vi "mainDebug.vi"() -> ()   [LabVIEW 2024]
doc: "Main VI for FLS imaging system."
uses:
  SubVI/DigitizerConfiguration/FLImDAQ.ctl
  <instrlib>/niScope/Controls/niScope trigger source.ctl
  SubVI/LabJack/LJ Pin Setting.ctl
  ConfigFiles/AimingBeamVideoConfig.ctl
  <vilib>/Utility/error.llb/DialogType.ctl
  SubVI/GlobalVariables.vi
  <vilib>/Instr/_visa.llb/VISA Configure Serial Port (Instr).vi
  <userlib>/_OpenG.lib/file/file.llb/openg_file.lvlib
  <userlib>/_OpenG.lib/time/time.llb/openg_time.lvlib
  <vilib>/Utility/miscctls.llb/LVPointTypeDef.ctl
panel:
  out "TCP wait time(ms)":u32
  in  "error (stop LT loop)":errorcluster
  out "Dummy LT Waveform":dbl(graph)
  in  "DeconChannel":i8=1 min=1 max=3 step=1
  out "Visualization PC video source":T1
  in  "Video Display":bool
  out "ML?":bool
  out "Sync Success?":bool
  out "Disclamer":picture
  out "Calibration #":i8
  out "BG #":i8
  in  "TCP Connect":bool
  out "Help":string
  in  "355nm Laser toggle":bool caption="355nm 460Hz"
  in  "Aiming beam toggle":bool caption="445nm 15Hz 15mA"
  out "Run #":i8
  in  "StopButton":bool caption="Stop"
  out "Aquisition Status:":bool
  in  "StartButton":bool caption="Start"
  in  "Video Source":enum32{"Camera", "FrameGrabber"}(radio)
  out "Case #":string
  out "System Hardware Connection Status":T2
  in  "Tab Control":T3(tab)
  out "Communication loop(ms)":u32
  out "laser EM lamp V":dbl format="%0.6f"
  in  "Show BG":bool
  out "LJ Pinout":T4={"Ch1 Bias"="DAC0", "Ch2 Bias"="DAC1", "Ch3 Bias"="DAC2", "Ch4 Bias"="DAC0", "355 PWM"="FIO0", "AimingBeam PWM"="FIO2", "Laser Ready"="FIO3", "Interlock"="FIO1", "Laser Start/Stop"="FIO1", "Red LED"="FIO1", "Green LED"="DIO3", "Foot Pedal"="DIO15"}
  out "FLImDAQ":T5={"Digitizer 1"="", "Digitizer 2"="", "Channel"=enum."Channel 0", "trigger source"="VAL_EXTERNAL", "trigger level"=0.5, "trigger delay"=1.35e-07, "min sample rate"=12500000000.0, "min record length"=2500, "vertical range"=1.0, "vertical offset"=-0.25, "Waveform to Avg"=2000} caption="FLIm DAQ Configuration" {"trigger delay" format="%^#.4e"; "trigger level" min=0.0 max=3.5 step=0.5 format="%.2f"; "vertical offset" format="%.4f"; "vertical range" format="%.2f"; "min sample rate" format="%#.2p"}
  in  "Sys Reconfig":bool
  out "data out(communcation loop)":string
  out "Laser Rep Rate":dbl
  out "State log":string
  in  "Quit":bool
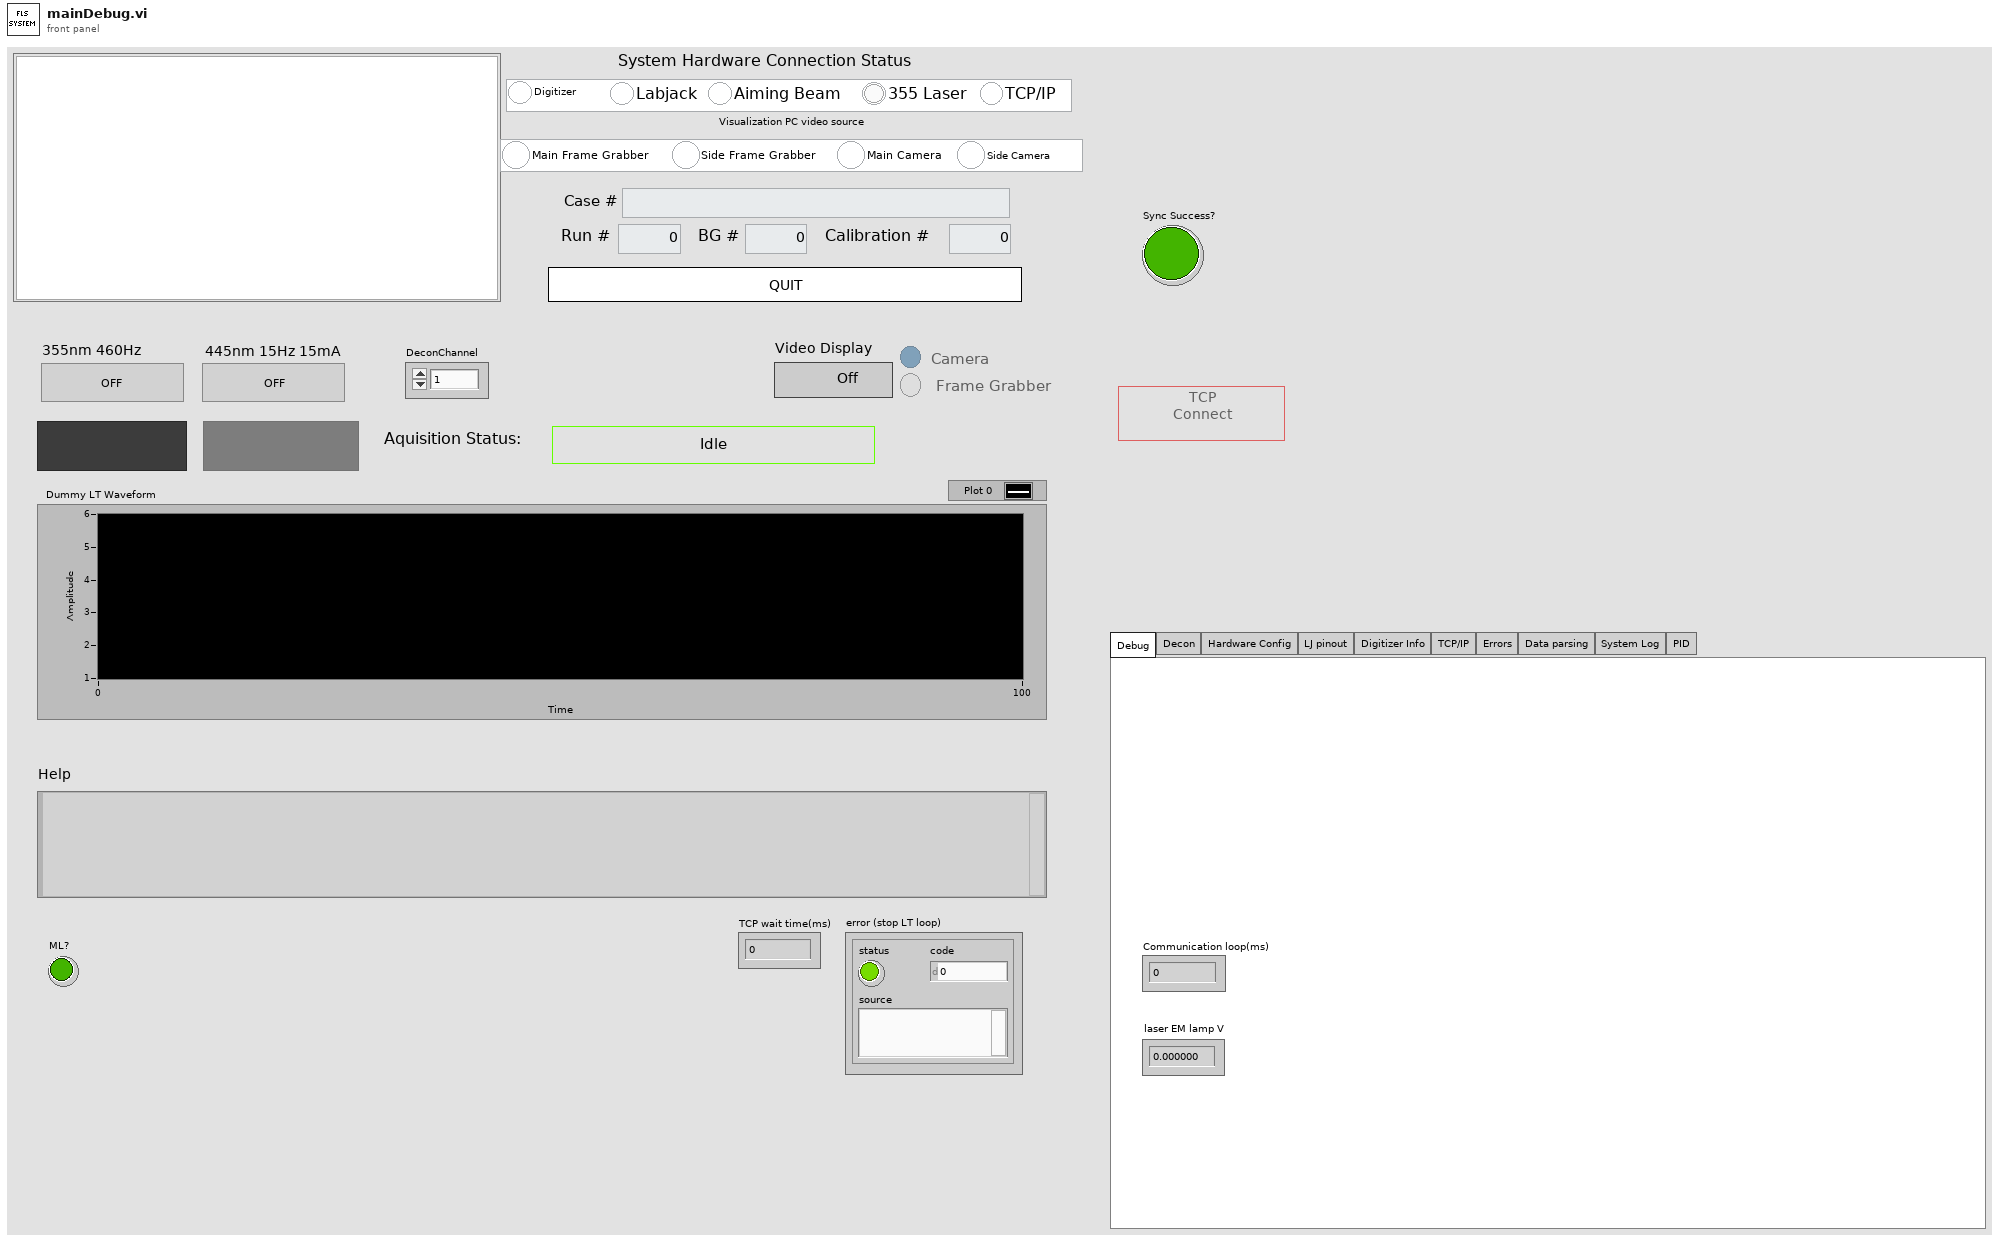
[diagram p1: front panel]
types:
  T1 = cluster{"Main Frame Grabber":bool, "Side Frame Grabber":bool, "Main Camera":bool, "Side Camera":bool}
  T2 = cluster{"Digitizer":bool, "Labjack":bool, "Aiming Beam":bool, "355 Laser":bool, "TCP/IP":bool}
  T3 = enum32{"Debug", "Decon", "Hardware Config", "LJ pinout", "Digitizer Info", "TCP/IP", "Errors", "Data parsing", "System Log", "PID"}
  T4 = typedef "LJ Pin Setting.ctl" = cluster{"Ch1 Bias":string, "Ch2 Bias":string, "Ch3 Bias":string, "Ch4 Bias":string, "355 PWM":string, "AimingBeam PWM":string, "Laser Ready":string, "Interlock":string, "Laser Start/Stop":string, "Red LED":string, "Green LED":string, "Foot Pedal":string}
  T5 = typedef "FLImDAQ.ctl" = cluster{"Digitizer 1":refnum<k15>, "Digitizer 2":refnum<k15>, "Channel":enum16{"Channel 0", "Channel 1", "Channel 0&1"}, "trigger source":T6, "trigger level":dbl, "trigger delay":dbl, "min sample rate":dbl, "min record length":i32, "vertical range":dbl, "vertical offset":dbl, "Waveform to Avg":i16}
  T6 = typedef "niScope trigger source.ctl" = string
  T7 = cluster{"remote start event":refnum<user-event>, "remote stop  event":refnum<user-event>}
  T8 = enum8{"Enabled", "Disabled", "Disabled and Grayed Out"}
  T9 = enum16{"open", "replace", "create", "open or create", "replace or create", "replace or create with confirmation"}
  T10 = enum32{"Invalid", "Standard", "Closed", "Hidden", "Minimized", "Maximized"}
  T11 = enum32{"invalid app kind", "Development System", "Run Time System", "Student Edition", "Embedded LabVIEW", "Evaluation", "Custom"}
  T12 = enum32{"Bad", "Idle", "Run top level", "Running"}
  T13 = enum16{"Standard", "Buffered", "CRLF", "Immediate"}
  T14 = typedef "AimingBeamVideoConfig.ctl" = cluster{"DeCon Channel":enum16{"1", "2", "3"}, "Scale Bar":bool, "Scale Low":dbl, "Scale High":dbl, "ANSI":dbl, "Radius":dbl, "3D?":bool, "Firefly?":bool, "Pentero?":bool}
  T15 = cluster{"Core":cluster{"Current VI Reference":refnum<vi>, "Close Panel on Exit?":bool}, "SysConfigCluster":cluster{"Ch1Enable?":bool, "Ch2Enable?":bool, "Ch3Enable?":bool, "Ch1AutoGain?":bool, "Ch2AutoGain?":bool, "Ch3AutoGain?":bool, "AimingBeamEnable?":bool}, "System Status":cluster{"Digitizer":bool, "Labjack":bool, "Aiming Beam":bool, "355 Laser":bool, "TCP/IP":bool}, "IDs":cluster{"RunID":i8, "BG ID":i8, "Cali ID":i8}, "CaseID":string, "DefaultPath":path, "Pathes":cluster{"DataPath":path, "BG Path":path, "iRFPath":path, "CaliPath":path}, "FLImDAQ":cluster{"resource name":refnum<k15>, "resource name 2":refnum<k15>, "Channel":enum16{"Channel 0", "Channel 1", "Channel 0&1"}, "trigger source":T6, "trigger level":dbl, "trigger delay":dbl, "min sample rate":dbl, "min record length":i32, "vertical range":dbl, "vertical offset":dbl, "Waveform to Avg":i32}, "SysRunning?":bool, "AB Cluster":cluster{"Aiming Beam COM Port":refnum<visa-resource-name>, "Min Current":dbl, "Max Current":dbl, "Default Current":dbl, "Freq":i32}, "LJ Pinout":T4, "355 PWM setting":cluster{"DIO_EF_CLOCK1_DIVISOR":i16, "DIO_EF_CLOCK1_ROLL_VALUE":i32, "DIO#_EF_INDEX":i16, "DIO#_EF_OPTIONS":i16, "DIO#_EF_CONFIG_A":i32}, "AB PWM setting":cluster{"DIO_EF_CLOCK1_DIVISOR":i16, "DIO_EF_CLOCK1_ROLL_VALUE":i32, "DIO#_EF_INDEX":i16, "DIO#_EF_OPTIONS":i16, "DIO#_EF_CONFIG_A":i32}, "Last Trigger":u32, "niTClk sessions":refnum<k20>[], "Laser start tic":u32, "TCP attempt count":i32, "Ch1Data":dbl[][], "Ch2Data":dbl[][], "Ch3Data":dbl[][], "V1":dbl[], "V2":dbl[], "V3":dbl[], "SlowTimer":u32, "FastTimer":u32, "listener ID":refnum<k5>, "TempPath":path, "LED vi reference":refnum<vi>, "Aquisition Timer":u32, "APDSerialNum":cluster{"Ch1APDSerial#":string, "Ch2APDSerial#":string, "Ch3APDSerial#":string}, "VideoConfig":T14, "CaliPath":path, "LED vi ref open?":bool, "video source":cluster{"Main Frame Grabber":bool, "Side Frame Grabber":bool, "Main Camera":bool, "Side Camera":bool}, "bothVidSourceAvail":bool}
  T16 = cluster{"Ch1APDSerial#":string, "Ch2APDSerial#":string, "Ch3APDSerial#":string}
  T17 = cluster{"DataPath":path, "BG Path":path, "iRFPath":path, "CaliPath":path}
  T18 = cluster{"DIO_EF_CLOCK1_DIVISOR":i16, "DIO_EF_CLOCK1_ROLL_VALUE":i32, "DIO#_EF_INDEX":i16, "DIO#_EF_OPTIONS":i16, "DIO#_EF_CONFIG_A":i32}
  T19 = cluster{"Aiming Beam COM Port":refnum<visa-resource-name>, "Min Current":dbl, "Max Current":dbl, "Default Current":dbl, "Freq":i32}
  T20 = cluster{"resource name":refnum<k15>, "resource name 2":refnum<k15>, "Channel":enum16{"Channel 0", "Channel 1", "Channel 0&1"}, "trigger source":T6, "trigger level":dbl, "trigger delay":dbl, "min sample rate":dbl, "min record length":i32, "vertical range":dbl, "vertical offset":dbl, "Waveform to Avg":i32}
  T21 = cluster{"Ch1Enable?":bool, "Ch2Enable?":bool, "Ch3Enable?":bool, "Ch1AutoGain?":bool, "Ch2AutoGain?":bool, "Ch3AutoGain?":bool, "AimingBeamEnable?":bool}
  T22 = cluster{"Current VI Reference":refnum<vi>, "Close Panel on Exit?":bool}
  T23 = typedef "DialogType.ctl" = u16
  T24 = typedef "LJ PWM Setting.ctl" = cluster{"DIO_EF_CLOCK1_DIVISOR":i16, "DIO_EF_CLOCK1_ROLL_VALUE":i32, "DIO#_EF_INDEX":i16, "DIO#_EF_OPTIONS":i16, "DIO#_EF_CONFIG_A":i32}
  T25 = typedef "AimingBeam.ctl" = cluster{"Aiming Beam COM Port":refnum<visa-resource-name>, "Min Current":dbl, "Max Current":dbl, "Default Current":dbl, "Frequency(Hz)":u32}
  T26 = typedef "LVBoundsTypeDef.ctl" = cluster{"Width":u32, "Height":u32}
  T27 = typedef "imagedata.ctl" = cluster{"image type":i32, "image depth":i32, "image":u8[], "mask":u8[], "colors":u32[], "Rectangle":cluster{"left":i16, "top":i16, "right":i16, "bottom":i16}}
  T28 = typedef "LVPointTypeDef.ctl" = cluster{"Horizontal":i16, "Vertical":i16}
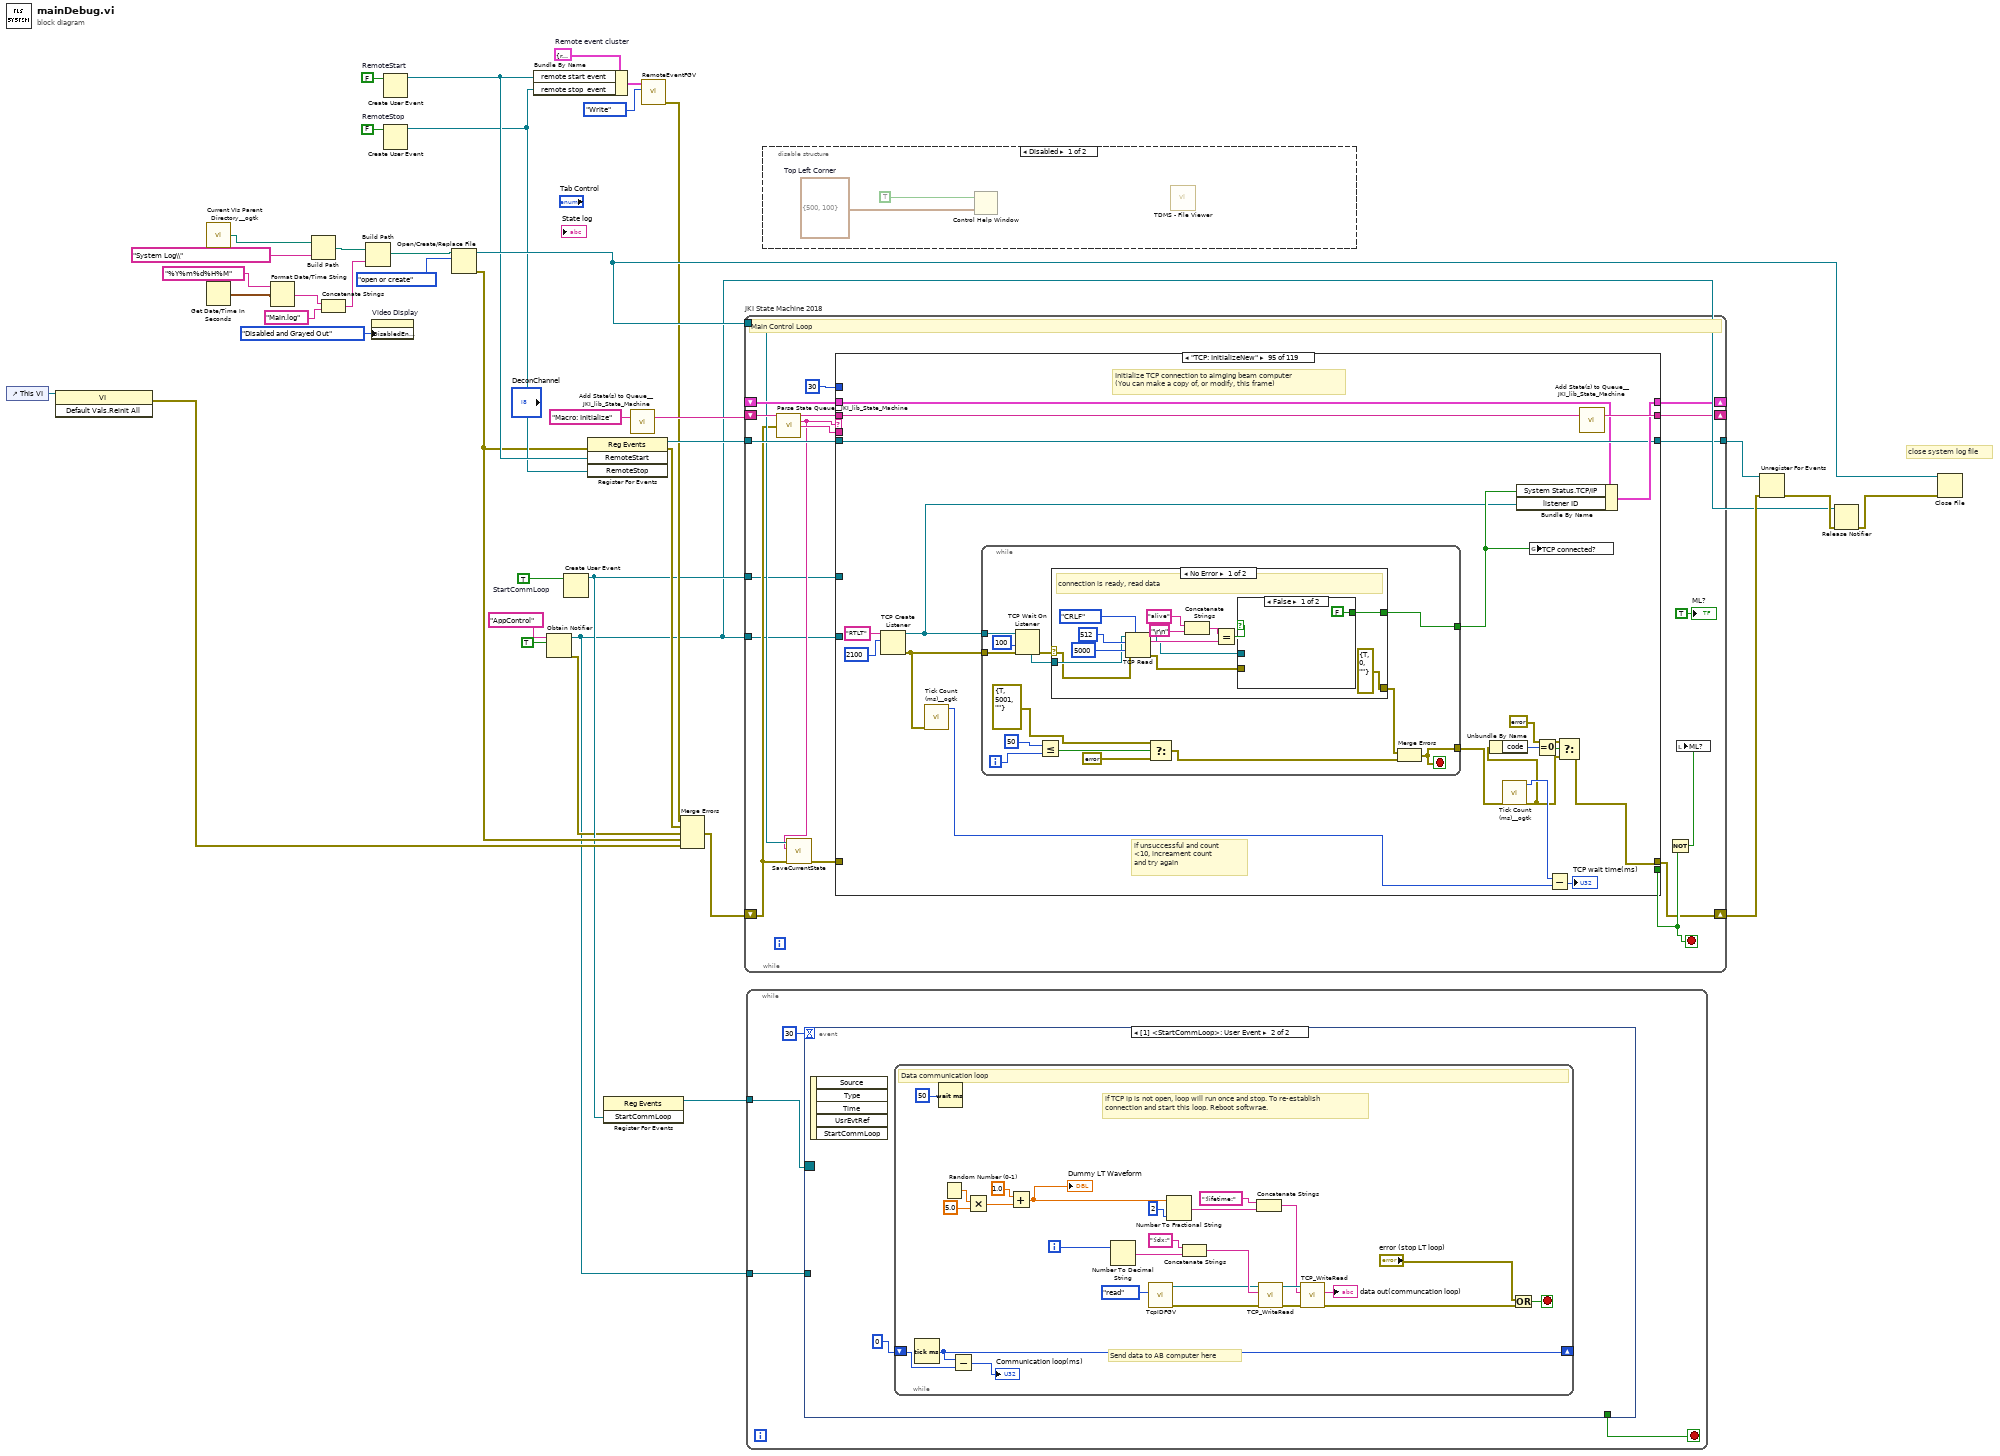
[diagram p0: block diagram]
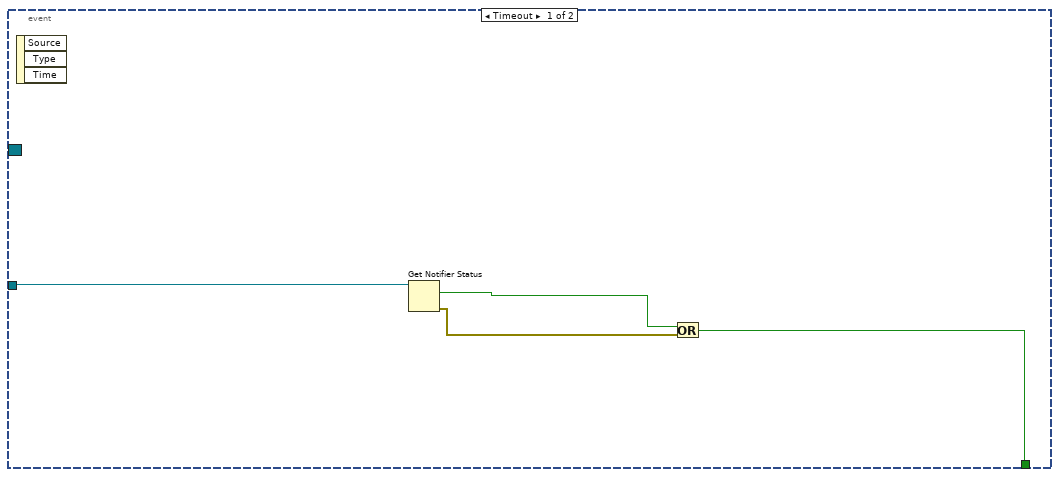
[diagram p2: hidden frame]
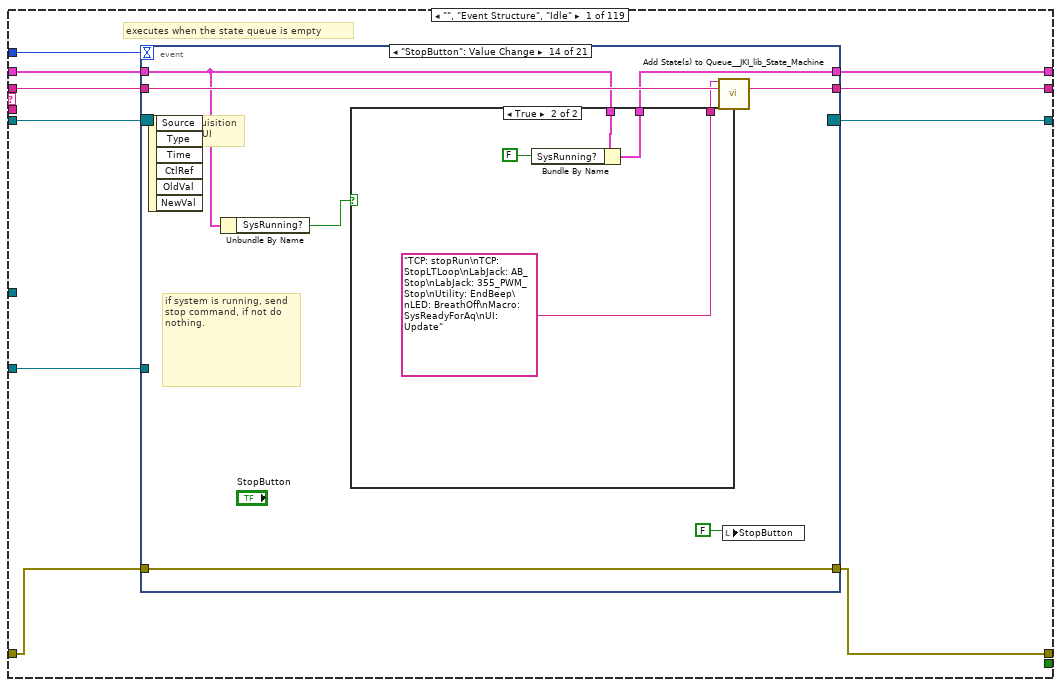
[diagram p3: hidden frame]
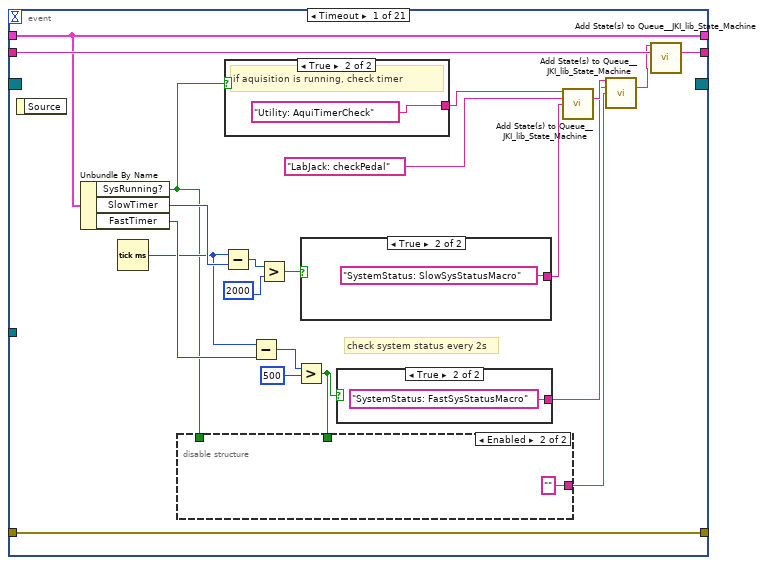
[diagram p4: hidden frame]
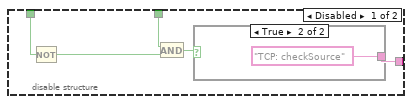
[diagram p5: hidden frame]
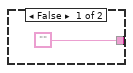
[diagram p6: hidden frame]
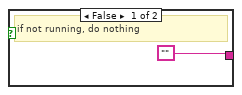
[diagram p7: hidden frame]
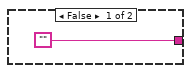
[diagram p8: hidden frame]
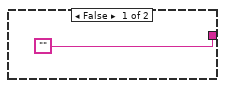
[diagram p9: hidden frame]
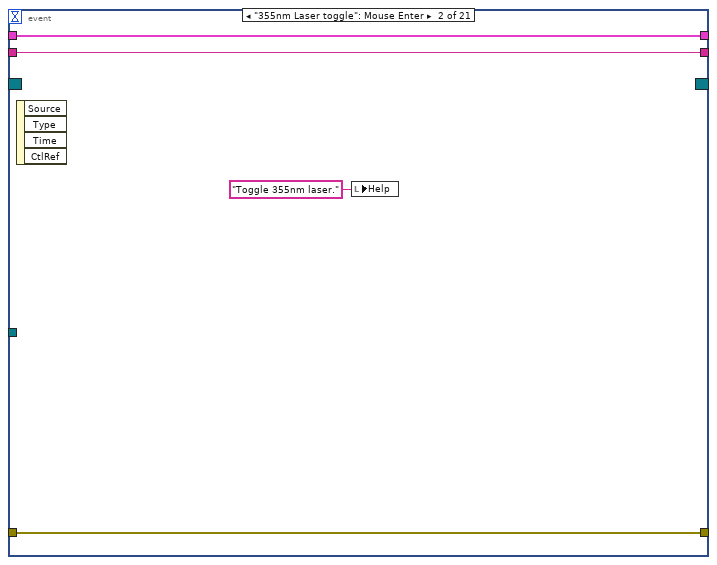
[diagram p10: hidden frame]
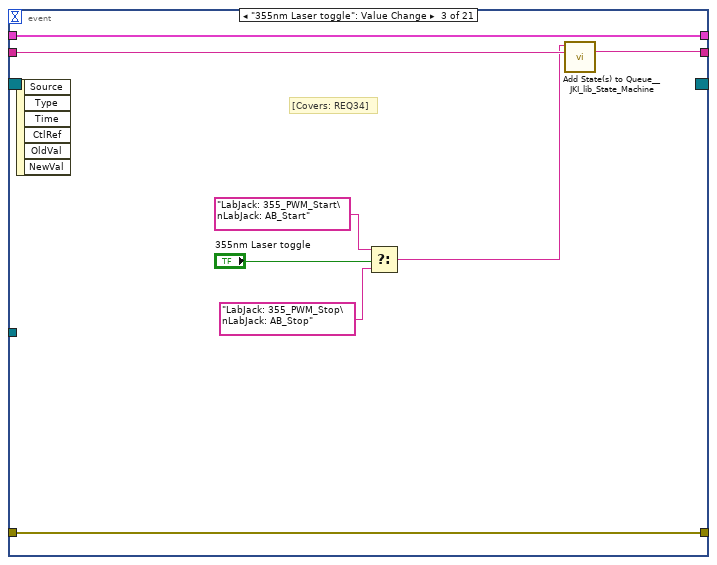
[diagram p11: hidden frame]
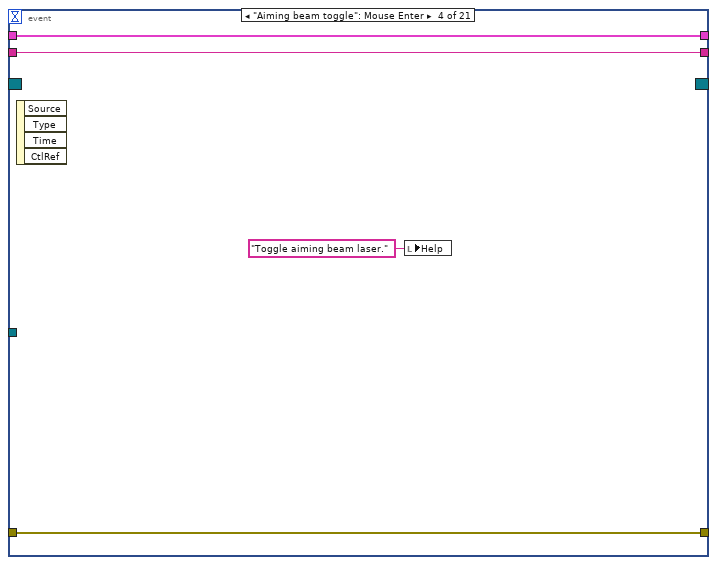
[diagram p12: hidden frame]
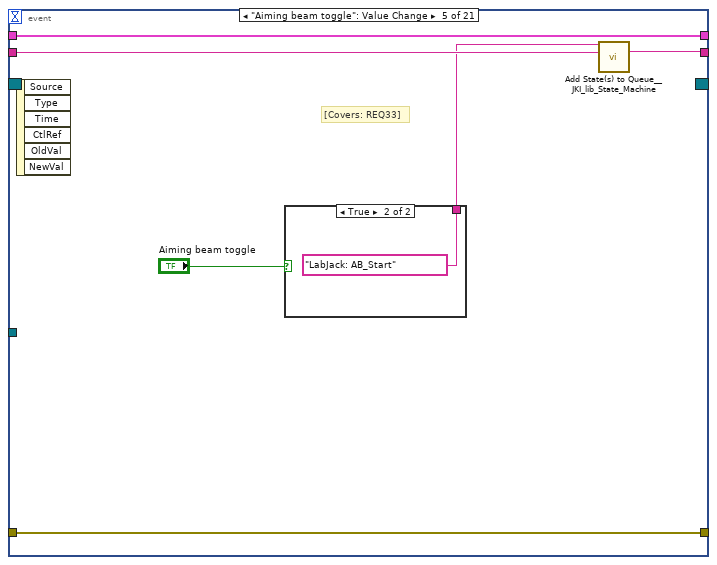
[diagram p13: hidden frame]
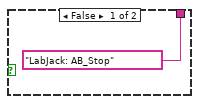
[diagram p14: hidden frame]
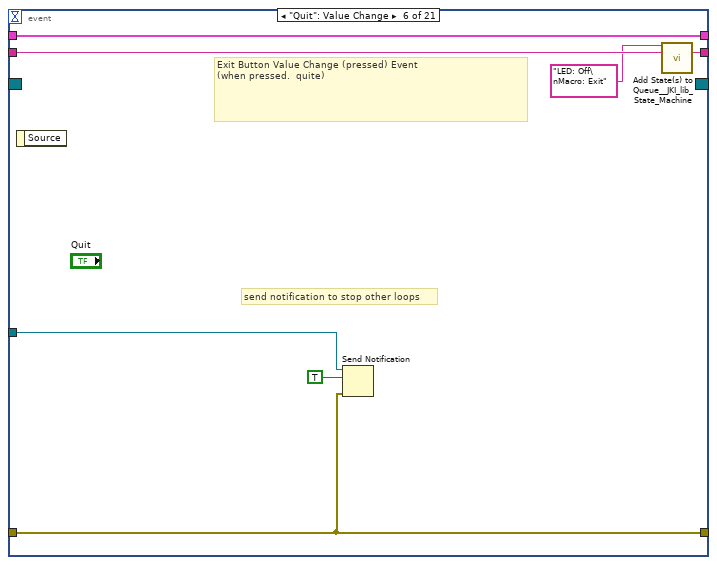
[diagram p15: hidden frame]
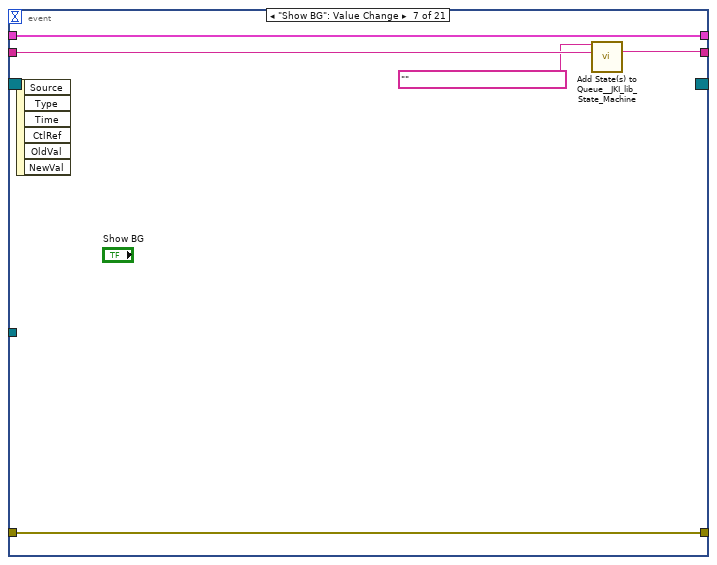
[diagram p16: hidden frame]
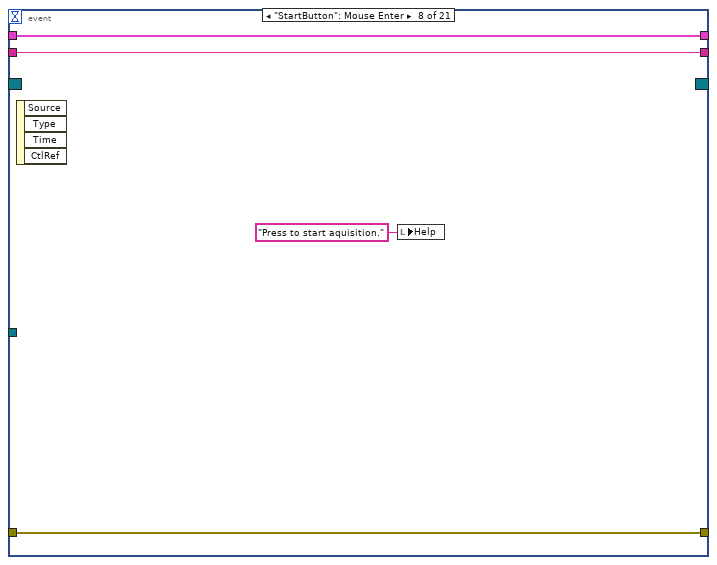
[diagram p17: hidden frame]
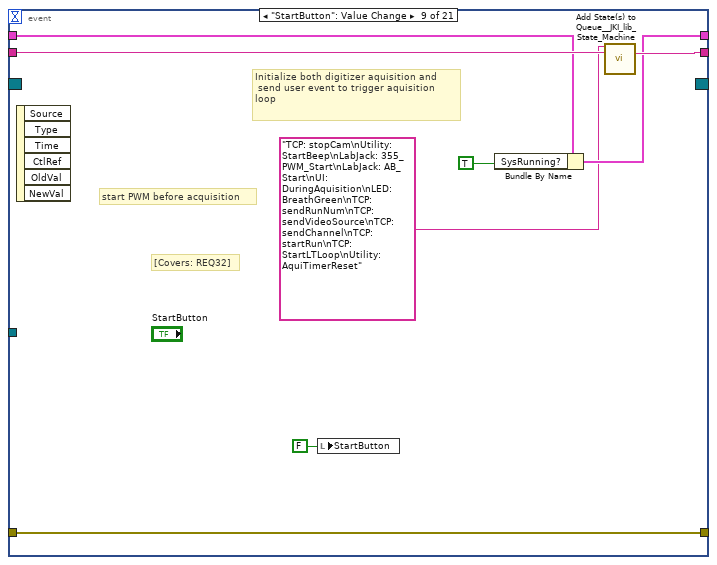
[diagram p18: hidden frame]
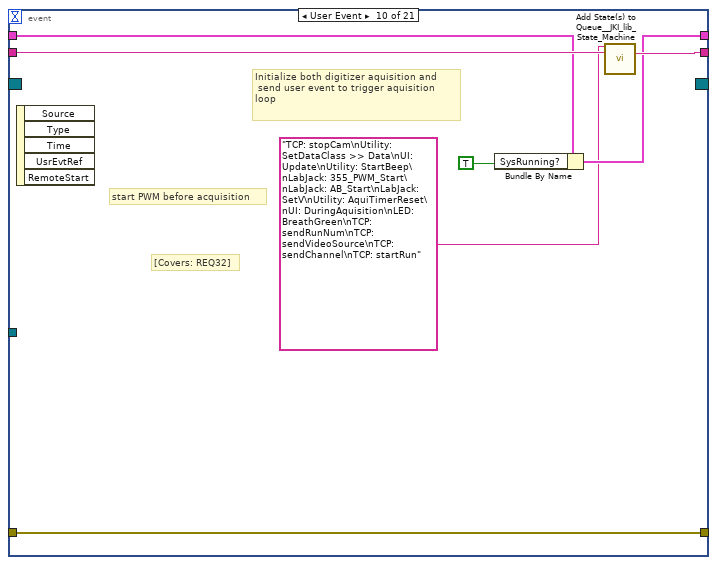
[diagram p19: hidden frame]
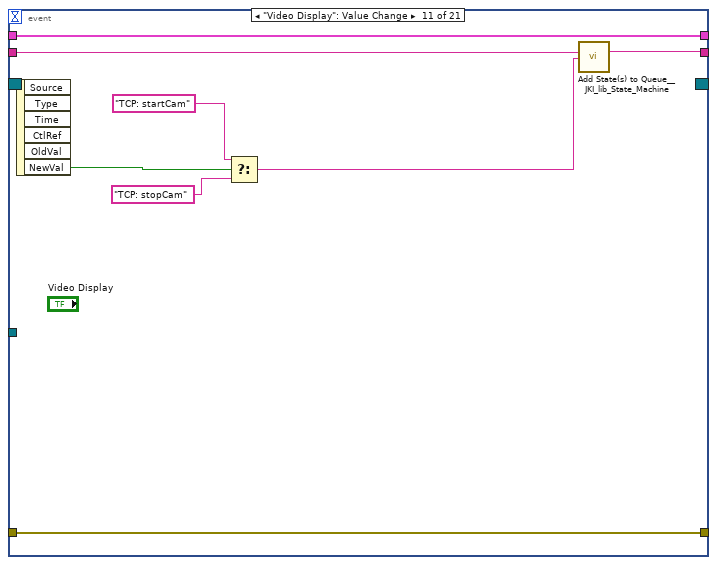
[diagram p20: hidden frame]
diagram:
  w9 = TRUE  # StartCommLoop
  w17 = T7 {"remote start event"=refnum, "remote stop  event"=refnum}  # Remote event cluster
  w20 = FALSE  # RemoteStop
  w21 = FALSE  # RemoteStart
  # "close system log file"
  n1 = control-ref of="This VI"() -> (w37:refnum<vi>)
  n2 = invoke on="Invoke Node" class="VI" method="Default Vals.Reinit All"(reference=w37) -> (error out=w11:errorcluster)  [unwired: 2 in, 2 out]
  n3 = call <userlib>:"Current VIs Parent Directory__ogtk.vi"() -> ("Parent Directory (+ Relative)"=w34:path)  [unwired: 5 in]
  n4 = Get Date/Time In Seconds() -> (seconds since 1Jan1904=w32:timestamp)
  n5 = Format Date/Time String(time format string (%c)="%Y%m%d%H%M", seconds (now)=w32) -> (date/time string=w29:string)  [unwired: 1 in]
  n6 = Build Path(base path=w34, name or relative path="System Log\\") -> (appended path=w25:path)
  n7 = Concatenate Strings(w29, "Main.log" ("string")) -> (w27:string)
  n8 = Build Path(base path=w25, name or relative path=w27) -> (appended path=w30:path)
  n9 = property on="Video Display" class="Bool (strict)"("DisabledEnum"=T8."Disabled and Grayed Out" ("Disabled")) -> ()  [unwired: 2 in, 2 out]
  n10 = Create User Event(user event datatype=w21) -> (user event=w19:refnum<user-event>)  [unwired: 1 in, 1 out]
  n11 = Create User Event(user event datatype=w20) -> (user event=w18:refnum<user-event>)  [unwired: 1 in, 1 out]
  n12 = Open/Create/Replace File(file path (use dialog)=w30, operation (0:open)=T9."open or create") -> (refnum out=w23:refnum<file>, error out=w10:errorcluster)  [unwired: 4 in, 1 out]
  n13 = Bundle By Name(cluster=w17, "remote start event"=w19, "remote stop  event"=w18) -> (w15:T7)
  n14 = Obtain Notifier(name (unnamed)="AppControl", notification data type=TRUE) -> (notifier out=w1:refnum<notifier>, error out=w5:errorcluster)  [unwired: 2 in, 1 out]
  n15 = Create User Event(user event datatype=w9) -> (user event=w8:refnum<user-event>)  [unwired: 1 in, 1 out]
  n16 = register-events(error in=w10, w19, w18) -> (reference out=w36:refnum<event-registration>, error out=w14:errorcluster)  [unwired: 1 in]
  n17 = register-events(w8) -> (reference out=w7:refnum<event-registration>)  [unwired: 2 in, 1 out]
  n18 = call <vilib>:"Add State(s) to Queue__JKI_lib_State_Machine.vi"("State(s) in (\"\")"="Macro: Initialize") -> ("States Out"=w39:string)  [unwired: 14 in]
  n19 = call "RemoteEventFGV.vi"("Operation (Read)"=enum16{"Read", "Write"}."Write", "Remote Event in"=w15) -> ("Error Out"=w12:errorcluster)  [unwired: 8 in, 1 out]
  n20 = Merge Errors(w12, w14, w5, w10, w11) -> (w24:errorcluster)
  n21 = while "JKI State Machine 2018" {
    shift-right: [w54] -> _
    shift-left: _ -> [w53]
    shift-right: [w42] -> w13
    shift-left: w24 -> [w44]
    shift-right: [w55] -> _
    shift-left: w39 -> [w56]
    tunnel: w36 -> [w51]
    tunnel: [w50] -> w35
    tunnel: w23 -> [w46]
    tunnel: w8 -> [w41]
    tunnel: w1 -> [w40]
    stop <- w49 stop-if-true
    # "Main Control Loop"
    n22 = call <vilib>:"Parse State Queue__JKI_lib_State_Machine.vi"("State Queue"=w56, "Error In (no error)"=w44) -> ("Remaining States"=w58:string, "Current State"=w45:string, "Arguments"=w57:string)  [unwired: 11 in]
    n23 = call "SaveCurrentState.vi"("error in (no error)"=w44, "Current State"=w45, "Byte Stream File in"=w46) -> ("error out"=w43:errorcluster)  [unwired: 8 in]
    n24 = case shown="\"TCP: InitializeNew\"" w45 {
      selector: w45 -> [_ _ _ _ _ _ _ _ _ _ w358 _ _ _ _ _ _ _ _ _ _ _ _ _ _ _ _ _ _ _ _ _ _ _ _ _ _ _ _ _ _ _ _ _ _ _ _ _ _ _ _ _ _ _ _ _ _ _ _ _ _ _ _ _ _ _ _ _ _ _ _ _ _ _ _ _ _ _ _ _ _ _ _ _ _ _ _ _ _ _ _ _ _ _ _ _ _ _ _ _ _ _ _ _ _ _ _ _ _ _ _ _ _ _ _ _ _ _ _]
      tunnel: w58 -> [w68 w248 w257 w263 w269 w291 w304 w344 w351 w356 w362 w389 w397 w420 w425 w432 w445 w464 w492 w520 w556 w568 w597 w621 w633 w668 w679 w685 w696 w708 w739 w752 w766 w781 w800 w835 w840 w854 w864 w880 w892 w904 w932 w947 w952 w960 w968 w977 w986 w991 w1007 w1027 w1038 w1060 w1075 w1080 w1088 w1096 w1101 w1107 w1125 w1134 w1141 w1147 w1156 w1172 w1177 w1184 w1196 w1266 w1278 w1287 w1304 w1313 w1336 w1353 w1364 w1377 w1402 w1425 w1431 w1447 w1469 w1477 w1483 w1488 w1495 w1507 w1516 w1521 w1535 w1540 w1545 w1550 w1569 w1620 w1666 w1711 w1722 w1740 w1760 w1774 w1787 w1795 w1812 w1834 w1858 w1877 w1895 w1913 w1931 w1945 w1959 w1978 w1992 w2007 w2013 w2021 w2036]
      tunnel: w57 -> [_ _ _ _ _ _ _ _ _ _ _ _ _ _ _ _ _ _ _ _ _ _ _ _ _ _ _ _ _ w706 _ _ _ _ _ _ _ _ _ _ _ _ _ _ _ _ _ _ _ _ _ _ _ _ _ _ _ _ _ _ _ _ _ _ _ _ _ w1179 w1190 _ _ _ _ w1310 _ _ _ _ _ w1421 _ _ _ _ _ _ _ _ _ _ w1531 _ _ _ _ _ _ _ _ _ _ _ _ _ _ _ _ _ _ _ _ _ _ _ _ _ _ _ _]
      tunnel: w53 -> [w66 w245 w253 w260 w266 w288 w301 _ w346 w353 w360 w382 w394 w418 w422 w428 w433 w454 w484 w512 w553 w557 w586 w611 w626 w647 w677 w682 w689 w704 w722 w747 w758 w776 w793 w818 w837 w850 w858 w877 w889 w901 w920 w936 w949 w954 w961 w973 w982 w988 w994 w1022 w1028 w1057 w1068 w1077 w1081 w1089 w1098 w1105 w1122 w1128 w1139 w1144 w1150 w1169 w1174 w1182 w1192 w1263 w1268 w1281 w1302 w1311 w1326 w1350 w1361 w1371 w1395 w1422 w1428 w1440 w1465 w1474 w1480 w1485 w1489 w1503 w1513 w1518 w1528 w1537 w1542 w1547 w1563 w1614 w1662 w1708 w1718 w1735 w1755 w1769 w1783 w1789 w1807 w1829 w1853 w1872 w1890 w1908 w1926 w1940 w1954 w1973 w1987 w2005 w2010 w2016 w2033]
      tunnel: [w61 w246 w255 w261 w267 w289 w302 w342 w347 w354 w364 w386 errorcluster {"status"=FALSE, "code"=0, "source"=""} ("error out") w417 w423 w430 w443 w462 w476 w499 w554 w560 w584 w607 w625 w635 w671 w683 w694 w698 w713 w742 w754 w772 w792 w809 w838 w842 w860 w875 w887 w899 w922 w937 w950 w958 w966 w970 w979 w989 w1002 w1021 w1032 w1050 w1072 w1078 w1086 w1094 w1099 w1104 w1123 w1132 w1138 w1145 w1153 w1170 w1175 w1180 w1193 w1264 w1272 w1284 w1294 w1307 w1327 w1351 w1360 w1373 w1397 w1423 w1429 w1437 w1459 w1475 w1481 w1486 w1493 w1505 w1514 w1519 w1533 w1538 w1543 w1548 w1558 w1615 w1663 w1709 w1717 w1737 w1757 w1771 w1785 w1791 w1809 w1831 w1855 w1874 w1892 w1910 w1928 w1942 w1956 w1975 w1989 w2001 w2011 w2017 w2034] -> w42
      tunnel: w43 -> [w65 w246 w255 w261 w267 w289 w302 w342 w348 w354 w363 w386 w390 w417 w423 w430 w443 w462 w475 w511 w554 w559 w585 w610 w631 w640 w670 w683 w691 w701 w712 w741 w757 w771 w791 w808 w838 w848 w861 w874 w886 w898 w921 w938 w950 w958 w966 w969 w978 w989 w1001 w1020 w1031 w1056 w1071 w1078 w1086 w1094 w1099 w1104 w1123 w1132 w1138 w1145 w1153 w1170 w1175 w1181 w1194 w1264 w1273 w1283 w1290 w1306 w1328 w1351 w1360 w1368 w1400 w1423 w1429 w1442 w1458 w1475 w1481 w1486 w1493 w1505 w1514 w1519 w1533 w1538 w1543 w1548 _ w1616 w1663 w1709 w1716 w1736 w1756 w1770 w1785 w1790 w1808 w1830 w1854 w1873 w1891 w1909 w1927 w1941 w1955 w1974 w1988 w2000 w2011 w2015 w2034]
      tunnel: [w67 w247 w256 w262 w268 w290 w303 w343 w350 w355 w361 w388 w396 w419 w424 w431 w444 w463 w491 w519 w555 w567 w596 w620 w632 w667 w678 w684 w695 w707 w738 w751 w765 w780 w799 w834 w839 w853 w863 w879 w891 w903 w931 w946 w951 w959 w967 w976 w985 w990 w1006 w1026 w1037 w1059 w1074 w1079 w1087 w1095 w1100 w1106 w1124 w1133 w1140 w1146 w1155 w1171 w1176 w1183 w1195 w1265 w1277 w1286 w1303 w1312 w1335 w1352 w1363 w1376 w1401 w1424 w1430 w1446 w1468 w1476 w1482 w1487 w1494 w1506 w1515 w1520 w1534 w1539 w1544 w1549 w1568 w1619 w1665 w1710 w1721 w1739 w1759 w1773 w1786 w1794 w1811 w1833 w1857 w1876 w1894 w1912 w1930 w1944 w1958 w1977 w1991 w2006 w2012 w2020 w2035] -> w55
      tunnel: [_ _ _ _ _ _ _ _ _ _ _ _ _ TRUE _ _ _ _ _ _ _ _ _ _ _ _ _ _ _ _ _ _ _ _ _ _ _ _ _ _ _ _ _ _ _ _ _ _ _ _ _ _ _ _ _ _ _ _ _ _ _ _ _ _ _ _ _ _ _ _ _ _ _ _ _ _ _ _ _ _ _ _ _ _ _ _ _ _ _ _ _ _ _ _ _ _ _ _ _ _ _ _ _ _ _ _ _ _ _ _ _ _ _ _ _ _ _ _ _] -> w49
      tunnel: [w64 w245 w253 w260 w266 w288 w301 w317 w346 w353 w360 w387 w394 w418 w422 w429 w434 w455 w485 w513 w553 w558 w586 w611 w630 w647 w677 w682 w692 w704 w722 w747 w758 w776 w793 w818 w837 w851 w858 w877 w889 w901 w920 w936 w949 w955 w962 w974 w983 w988 w1000 w1009 w1033 w1058 w1069 w1077 w1082 w1090 w1098 w1105 w1122 w1128 w1139 w1144 w1150 w1169 w1174 w1182 w1192 w1263 w1269 w1282 w1302 w1311 w1326 w1350 w1361 w1372 w1396 w1422 w1428 w1441 w1465 w1474 w1480 w1485 w1490 w1503 w1513 w1518 w1528 w1537 w1542 w1547 w1567 w1613 w1662 w1708 w1718 w1735 w1755 w1769 w1783 w1789 w1807 w1829 w1853 w1872 w1890 w1908 w1926 w1940 w1954 w1973 w1987 w2005 w2010 w2018 w2033] -> w54
      tunnel: 30 ("Timeout") -> [w63 _ _ _ _ _ _ _ _ _ _ _ _ _ _ _ _ _ _ _ _ _ _ _ _ _ _ _ _ _ _ _ _ _ _ _ _ _ _ _ _ _ _ _ _ _ _ _ _ _ _ _ _ _ _ _ _ _ _ _ _ _ _ _ _ _ _ _ _ _ _ _ _ _ _ _ _ _ _ _ _ _ _ _ _ _ _ _ _ _ _ _ _ _ _ _ _ _ _ _ _ _ _ _ _ _ _ _ _ _ _ _ _ _ _ _ _ _ _]
      tunnel: w51 -> [w60 w244 w254 w259 w265 w280 w300 w327 w345 w352 w357 w374 w393 w416 w421 w427 w442 w461 w490 w510 w552 w566 w595 w619 w624 w666 w669 w681 w688 w697 w709 w740 w756 w770 w790 w805 w836 w852 w862 w878 w890 w902 w930 w933 w948 w957 w965 w972 w981 w987 w995 w1010 w1029 w1055 w1073 w1076 w1084 w1092 w1097 w1103 w1121 w1131 w1137 w1143 w1152 w1164 w1173 w1178 w1189 w1262 w1267 w1279 w1289 w1305 w1334 w1349 w1362 w1374 w1398 w1418 w1426 w1439 w1467 w1472 w1478 w1484 w1492 w1504 w1512 w1517 w1532 w1536 w1541 w1546 w1566 w1618 w1664 w1705 w1720 w1738 w1758 w1772 w1784 w1793 w1810 w1832 w1856 w1875 w1893 w1911 w1929 w1943 w1957 w1976 w1990 w2004 w2009 w2019 w2032]
      tunnel: [w62 w244 w254 w259 w265 w280 w300 w327 w345 w352 w357 w374 w393 w416 w421 w427 w442 w461 w490 w510 w552 w566 w595 w619 w624 w666 w669 w681 w688 w697 w709 w740 w756 w770 w790 w805 w836 w852 w862 w878 w890 w902 w930 w933 w948 w957 w965 w972 w981 w987 w995 w1010 w1029 w1055 w1073 w1076 w1084 w1092 w1097 w1103 w1121 w1131 w1137 w1143 w1152 w1164 w1173 w1178 w1189 w1262 w1267 w1279 w1289 w1305 w1334 w1349 w1362 w1374 w1398 w1418 w1426 w1439 w1467 w1472 w1478 w1484 w1492 w1504 w1512 w1517 w1532 w1536 w1541 w1546 w1566 w1618 w1664 w1705 w1720 w1738 w1758 w1772 w1784 w1793 w1810 w1832 w1856 w1875 w1893 w1911 w1929 w1943 w1957 w1976 w1990 w2004 w2009 w2019 w2032] -> w50
      tunnel: w41 -> [_ _ _ _ _ _ _ _ _ _ _ _ _ _ _ _ _ _ _ _ _ _ _ _ _ _ _ _ _ _ _ _ _ _ _ _ _ _ _ _ _ _ _ _ _ _ _ _ _ _ _ _ _ _ _ _ _ _ _ _ _ _ _ _ _ _ _ _ _ _ _ _ _ _ _ _ _ _ _ _ _ _ _ _ _ _ _ _ _ _ _ _ _ _ _ _ _ _ _ _ _ _ _ _ _ _ _ _ _ _ _ _ _ _ _ w2003 _ _ _]
      tunnel: w40 -> [w59 _ _ _ _ _ _ _ _ _ _ _ _ _ _ _ _ _ _ _ _ _ _ _ _ _ _ _ _ _ _ _ _ _ _ _ _ _ _ _ _ _ _ _ _ _ _ _ _ _ _ _ _ _ _ _ _ _ _ _ _ _ _ _ _ _ _ _ _ _ _ _ _ _ _ _ _ _ _ _ _ _ _ _ _ _ _ _ _ _ _ _ _ _ _ _ _ _ _ _ _ _ _ _ _ _ _ _ _ _ _ _ _ _ _ _ _ _ _]
      frame "", "Event Structure", "Idle" {
        # "executes when the state queue is empty"
        n25 = event shown="[13] \"StopButton\": Value Change" {
          selector: w60 -> [_ _ _ _ _ _ _ _ _ _ _ _ _ _ _ _ _ _ _ _ _]
          dyn-events: [_ _ _ _ _ _ _ _ _ _ _ _ _ _ _ _ _ _ _ _ _] -> w62
          timeout: w63 -> [_ _ _ _ _ _ _ _ _ _ _ _ _ _ _ _ _ _ _ _ _]
          tunnel: w68 -> [w88 w107 w115 w119 w123 w134 w137 w143 w150 w157 w163 w169 w175 w182 w195 w206 w218 w225 w229 w233 w243]
          tunnel: [w89 w107 w114 w119 w122 w133 w136 w143 w151 w158 w162 w168 w175 w183 w196 w206 w219 w225 w229 w232 w242] -> w67
          tunnel: w66 -> [w72 w105 w109 w117 w124 w131 w138 w141 w146 w153 w165 w170 w173 w177 w190 w204 w214 w223 w227 w234 w240]
          tunnel: [w87 w106 w110 w118 w125 w128 w139 w142 w147 w154 w166 w171 w174 w181 w194 w205 w215 w224 w228 w235 w241] -> w61
          tunnel: w65 -> [w87 w106 w110 w118 w125 w128 w139 w142 w147 w154 w166 w171 w174 w181 w194 w205 w217 w224 w228 w235 w241]
          tunnel: [w72 w105 w109 w117 w124 w131 w138 w141 w148 w155 w165 w170 w173 w178 w191 w204 w220 w223 w227 w234 w240] -> w64
          tunnel: w59 -> [_ _ _ _ _ w130 _ _ _ _ _ _ _ _ _ _ _ _ _ _ _]
          event Timeout {
            # "check system status every 2s"
            n26 = event-data() -> ()  [unwired: 1 in, 1 out]
            n27 = Unbundle By Name(w72) -> ("SysRunning?"=w70:bool, "SlowTimer"=w86:u32, "FastTimer"=w80:u32)
            n28 = Tick Count (ms)() -> (millisecond timer value=w73:u32)
            n29 = Subtract(x=w73, y=w86) -> (x-y=w83:u32)
            n30 = case shown="True" w70 {
              tunnel: ["" "Utility: AquiTimerCheck" ("State(s) in Front (\"\")")] -> w78
              frame False {
                # "if not running, do nothing"
              }
              frame True {
                # "if aquisition is running, check timer"
              }
            }
            n31 = Subtract(x=w73, y=w80) -> (x-y=w81:u32)
            n32 = Greater?(x=w83, y=u32 2000) -> (0:w84:bool)
            n33 = Greater?(x=w81, y=u32 500) -> (0:w71:bool)
            n34 = disable-structure shown="Enabled" {
              disable-tunnel: w71 -> [w94 _]
              disable-tunnel: w70 -> [w93 _]
              disable-tunnel: [w90 "" ("State(s) at Back (\"\")")] -> w69
              frame Disabled {
                n35 = Not(x=w93) -> (.not. x?=w92:bool)
                n36 = And(x=w94, y=w92) -> (x .and. y?=w91:bool)
                n37 = case shown="True" w91 {
                  tunnel: ["" ("Empty String Constant") "TCP: checkSource" ("State(s) in Front (\"\")")] -> w90
                  frame False {
                  }
                  frame True {
                  }
                }
              }
              frame Enabled {
              }
            }
            n38 = case shown="True" w84 {
              tunnel: ["" ("Empty String Constant") "SystemStatus: SlowSysStatusMacro" ("State(s) in Front (\"\")")] -> w76
              frame False {
              }
              frame True {
              }
            }
            n39 = case shown="True" w71 {
              tunnel: ["" ("Empty String Constant") "SystemStatus: FastSysStatusMacro" ("State(s) in Front (\"\")")] -> w74
              frame False {
              }
              frame True {
              }
            }
            n40 = call <vilib>:"Add State(s) to Queue__JKI_lib_State_Machine.vi"("State(s) in Front (\"\")"=w78, "State(s) in (\"\")"="LabJack: checkPedal" ("State(s) in Front (\"\")"), "State(s) at Back (\"\")"=w76) -> ("States Out"=w75:string)  [unwired: 12 in]
            n41 = call <vilib>:"Add State(s) to Queue__JKI_lib_State_Machine.vi"("State(s) in Front (\"\")"=w75, "State(s) in (\"\")"=w74, "State(s) at Back (\"\")"=w69) -> ("States Out"=w79:string)  [unwired: 12 in]
            n42 = call <vilib>:"Add State(s) to Queue__JKI_lib_State_Machine.vi"("State(s) in Front (\"\")"=w79, "State(s) in (\"\")"=w88) -> ("States Out"=w89:string)  [unwired: 13 in]
          }
          event "355nm Laser toggle": Mouse Enter {
            n43 = event-data() -> ()  [unwired: 1 in, 4 out]
            n44 = local write "Help"("Toggle 355nm laser." ("Help")) -> ()
          }
          event "355nm Laser toggle": Value Change {
            # "[Covers: REQ34]"
            n45 = event-data() -> ()  [unwired: 1 in, 6 out]
            n46 = Select(t="LabJack: 355_PWM_Start\nLabJack: AB_Start", s="355nm Laser toggle", f="LabJack: 355_PWM_Stop\nLabJack: AB_Stop") -> (s? t:f=w112:string)
            n47 = call <vilib>:"Add State(s) to Queue__JKI_lib_State_Machine.vi"("State(s) in Front (\"\")"=w112, "State(s) in (\"\")"=w115) -> ("States Out"=w114:string)  [unwired: 13 in]
          }
          event "Aiming beam toggle": Mouse Enter {
            n48 = event-data() -> ()  [unwired: 1 in, 4 out]
            n49 = local write "Help"("Toggle aiming beam laser." ("Help")) -> ()
          }
          event "Aiming beam toggle": Value Change {
            # "[Covers: REQ33]"
            n50 = event-data() -> ()  [unwired: 1 in, 6 out]
            n51 = case shown="True" "Aiming beam toggle" {
              tunnel: ["LabJack: AB_Stop" ("State(s) in Front (\"\")") "LabJack: AB_Start" ("State(s) in Front (\"\")")] -> w121
              frame False {
              }
              frame True {
              }
            }
            n52 = call <vilib>:"Add State(s) to Queue__JKI_lib_State_Machine.vi"("State(s) in Front (\"\")"=w121, "State(s) in (\"\")"=w123) -> ("States Out"=w122:string)  [unwired: 13 in]
          }
          event "Quit": Value Change {
            # "send notification to stop other loops"
            # "Exit Button Value Change (pressed) Event\n(when pressed.  quite)"
            n53 = event-data() -> ()  [unwired: 1 in, 1 out]
            n54 = Send Notification(notification=TRUE, notifier=w130, error in (no error)=w128) -> ()  [unwired: 2 out]
            n55 = call <vilib>:"Add State(s) to Queue__JKI_lib_State_Machine.vi"("State(s) in Front (\"\")"="LED: Off\nMacro: Exit", "State(s) in (\"\")"=w134) -> ("States Out"=w133:string)  [unwired: 13 in]
          }
          event "Show BG": Value Change {
            n56 = event-data() -> ()  [unwired: 1 in, 6 out]
            n57 = call <vilib>:"Add State(s) to Queue__JKI_lib_State_Machine.vi"("State(s) in Front (\"\")"="" ("State(s) in Front (\"\")"), "State(s) in (\"\")"=w137) -> ("States Out"=w136:string)  [unwired: 13 in]
          }
          event "StartButton": Mouse Enter {
            n58 = event-data() -> ()  [unwired: 1 in, 4 out]
            n59 = local write "Help"("Press to start aquisition." ("Help")) -> ()
          }
          event "StartButton": Value Change {
            # "[Covers: REQ32]"
            # "start PWM before acquisition"
            # "Initialize both digitizer aquisition and\n send user event to trigger aquisition loop"
            n60 = event-data() -> ()  [unwired: 1 in, 6 out]
            n61 = local write "StartButton"(FALSE ("StartButton")) -> ()
            n62 = Bundle By Name(cluster=w146, "SysRunning?"=TRUE) -> (w148:T15)
            n63 = call <vilib>:"Add State(s) to Queue__JKI_lib_State_Machine.vi"("State(s) in Front (\"\")"="TCP: stopCam\nUtility: StartBeep\nLabJack: 355_PWM_Start\nLabJack: AB_Start\nUI: DuringAquisition\nLED: BreathGreen\nTCP: sendRunNum\nTCP: sendVideoSource\nTCP: sendChannel\nTCP: startRun\nTCP: StartLTLoop\nUtility: AquiTimerReset", "State(s) in (\"\")"=w150) -> ("States Out"=w151:string)  [unwired: 13 in]
          }
          event User Event {
            # "[Covers: REQ32]"
            # "start PWM before acquisition"
            # "Initialize both digitizer aquisition and\n send user event to trigger aquisition loop"
            n64 = event-data() -> ()  [unwired: 1 in, 5 out]
            n65 = Bundle By Name(cluster=w153, "SysRunning?"=TRUE) -> (w155:T15)
            n66 = call <vilib>:"Add State(s) to Queue__JKI_lib_State_Machine.vi"("State(s) in Front (\"\")"="TCP: stopCam\nUtility: SetDataClass >> Data\nUI: Update\nUtility: StartBeep\nLabJack: 355_PWM_Start\nLabJack: AB_Start\nLabJack: SetV\nUtility: AquiTimerReset\nUI: DuringAquisition\nLED: BreathGreen\nTCP: sendRunNum\nTCP: sendVideoSource\nTCP: sendChannel\nTCP: startRun", "State(s) in (\"\")"=w157) -> ("States Out"=w158:string)  [unwired: 13 in]
          }
          event "Video Display": Value Change {
            n67 = event-data() -> ("NewVal"=w164:bool)  [unwired: 1 in, 5 out]
            n68 = Select(t="TCP: startCam", s=w164, f="TCP: stopCam") -> (s? t:f=w161:string)
            n69 = call <vilib>:"Add State(s) to Queue__JKI_lib_State_Machine.vi"("State(s) in (\"\")"=w163, "State(s) at Back (\"\")"=w161) -> ("States Out"=w162:string)  [unwired: 13 in]
          }
          event "Video Source": Value Change {
            n70 = event-data() -> ()  [unwired: 1 in, 6 out]
            n71 = call <vilib>:"Add State(s) to Queue__JKI_lib_State_Machine.vi"("State(s) in Front (\"\")"="TCP: sendVideoSource" ("State(s) in Front (\"\")"), "State(s) in (\"\")"=w169) -> ("States Out"=w168:string)  [unwired: 13 in]
          }
          event "StopButton": Mouse Enter {
            n72 = event-data() -> ()  [unwired: 1 in, 4 out]
            n73 = local write "Help"("Press to stop data aquisition." ("Help")) -> ()
          }
          event "StopButton": Value Change {
            # "if system is running, send stop command, if not do nothing."
            # "stop aquisition\nupdate UI"
            n74 = event-data() -> ()  [unwired: 1 in, 6 out]
            n75 = Unbundle By Name(w177) -> ("SysRunning?"=w179:bool)
            n76 = case shown="True" w179 {
              tunnel: ["" ("Empty String Constant") "TCP: stopRun\nTCP: StopLTLoop\nLabJack: AB_Stop\nLabJack: 355_PWM_Stop\nUtility: EndBeep\nLED: BreathOff\nMacro: SysReadyForAq\nUI: Update"] -> w180
              tunnel: w177 -> [w184 w188]
              tunnel: [w184 w187] -> w178
              frame False {
              }
              frame True {
                n77 = Bundle By Name(cluster=w188, "SysRunning?"=FALSE) -> (w187:T15)
              }
            }
            n78 = call <vilib>:"Add State(s) to Queue__JKI_lib_State_Machine.vi"("State(s) in Front (\"\")"=w180, "State(s) in (\"\")"=w182) -> ("States Out"=w183:string)  [unwired: 13 in]
            n79 = local write "StopButton"(FALSE ("StopButton")) -> ()
          }
          event User Event {
            # "if system is running, send stop command, if not do nothing."
            # "stop aquisition\nupdate UI"
            n80 = event-data() -> ()  [unwired: 1 in, 5 out]
            n81 = Unbundle By Name(w190) -> ("SysRunning?"=w192:bool)
            n82 = case shown="True" w192 {
              tunnel: ["" ("Empty String Constant") "LabJack: AB_Stop\nLabJack: 355_PWM_Stop"] -> w193
              tunnel: w190 -> [w197 w201]
              tunnel: [w197 w200] -> w191
              frame False {
              }
              frame True {
                n83 = Bundle By Name(cluster=w201, "SysRunning?"=FALSE) -> (w200:T15)
              }
            }
            n84 = call <vilib>:"Add State(s) to Queue__JKI_lib_State_Machine.vi"("State(s) in Front (\"\")"=w193, "State(s) in (\"\")"=w195) -> ("States Out"=w196:string)  [unwired: 13 in]
          }
          event "Sys Reconfig": Mouse Enter {
            n85 = event-data() -> ()  [unwired: 1 in, 4 out]
            n86 = local write "Help"("Click to reconfig digitizer settings." ("Help")) -> ()
          }
          event "Sys Reconfig": Value Change {
            # "everytime the user change data aquisition setting, need to reinitilize decon engine and realign iRF.\ncheck whether data length has changed, if changed, reinitialize Decon engine\nreset BG ready, need a new BG"
            # "update DAQ FGV"
            n87 = event-data() -> ()  [unwired: 1 in, 6 out]
            n88 = call "SystemConfigEditorV6.vi"("error in"=w217) -> ("error out"=w216:errorcluster, "FLImDAQ out"=w211:T5)  [unwired: 1 in]
            n89 = Unbundle By Name(w214) -> ("FLImDAQ.min record length"=w213:i32)
            n90 = Unbundle By Name(w211) -> ("min record length"=w212:i32)
            n91 = call "FLImDAQ_FGV.vi"("error in (no error)"=w216, "Operation (Read)"=enum16{"Write", "Read"}."Write" ("Operation"), "Write data"=w211) -> ("error out"=w215:errorcluster, "Read data"=w210:T5)  [unwired: 7 in]
            n92 = Equal?(x=w213, y=w212) -> (x = y?=w209:bool)
            n93 = case shown="False" w209 {
              tunnel: ["UI: Cursor Set >> Busy\nUI: CaliAndiRFNotReady\n/*UI iRF not ready\nUI: Update\nUI: Cursor Set >> Idle" "UI: Cursor Set >> Busy\nUI: Update\nUI: Cursor Set >> Idle"] -> w208
              frame False {
              }
              frame True {
              }
            }
            n94 = Bundle By Name(cluster=w214, "FLImDAQ"=w210) -> (w220:T15)
            n95 = call <vilib>:"Add State(s) to Queue__JKI_lib_State_Machine.vi"("State(s) in Front (\"\")"=w208, "State(s) in (\"\")"=w218) -> ("States Out"=w219:string)  [unwired: 13 in]
          }
          event "System Hardware Connection Status", "StartButton", "StopButton", "355nm Laser toggle", "Aiming beam toggle", "Sys Reconfig": Mouse Leave {
            n96 = event-data() -> ()  [unwired: 1 in, 4 out]
            n97 = invoke on="Help" class="Str" method="Reinit To Default"() -> ()  [unwired: 3 in, 3 out]
          }
          event "System Hardware Connection Status.Digitizer": Mouse Enter {
            n98 = event-data() -> ()  [unwired: 1 in, 4 out]
            n99 = local write "Help"("Status of hardware connections. TCP/IP is optional." ("Help")) -> ()
          }
          event "TCP Connect": Value Change {
            n100 = event-data() -> ("NewVal"=w230:bool)  [unwired: 1 in, 5 out]
            n101 = case shown="True" w230 {
              tunnel: ["TCP: Close\nUI: Update" ("State(s) in Front (\"\")") "TCP: SendSettingMacro\nUI: Update" ("State(s) in Front (\"\")")] -> w231
              frame False {
              }
              frame True {
              }
            }
            n102 = call <vilib>:"Add State(s) to Queue__JKI_lib_State_Machine.vi"("State(s) in Front (\"\")"=w231, "State(s) in (\"\")"=w233) -> ("States Out"=w232:string)  [unwired: 13 in]
          }
          event Panel Close? {
            # "Discard the event because we'll close the front panel ourselves in Macro: Exit"
            # "Close Panel button (pressed) Event\n(this executes Macro: Exit to terminate the VI)"
            n103 = event-data() -> ()  [unwired: 1 in, 1 out]
            n104 = event-data ("Event Filter Node")("Discard?"=TRUE) -> ()  [unwired: 1 in, 1 out]
            n105 = call <vilib>:"Add State(s) to Queue__JKI_lib_State_Machine.vi"("State(s) in Front (\"\")"="Macro: Exit", "State(s) in (\"\")"=w243) -> ("States Out"=w242:string)  [unwired: 13 in]
          }
        }
      }
      frame "---------- Macro ----------" {
        # "Do not put any code in this frame.\n(It is a separator no-op. You can make a copy of this frame to create a new Macro frame)"
        n106 = call <vilib>:"Add State(s) to Queue__JKI_lib_State_Machine.vi"("State(s) in (\"\")"=w248) -> ("States Out"=w247:string)  [unwired: 14 in]
      }
      frame "Macro: Initialize" {
        # "load Labjack setting 1st as it contaisn laser pin infortmation"
        # "start laser 1st, need 7.5s for laser to get ready"
        # "Initialization Macro\n(This is called once, when the VI starts)"
        n107 = call <vilib>:"Add State(s) to Queue__JKI_lib_State_Machine.vi"("State(s) in Front (\"\")"="UI: showDisclaimer\nUI: Cursor Set >> Busy\nData: Initialize\nInitialize Core Data\nUI: Initialize\nUI: Front Panel State >> Open\nMacro: LoadSysConfig\nTCP: InitializeNew\nTCP: checkSource\nUI: Update\nLabJack: Open\nLabJack: SetDefaultSub\nLED: OpenVIRef\nLED: BreathOrange\nUI: Update\n355 Laser: CheckControllerStatus\n355 Laser: Laser enable\n355 Laser: Dewelling>>500\n355 Laser: CheckControllerStatus\nUI: Update\nLabJack: 355_PWM_Config\nLabJack: AB_PWM_Config\nUI: Update", "State(s) in (\"\")"="UI: Update\nAimingBeam: Initialize\nAimingBeam: Set Status>>Enable\nAimingBeam: Set Current\nUI: Update\n355 Laser: Check Dewelling\nUI: Cursor Set >> Idle\nCase: GetID\nUI: Update\nTCP: SendSettingMacro\nCase: CreatFileStruct\nUI: Update\nLED: BreathOff\nMacro: SysReadyForAq") -> ("States Out"=w249:string)  [unwired: 13 in]
        n108 = call <vilib>:"Add State(s) to Queue__JKI_lib_State_Machine.vi"("State(s) in Front (\"\")"=w249, "State(s) in (\"\")"=w257) -> ("States Out"=w256:string)  [unwired: 13 in]
        "Help" <- "Hover over controls to see help!" ("Help")
      }
      frame "Macro: LoadSysConfig" {
        # "System configuration Macro. [Covers: REQ15]\n(Load configurations for different component of the system)"
        n109 = call <vilib>:"Add State(s) to Queue__JKI_lib_State_Machine.vi"("State(s) in Front (\"\")"="SysConfig: Load AB setting\nSysConfig: Load LJ Pinout\nSysConfig: Load 355 PWM\nSysConfig: LoadABVideoSetting", "State(s) in (\"\")"=w263) -> ("States Out"=w262:string)  [unwired: 13 in]
      }
      frame "Macro: SysReadyForAq" {
        # "Macro for system ready\n(It is a separator no-op. You can make a copy of this frame to create a new Macro frame)"
        n110 = call <vilib>:"Add State(s) to Queue__JKI_lib_State_Machine.vi"("State(s) in Front (\"\")"="UI: ReadyForAquisition\nLED: Green" ("State(s) in Front (\"\")"), "State(s) in (\"\")"=w269) -> ("States Out"=w268:string)  [unwired: 13 in]
      }
      frame "Macro: Exit" {
        # "close LJ last"
        # "check whether hardware is initilized, if so close, if not do nothing"
        # "Exit Macro, close all hardware\n(This is called once, when the VI exits)"
        n111 = Unbundle By Name(w288) -> ("System Status.Digitizer"=w284:bool, "System Status.Aiming Beam"=w283:bool, "System Status.355 Laser"=w282:bool, "System Status.Labjack"=w273:bool, "Core.Close Panel on Exit?"=w277:bool)
        n112 = case shown="True" w284 {
          tunnel: ["" ("Empty String Constant") ""] -> w279
          frame False {
          }
          frame True {
          }
        }
        n113 = case shown="True" w273 {
          tunnel: ["" ("Empty String Constant") "LabJack: SetDefaultAndClose"] -> w270
          frame False {
          }
          frame True {
          }
        }
        n114 = case shown="True" w283 {
          tunnel: ["" ("Empty String Constant") "AimingBeam: Set Status >> Disable\nAimingBeam: Close"] -> w272
          frame False {
          }
          frame True {
          }
        }
        n115 = case shown="True" w282 {
          tunnel: ["" ("Empty String Constant") "355 Laser: Close\n355 Laser: CheckControllerStatus"] -> w271
          frame False {
          }
          frame True {
          }
        }
        n116 = Select(t="UI: Front Panel State >> Close", s=w277, f="" ("Empty String Constant")) -> (s? t:f=w274:string)
        n117 = call <vilib>:"Add State(s) to Queue__JKI_lib_State_Machine.vi"("State(s) in Front (\"\")"="TCP: Close", "State(s) in (\"\")"=w279, "State(s) at Back (\"\")"=w272) -> ("States Out"=w281:string)  [unwired: 12 in]
        n118 = call <vilib>:"Add State(s) to Queue__JKI_lib_State_Machine.vi"("State(s) in Front (\"\")"=w281, "State(s) in (\"\")"=w271, "State(s) at Back (\"\")"=w270) -> ("States Out"=w276:string)  [unwired: 12 in]
        n119 = call <vilib>:"Add State(s) to Queue__JKI_lib_State_Machine.vi"("State(s) in Front (\"\")"=w276, "State(s) in (\"\")"="UI: Update\nLED: CloseVIRef\nData: Cleanup\nExit", "State(s) at Back (\"\")"=w274) -> ("States Out"=w285:string)  [unwired: 12 in]
        n120 = call <vilib>:"Add State(s) to Queue__JKI_lib_State_Machine.vi"("State(s) in Front (\"\")"=w285, "State(s) in (\"\")"=w291) -> ("States Out"=w290:string)  [unwired: 13 in]
      }
      frame "---------- Data ----------" {
        # "Do not put any code in this frame.\n(It is a separator no-op. You can make a copy of this frame to create a new Data frame)"
        n121 = call <vilib>:"Add State(s) to Queue__JKI_lib_State_Machine.vi"("State(s) in (\"\")"=w304) -> ("States Out"=w303:string)  [unwired: 14 in]
      }
      frame "Data: Initialize" {
        w305 = FALSE  # bothVidSourceAvail
        w306 = T1 {"Main Frame Grabber"=FALSE, "Side Frame Grabber"=FALSE, "Main Camera"=FALSE, "Side Camera"=FALSE}  # video source
        w307 = FALSE  # LED vi ref open?
        w309 = path ""  # CaliPath
        w310 = T14 {"DeCon Channel"=enum."1", "Scale Bar"=FALSE, "Scale Low"=3.0, "Scale High"=8.0, "ANSI"=20.0, "Radius"=1.0, "3D?"=FALSE, "Firefly?"=FALSE, "Pentero?"=FALSE}  # VideoConfig
        w311 = T16 {"Ch1APDSerial#"="", "Ch2APDSerial#"="", "Ch3APDSerial#"=""}  # APDSerialNum
        w312 = u32 0  # Aquisition Timer
        w313 = cluster{"RunID":i8, "BG ID":i8, "Cali ID":i8} {"RunID"=1, "BG ID"=1, "Cali ID"=1}  # IDs
        w314 = refnum<vi> refnum  # LED vi reference
        w315 = path ""  # TempPath
        w316 = T17 {"DataPath"=path "", "BG Path"=path "", "iRFPath"=path "", "CaliPath"=path ""}  # Pathes
        w318 = dbl[] []  # V3
        w319 = dbl[] []  # V2
        w320 = dbl[] []  # V1
        w322 = u32 0  # FastTimer
        w323 = u32 0  # SlowTimer
        w324 = dbl[][] []  # Ch3Data
        w325 = dbl[][] []  # Ch2Data
        w308 = dbl[][] []  # Ch1Data
        w328 = T2 {"Digitizer"=FALSE, "Labjack"=FALSE, "Aiming Beam"=FALSE, "355 Laser"=FALSE, "TCP/IP"=FALSE}  # System Status
        w329 = T18 {"DIO_EF_CLOCK1_DIVISOR"=16, "DIO_EF_CLOCK1_ROLL_VALUE"=25000, "DIO#_EF_INDEX"=0, "DIO#_EF_OPTIONS"=1, "DIO#_EF_CONFIG_A"=6250}  # AB PWM setting
        w330 = T4 {"Ch1 Bias"="TDA11", "Ch2 Bias"="DAC10", "Ch3 Bias"="DAC0", "Ch4 Bias"="DAC0", "355 PWM"="FIO0", "AimingBeam PWM"="FIO2", "Laser Ready"="FIO3", "Interlock"="FIO1", "Laser Start/Stop"="FIO1", "Red LED"="FIO1", "Green LED"="FIO1", "Foot Pedal"="DIO15"}  # LJ Pinout
        w331 = 0  # TCP attempt count
        w332 = u32 0  # Laser start tic
        w333 = refnum<k20>[] []  # niTClk sessions
        w334 = u32 0  # Last Trigger
        w335 = T18 {"DIO_EF_CLOCK1_DIVISOR"=16, "DIO_EF_CLOCK1_ROLL_VALUE"=25000, "DIO#_EF_INDEX"=0, "DIO#_EF_OPTIONS"=1, "DIO#_EF_CONFIG_A"=6250}  # 355 PWM setting
        w336 = T19 {"Aiming Beam COM Port"="COM3", "Min Current"=0.0, "Max Current"=63.0, "Default Current"=20.0, "Freq"=0}  # AB Cluster
        w337 = T20 {"resource name"="", "resource name 2"="", "Channel"=enum."Channel 0", "trigger source"="VAL_EXTERNAL", "trigger level"=0.5, "trigger delay"=1.35e-07, "min sample rate"=12500000000.0, "min record length"=2500, "vertical range"=1.0, "vertical offset"=-0.25, "Waveform to Avg"=2000}  # FLImDAQ
        w338 = FALSE  # SysRunning?
        w326 = path ""  # DefaultPath
        w339 = ""  # CaseID
        w340 = T21 {"Ch1Enable?"=FALSE, "Ch2Enable?"=FALSE, "Ch3Enable?"=FALSE, "Ch1AutoGain?"=FALSE, "Ch2AutoGain?"=FALSE, "Ch3AutoGain?"=FALSE, "AimingBeamEnable?"=FALSE}  # SysConfigCluster
        w341 = T22 {"Current VI Reference"=refnum, "Close Panel on Exit?"=FALSE}  # Core
        # "Initialize the shift-register data, here.\n(data names are defined by what you wire into the bundle function)"
        n122 = Bundle("Core"=w341, "SysConfigCluster"=w340, "System Status"=w328, "IDs"=w313, "CaseID"=w339, "DefaultPath"=w326, "Pathes"=w316, "FLImDAQ"=w337, "SysRunning?"=w338, "AB Cluster"=w336, "LJ Pinout"=w330, "355 PWM setting"=w335, "AB PWM setting"=w329, "Last Trigger"=w334, "niTClk sessions"=w333, "Laser start tic"=w332, "TCP attempt count"=w331, "Ch1Data"=w308, "Ch2Data"=w325, "Ch3Data"=w324, "V1"=w320, "V2"=w319, "V3"=w318, "SlowTimer"=w323, "FastTimer"=w322, "listener ID"=refnum<k5> refnum, "TempPath"=w315, "LED vi reference"=w314, "Aquisition Timer"=w312, "APDSerialNum"=w311, "VideoConfig"=w310, "CaliPath"=w309, "LED vi ref open?"=w307, "video source"=w306, "bothVidSourceAvail"=w305) -> (w317:T15)  [unwired: 1 in]
        n123 = call <vilib>:"Add State(s) to Queue__JKI_lib_State_Machine.vi"("State(s) in (\"\")"=w344) -> ("States Out"=w343:string)  [unwired: 14 in]
      }
      frame "Data: Cleanup" {
        # "Cleanup any data and references, here.\n(this is called automatically, by the Macro: Exit)"
        n124 = Unbundle By Name(w346) -> ("Core.Current VI Reference"=w349:refnum<vi>)
        n125 = Close Reference(reference=w349, error in (no error)=w348) -> (error out=w347:errorcluster)
        n126 = call <vilib>:"Add State(s) to Queue__JKI_lib_State_Machine.vi"("State(s) in (\"\")"=w351) -> ("States Out"=w350:string)  [unwired: 14 in]
      }
      frame "---------- Core ----------" {
        # "Do not put any code in this frame.\n(it is a separator no-op)"
        n127 = call <vilib>:"Add State(s) to Queue__JKI_lib_State_Machine.vi"("State(s) in (\"\")"=w356) -> ("States Out"=w355:string)  [unwired: 14 in]
      }
      frame Default {
        w367 = 42 items=["No error", "Argument error", "Memory is full", "Out of zone", "End of file", "File already open", "Generic file I/O error", "File not found", "File permission error", "Disk is full", "Duplicate path", "Too many files open", "System feature not enabled", "Resource file not found", "Cannot add resource", "Resource not found", "Image not found", "Image memory error", "Pen does not exist", "Config type invalid", "Config token not found", "Config parse error", "Config memory error", "Bad external code format", "Bad external code offset", "External code not present", "Null window", "Destroy window error", "Null menu", "Print aborted", "Bad print record", "Print driver error", "Windows error during printing", "Memory error during printing", "Print dialog error", "Generic print error", "Invalid device refnum", "Device not found", "Device parameter error", "Device unit error", "Cannot open device", "Device call aborted", "Generic error", "Cancelled by user", "Object ID too low", "Object ID too high", "Object not in heap", "Unknown heap", "Unknown object (invalid DefProc)", "Unknown object (DefProc not in table)", "Message out of range", "Invalid (null) method", "Unknown message", "Manager call not supported", "Bad address", "Network operation in progress", "Network operation timed out", "Connection is busy", "Network attribute not supported", "Network error", "Address in use", "System out of memory", "Connection aborted", "Connection refused", "Not connected", "Already connected", "Connection closed", "Initialization error (interapplication manager)", "Bad occurrence", "Wait on unbound occurrence handler", "Occurrence queue overflow", "Datalog type conflict", "Unused", "Unrecognized type (interapplication manager)", "Memory corrupt", "Failed to make temporary DLL", "Old CIN version", "Drag socket not found", "Failed to load drop-object", "Failed to register OLE object", "Failed to release OLE object", "Format specifier type mismatch", "Unknown format specifier", "Too few format specifiers", "Too many format specifiers", "Scan failed", "Newer CIN version", "Error converting to variant", "Runtime menu error", "Password tampered", "Variant attribute not found", "Incompatible variant data type", "Event data is not available", "Event Store is not present", "Occurrence is not found", "Event Queue is not created", "Event info is not available", "Refnum passed is NULL", "Error retrieving Class GUID", "Error retrieving CoClass GUID", "Error retrieving TypeLib GUID.", "Bad built application magic bytes.", "Specific driver is different from the specific driver associated with the Logical Name.", "There is no session opened to the class driver.", "Max Error", "MAX - Error with config objects", "MAX - Error loading configuration", "MAX - Group not supported"]
        # "Current State"
        # "Do not delete, rename, or modify this frame.\n(this is used to capture unhandled states and typos)"
        # "Handle mistyped state name (developer tool)"
        n128 = Format Into String(format string="Software Exception: Unhandled State \"%s\"." ("message"), error in=w363, w358) -> (resulting string=w366:string, error out=w365:errorcluster)  [unwired: 1 in]
        n129 = call <vilib>:"Error Cluster From Error Code.vi"("show call chain? (False)"=TRUE, "error in (no error)"=w365, "error message (\"\")"=w366, "error code (0)"=w367) -> ("error out"=w364:errorcluster)  [unwired: 5 in]
        n130 = call <vilib>:"Add State(s) to Queue__JKI_lib_State_Machine.vi"("State(s) in (\"\")"=w362) -> ("States Out"=w361:string)  [unwired: 14 in]
      }
      frame "Initialize Core Data" {
        # "Build default path based on the location of project"
        # "Do not delete, rename, or modify this frame.\n(this is used to determine panel behavior on exit)"
        # "originally closed?"
        # "exe?"
        # "If panel starts closed or is an EXE, then close it when we exit"
        n131 = call <vilib>:"Application Directory.vi"() -> ("Application Directory"=w371:path)
        n132 = property on="Property Node" class="App"() -> ("App.Kind"=w385:T11)  [unwired: 2 in, 2 out]
        n133 = property on="Property Node" class="VI"() -> ("FP.State"=w379:T10)  [unwired: 2 in, 2 out]
        n134 = control-ref of="Current VI Reference"() -> (w380:refnum<vi>)
        n135 = Equal?(x=w379, y=T10."Closed" ("Front Panel Window:State")) -> (x = y?=w377:bool)
        n136 = Equal?(x=w385, y=T11."Run Time System" ("Application:Kind")) -> (x = y?=w383:bool)
        n137 = Build Path(base path=w371, name or relative path="Data") -> (appended path=w375:path)
        n138 = Build Path(base path=w371, name or relative path="SystemTemp") -> (appended path=w372:path)
        n139 = Build Path(base path=w371, name or relative path="SystemCalibrationFile") -> (appended path=w369:path)
        n140 = Or(x=w377, y=w383) -> (x .or. y?=w381:bool)
        n141 = Bundle By Name(cluster=w382, "Core.Current VI Reference"=w380, "Core.Close Panel on Exit?"=w381, "DefaultPath"=w375, "TempPath"=w372, "CaliPath"=w369) -> (w387:T15)
        n142 = call <vilib>:"Add State(s) to Queue__JKI_lib_State_Machine.vi"("State(s) in (\"\")"=w389) -> ("States Out"=w388:string)  [unwired: 14 in]
      }
      frame "Error Handler" {
        # "Unhandled Error -- Display it"
        # "Handle any errors here.\nYou can also output any states to clean-up after errors occur"
        # "Clear error"
        n143 = Unbundle By Name(w390) -> ("code"=w392:i32)
        n144 = case shown="5001" w392 {
          tunnel: ["Macro: Exit" w402 w408] -> w391
          tunnel: w390 -> [w398 _ _]
          frame Default {
            w400 = T23 1 items=["no dialog", "OK message", "continue or stop message", "OK message + warnings", "continue/stop + warnings"] ("type of dialog (OK msg:1)")
            n145 = call <vilib>:"General Error Handler.vi"("type of dialog (OK msg:1)"=w400, "error in (no error)"=w398) -> ()  [unwired: 9 in, 5 out]
          }
          frame 5002 {
            n146 = Two Button Dialog(message="Laser interlock open! Please close interlock and try again! ", 1:"Safely Shutdown" ("F button name (\"Cancel\")"), 2:"OK" ("T button name (\"OK\")")) -> (T button?=w403:bool)
            n147 = case shown="True" w403 {
              tunnel: ["Macro: Exit" "355 Laser: CheckControllerStatus"] -> w402
              frame False {
              }
              frame True {
              }
            }
          }
          frame 5001 {
            n148 = Two Button Dialog(message="Unable to connect to imaging computer, do you want to run data aquisiton alone? ", 1:"No" ("F button name (\"Cancel\")"), 2:"Yes" ("T button name (\"OK\")")) -> (T button?=w409:bool)
            n149 = case shown="False" w409 {
              tunnel: ["Macro: Exit" "" ("Empty String Constant")] -> w408
              frame False {
              }
              frame True {
              }
            }
          }
        }
        n150 = call <vilib>:"Add State(s) to Queue__JKI_lib_State_Machine.vi"("State(s) in Front (\"\")"=w391, "State(s) in (\"\")"=w397) -> ("States Out"=w396:string)  [unwired: 13 in]
      }
      frame "Exit" {
        # "Do not put any code in this frame.\n(No errors that occur here will be handled.)"
        n151 = call <vilib>:"Add State(s) to Queue__JKI_lib_State_Machine.vi"("State(s) in (\"\")"=w420) -> ("States Out"=w419:string)  [unwired: 14 in]
      }
      frame "---------- Case ----------" {
        # "Template Separator\n(You can make a copy of, or modify, this frame)"
        n152 = call <vilib>:"Add State(s) to Queue__JKI_lib_State_Machine.vi"("State(s) in (\"\")"=w425) -> ("States Out"=w424:string)  [unwired: 14 in]
      }
      frame "Case: GetID" {
        # "Template Separator\n(You can make a copy of, or modify, this frame)"
        n153 = call "set_subjectID.vi"() -> ("subject_id"=w426:string)  [unwired: 10 in]
        n154 = Bundle By Name(cluster=w428, "CaseID"=w426) -> (w429:T15)
        n155 = call <vilib>:"Add State(s) to Queue__JKI_lib_State_Machine.vi"("State(s) in (\"\")"=w432) -> ("States Out"=w431:string)  [unwired: 14 in]
      }
      frame "Case: getCaliID" {
        # "Get Calibration file #\n(You can make a copy of, or modify, this frame)"
        n156 = Unbundle By Name(w433) -> ("Pathes.CaliPath"=w436:path)
        n157 = call <vilib>:"Recursive File List.vi"("pattern"="*.tdms", "Treat LLBs as Folders?"=FALSE, "Folder Path"=w436) -> ("All Files in Dir"=w441:path[])  [unwired: 4 in, 4 out]
        n158 = for {
          tunnel: w441 -> [w451] mode=indexing
          tunnel: [w450] -> w440 mode=indexing
          tunnel: "Calibration" -> [w447]
          n159 = Strip Path(path=w451) -> (name=w448:string)  [unwired: 1 out]
          n160 = Search and Replace String(input string=w448, search string=w447) -> (result string=w446:string)  [unwired: 6 in, 3 out]
          n161 = Scan From String(format string="%d" ("string"), input string=w446) -> (output 1=w450:i32)  [unwired: 3 in, 3 out]
        }
        n162 = Array Max & Min(array=w440) -> (max value=w439:i32)  [unwired: 3 out]
        n163 = Bundle By Name(cluster=w433, "IDs.Cali ID"=w439) -> (w434:T15)
        n164 = call <vilib>:"Add State(s) to Queue__JKI_lib_State_Machine.vi"("State(s) in (\"\")"=w445) -> ("States Out"=w444:string)  [unwired: 14 in]
      }
      frame "Case: getBGID" {
        # "Get background #\n(You can make a copy of, or modify, this frame)"
        n165 = Unbundle By Name(w454) -> ("Pathes.BG Path"=w459:path)
        n166 = call <vilib>:"Recursive File List.vi"("pattern"="*.tdms", "Treat LLBs as Folders?"=FALSE, "Folder Path"=w459) -> ("All Files in Dir"=w457:path[])  [unwired: 4 in, 4 out]
        n167 = for {
          tunnel: w457 -> [w474] mode=indexing
          tunnel: "Background" ("name or relative path") -> [w472]
          shift-right: [w465] -> w452
          shift-left: 0 -> [w469]
          n168 = Strip Path(path=w474) -> (name=w473:string)  [unwired: 1 out]
          n169 = Search and Replace String(input string=w473, search string=w472) -> (number of replacements=w471:i32)  [unwired: 6 in, 3 out]
          n170 = Greater Than 0?(x=w471) -> (x > 0?=w470:bool)
          n171 = Select(t=1, s=w470, f=0) -> (s? t:f=w468:i32)
          n172 = Add(x=w468, y=w469) -> (x+y=w465:i32)
        }
        n173 = Bundle By Name(cluster=w454, "IDs.BG ID"=w452) -> (w455:T15)
        n174 = call <vilib>:"Add State(s) to Queue__JKI_lib_State_Machine.vi"("State(s) in (\"\")"=w464) -> ("States Out"=w463:string)  [unwired: 14 in]
      }
      frame "Case: getRunID" {
        # "Check folder for run ID\n(You can make a copy of, or modify, this frame)"
        n175 = Unbundle By Name(w484) -> ("Pathes.DataPath"=w483:path, "CaseID"=w479:string)
        n176 = Build Array("Background" ("name or relative path"), "Calibration", "3DScanData" ("element")) -> (w489:string[])
        n177 = call <vilib>:"Recursive File List.vi"("Folders to Exclude"=w489, "pattern"="*.tdms", "Treat LLBs as Folders?"=FALSE, "Folder Path"=w483) -> ("All Files in Dir"=w480:path[])  [unwired: 3 in, 4 out]
        n178 = for {
          tunnel: w480 -> [w498] mode=indexing
          tunnel: [w497] -> w486 mode=indexing
          tunnel: w479 -> [w494]
          n179 = Strip Path(path=w498) -> (name=w495:string)  [unwired: 1 out]
          n180 = Search and Replace String(input string=w495, search string=w494) -> (result string=w493:string)  [unwired: 6 in, 3 out]
          n181 = Scan From String(format string="_%d" ("string"), input string=w493) -> (output 1=w497:i32)  [unwired: 3 in, 3 out]
        }
        n182 = Array Max & Min(array=w486) -> (max value=w477:i32)  [unwired: 3 out]
        n183 = Bundle By Name(cluster=w484, "IDs.RunID"=w477) -> (w485:T15)
        n184 = call "RunIDFGV.vi"("Error In"=w475, "RunID in"=w477) -> ("Error Out"=w476:errorcluster)  [unwired: 8 in, 1 out]
        n185 = call <vilib>:"Add State(s) to Queue__JKI_lib_State_Machine.vi"("State(s) in (\"\")"=w492) -> ("States Out"=w491:string)  [unwired: 14 in]
      }
      frame "Case: CreatFileStruct" {
        # "Creat case file structure"
        n186 = Unbundle By Name(w512) -> ("DefaultPath"=w518:path, "CaseID"=w505:string)
        n187 = Build Path(base path=w518, name or relative path=w505) -> (appended path=w517:path)
        n188 = call <vilib>:"Check if File or Folder Exists.vi"("error in (no error)"=w511, "path"=w517) -> ("error out"=w514:errorcluster, "file or folder exists?"=w516:bool, "dup path"=w515:path)  [unwired: 7 in]
        n189 = case shown="True" w516 {
          tunnel: w515 -> [w535 w543]
          tunnel: w514 -> [w533 w538]
          tunnel: [w527 w543] -> w503
          tunnel: [w531 w545] -> w502
          tunnel: [u32 0 u32 0] -> w501
          tunnel: [w529 w548] -> w509
          tunnel: "Background" ("name or relative path") -> [w528 w540]
          tunnel: "Calibration" -> [w526 w539]
          tunnel: [w522 w541] -> w506
          tunnel: w505 -> [_ _]
          tunnel: ["" ("Empty String Constant") "Case: getRunID\nCase: getBGID\nCase: getCaliID\nUI: Update"] -> w504
          frame False {
            # "Folder not exist. Creat folders."
            n190 = Create Folder(path (use dialog)=w535, error in=w533) -> (created path=w527:path, error out=w524:errorcluster)  [unwired: 1 in, 1 out]
            n191 = Build Path(base path=w527, name or relative path=w526) -> (appended path=w525:path)
            n192 = Build Path(base path=w527, name or relative path=w528) -> (appended path=w534:path)
            n193 = Create Folder(path (use dialog)=w534, error in=w524) -> (created path=w529:path, error out=w530:errorcluster)  [unwired: 1 in, 1 out]
            n194 = Create Folder(path (use dialog)=w525, error in=w524) -> (created path=w522:path, error out=w523:errorcluster)  [unwired: 1 in, 1 out]
            n195 = Merge Errors(w530, w523) -> (w531:errorcluster)
          }
          frame True {
            # "Folder exsit, check file #"
            n196 = Build Path(base path=w543, name or relative path=w539) -> (appended path=w544:path)
            n197 = Build Path(base path=w543, name or relative path=w540) -> (appended path=w549:path)
            n198 = call <vilib>:"Check if File or Folder Exists.vi"("path"=w544) -> ("file or folder exists?"=w542:bool, "dup path"=w541:path)  [unwired: 8 in, 1 out]
            n199 = call <vilib>:"Check if File or Folder Exists.vi"("path"=w549) -> ("file or folder exists?"=w547:bool, "dup path"=w548:path)  [unwired: 8 in, 1 out]
            n200 = And(x=w547, y=w542) -> (x .and. y?=w546:bool)
            n201 = case shown="False" w546 {
              tunnel: w538 -> [_ w551]
              tunnel: [errorcluster {"status"=TRUE, "code"=5003, "source"="File structure error."} ("error out") w551] -> w545
              frame False {
              }
              frame True {
              }
            }
          }
        }
        n202 = Bundle By Name(cluster=w512, "Pathes.DataPath"=w503, "Pathes.BG Path"=w509, "Pathes.CaliPath"=w506, "IDs.RunID"=w501, "IDs.BG ID"=w501, "IDs.Cali ID"=w501) -> (w513:T15)
        n203 = call "DataRootPathFGV.vi"("Error In"=w502, "PathIn"=w503) -> ("Error Out"=w500:errorcluster)  [unwired: 8 in, 1 out]
        n204 = call "RunIDFGV.vi"("Error In"=w500, "RunID in"=w501) -> ("Error Out"=w499:errorcluster)  [unwired: 8 in, 1 out]
        n205 = call <vilib>:"Add State(s) to Queue__JKI_lib_State_Machine.vi"("State(s) in Front (\"\")"=w504, "State(s) in (\"\")"=w520) -> ("States Out"=w519:string)  [unwired: 13 in]
      }
      frame "---------- LabJack ----------" {
        # "Template Separator\n(You can make a copy of, or modify, this frame)"
        n206 = call <vilib>:"Add State(s) to Queue__JKI_lib_State_Machine.vi"("State(s) in (\"\")"=w556) -> ("States Out"=w555:string)  [unwired: 14 in]
      }
      frame "LabJack: checkPedal" {
        # "Template Separator\n(You can make a copy of, or modify, this frame)"
        n207 = Unbundle By Name(w557) -> ("LJ Pinout.Foot Pedal"=w561:string)
        n208 = call "LabJack_FGV.vi"("Operation(Read)"=enum16{"Write", "Read"}."Read" ("Operation"), "error in (no error)"=w559) -> ("error out"=w563:errorcluster, "Read data"=w564:i32)  [unwired: 8 in]
        n209 = call "LJM_eReadName.vi"("Handle In"=w564, "Name"=w561, "error in"=w563) -> ("Value"=w562:dbl, "error out"=w560:errorcluster)  [unwired: 10 in, 1 out]
        n210 = case shown="1" w562 {
          tunnel: w557 -> [w569 w572]
          tunnel: [w569 w570] -> w558
          frame 0, Default {
          }
          frame 1 {
            # "If Pedal pressed"
            n211 = Tick Count (ms)() -> (millisecond timer value=w576:u32)
            n212 = Unbundle By Name(w572) -> ("Last Trigger"=w571:u32)
            n213 = Subtract(x=w576, y=w571) -> (x-y=w575:u32)
            n214 = Greater Or Equal?(x=w575, y=u32 2000) -> (x >= y?=w573:bool)
            n215 = case shown="True" w573 {
              tunnel: w572 -> [w577 w578]
              tunnel: w571 -> [_ _]
              tunnel: [w577 w579] -> w570
              frame False {
              }
              frame True {
                n216 = Tick Count (ms)() -> (millisecond timer value=w580:u32)
                n217 = Unbundle By Name(w578) -> ("SysRunning?"=w581:bool)
                n218 = case shown="False" w581 {
                  frame False {
                    n219 = property on="StartButton" class="Bool (strict)"("Val(Sgnl)"=TRUE ("Value (Signaling)")) -> ()  [unwired: 2 in, 2 out]
                  }
                  frame True {
                    n220 = property on="StopButton" class="Bool (strict)"("Val(Sgnl)"=TRUE ("Value (Signaling)")) -> ()  [unwired: 2 in, 2 out]
                  }
                }
                n221 = Bundle By Name(cluster=w578, "Last Trigger"=w580) -> (w579:T15)
              }
            }
          }
        }
        n222 = call <vilib>:"Add State(s) to Queue__JKI_lib_State_Machine.vi"("State(s) in (\"\")"=w568) -> ("States Out"=w567:string)  [unwired: 14 in]
      }
      frame "LabJack: ZeroV" {
        # "Just Zero V\nDO not update FGV and front panel\nWIll resume from last V"
        # "set bias to 0"
        # "Zero APD bias\n(You can make a copy of, or modify, this frame)"
        n223 = Unbundle By Name(w586) -> ("LJ Pinout.Ch1 Bias"=w591:string, "LJ Pinout.Ch2 Bias"=w590:string, "LJ Pinout.Ch3 Bias"=w589:string)
        n224 = Build Array(w591, w590, w589) -> (w588:string[])
        n225 = call "LabJack_FGV.vi"("Operation(Read)"=enum16{"Write", "Read"}."Read" ("Operation"), "error in (no error)"=w585) -> ("error out"=w592:errorcluster, "Read data"=w593:i32)  [unwired: 8 in]
        n226 = call "LJM_eWriteNames.vi"("Handle In"=w593, "aNames"=w588, "aValuesIn"=dbl[] [0.0, 0.0, 0.0], "error in"=w592) -> ("error out"=w584:errorcluster)  [unwired: 9 in, 2 out]
        n227 = call <vilib>:"Add State(s) to Queue__JKI_lib_State_Machine.vi"("State(s) in (\"\")"=w597) -> ("States Out"=w596:string)  [unwired: 14 in]
      }
      frame "LabJack: SetV" {
        # "set bias to user specifid"
        # "Zero APD bias\n(You can make a copy of, or modify, this frame)"
        n228 = Unbundle By Name(w611) -> ("LJ Pinout.Ch1 Bias"=w615:string, "LJ Pinout.Ch2 Bias"=w614:string, "LJ Pinout.Ch3 Bias"=w613:string)
        n229 = call "V1FGV.vi"("Error In"=w610, "action (write)"=enum16{"write", "read"}."read") -> ("Error Out"=w609:errorcluster, "V1 out"=w603:dbl)  [unwired: 8 in]
        n230 = call "V2FGV.vi"("Error In"=w609, "action(write)"=enum16{"write", "read"}."read") -> ("Error Out"=w608:errorcluster, "V2 out"=w602:dbl)  [unwired: 8 in]
        n231 = Build Array(w615, w614, w613) -> (w612:string[])
        n232 = call "V3FGV.vi"("Error In"=w608, "action(write)"=enum16{"write", "read"}."read" ("action(read)")) -> ("Error Out"=w605:errorcluster, "V3 out"=w601:dbl)  [unwired: 8 in]
        n233 = Build Array(w603, w602, w601) -> (w604:dbl[])
        n234 = call "LabJack_FGV.vi"("Operation(Read)"=enum16{"Write", "Read"}."Read" ("Operation"), "error in (no error)"=w610) -> ("error out"=w616:errorcluster, "Read data"=w617:i32)  [unwired: 8 in]
        n235 = call "LJM_eWriteNames.vi"("Handle In"=w617, "aNames"=w612, "aValuesIn"=w604, "error in"=w616) -> ("error out"=w606:errorcluster)  [unwired: 9 in, 2 out]
        n236 = Merge Errors(w605, w606) -> (w607:errorcluster)
        n237 = call <vilib>:"Add State(s) to Queue__JKI_lib_State_Machine.vi"("State(s) in (\"\")"=w621) -> ("States Out"=w620:string)  [unwired: 14 in]
      }
      frame "LabJack: Open" {
        # "Initialize LabJack T7\nEstablish connection and initialize pins"
        n238 = call "LJ_Open.vi"("error in"=w631, "DeviceType"="LJM_dtT7") -> ("error out"=w628:errorcluster, "Success?"=w629:bool, "Handle Out"=w623:i32)  [unwired: 7 in]
        n239 = call "LabJack_FGV.vi"("Operation(Read)"=enum16{"Write", "Read"}."Write" ("Operation"), "error in (no error)"=w628, "Write data"=w623) -> ("error out"=w625:errorcluster)  [unwired: 7 in, 1 out]
        n240 = Bundle By Name(cluster=w626, "System Status.Labjack"=w629) -> (w630:T15)
        n241 = call <vilib>:"Add State(s) to Queue__JKI_lib_State_Machine.vi"("State(s) in (\"\")"=w633) -> ("States Out"=w632:string)  [unwired: 14 in]
      }
      frame "LabJack: SetDefaultSub" {
        w650 = "_EF_ENABLE" ("string")
        # "1. Disable PWM\n2. Set all V to 0\n3. Set 355 relay to open\n4. Set LED to off"
        # "read once to set DIO to input"
        # "set all initila V to 0. Set footpedal to input. Set PWM to low. Set laser relay to open. Set LEDs to yellow."
        # "Set Labjack to correct input and output state and initial values"
        n242 = Unbundle By Name(w647) -> ("LJ Pinout.355 PWM"=w652:string, "LJ Pinout.AimingBeam PWM"=w651:string, "LJ Pinout.Ch1 Bias"=w659:string, "LJ Pinout.Ch2 Bias"=w665:string, "LJ Pinout.Ch3 Bias"=w664:string, "LJ Pinout.Laser Start/Stop"=w663:string, "LJ Pinout.Red LED"=w662:string, "LJ Pinout.Green LED"=w661:string)
        n243 = call "V1FGV.vi"("Error In"=w640, "action (write)"=enum16{"write", "read"}."write" ("action"), "V1 in"=0.0) -> ("Error Out"=w641:errorcluster)  [unwired: 7 in, 1 out]
        n244 = call "LabJack_FGV.vi"("Operation(Read)"=enum16{"Write", "Read"}."Read" ("Operation"), "error in (no error)"=w640) -> ("error out"=w655:errorcluster, "Read data"=w656:i32)  [unwired: 8 in]
        n245 = call "V2FGV.vi"("Error In"=w641, "action(write)"=enum16{"write", "read"}."write" ("action"), "V2 in"=0.0) -> ("Error Out"=w637:errorcluster)  [unwired: 7 in, 1 out]
        n246 = Concatenate Strings(w652, w650) -> (w649:string)
        n247 = Concatenate Strings(w651, w650) -> (w648:string)
        n248 = call "V3FGV.vi"("Error In"=w637, "action(write)"=enum16{"write", "read"}."write" ("action"), "V3 in"=0.0) -> ("Error Out"=w634:errorcluster)  [unwired: 7 in, 1 out]
        n249 = Build Array(w649, w648, w659, w665, w664, w663, w662, w661) -> (w660:string[])
        n250 = Unbundle By Name(w647) -> ("LJ Pinout.Foot Pedal"=w646:string)
        n251 = call "LJM_eWriteNames.vi"("Handle In"=w656, "aNames"=w660, "aValuesIn"=dbl[] [0.0, 0.0, 0.0, 0.0, 0.0, 0.0, 0.0, 0.0], "error in"=w655) -> ("Handle Out"=w654:i32, "error out"=w653:errorcluster)  [unwired: 9 in, 1 out]
        n252 = call "LJM_eReadName.vi"("Handle In"=w654, "Name"=w646, "error in"=w653) -> ("error out"=w636:errorcluster)  [unwired: 10 in, 2 out]
        n253 = Merge Errors(w636, w634) -> (w635:errorcluster)
        n254 = call <vilib>:"Add State(s) to Queue__JKI_lib_State_Machine.vi"("State(s) in (\"\")"=w668) -> ("States Out"=w667:string)  [unwired: 14 in]
      }
      frame "LabJack: FootPedalConfig" {
        # "Setup footPedal\n(You can make a copy of, or modify, this frame)"
        n255 = call "LabJack_FGV.vi"("Operation(Read)"=enum16{"Write", "Read"}."Read" ("Operation"), "error in (no error)"=w670) -> ("error out"=w674:errorcluster, "Read data"=w675:i32)  [unwired: 8 in]
        n256 = call "LJM_eWriteName.vi"("Handle In"=w675, "Name"="DIO15", "Value"=1.0, "error in"=w674) -> ("error out"=w671:errorcluster)  [unwired: 10 in, 1 out]
        n257 = call <vilib>:"Add State(s) to Queue__JKI_lib_State_Machine.vi"("State(s) in (\"\")"=w679) -> ("States Out"=w678:string)  [unwired: 14 in]
      }
      frame "LabJack: SetDefaultAndClose" {
        # "Template Separator\n(You can make a copy of, or modify, this frame)"
        n258 = call <vilib>:"Add State(s) to Queue__JKI_lib_State_Machine.vi"("State(s) in Front (\"\")"="LabJack: SetDefaultSub\nLabJack: Close" ("State(s) in Front (\"\")"), "State(s) in (\"\")"=w685) -> ("States Out"=w684:string)  [unwired: 13 in]
      }
      frame "LabJack: Close" {
        # "Close LabJack Refnum"
        n259 = call "LabJack_FGV.vi"("Operation(Read)"=enum16{"Write", "Read"}."Read" ("Operation"), "error in (no error)"=w691) -> ("error out"=w686:errorcluster, "Read data"=w687:i32)  [unwired: 8 in]
        n260 = Bundle By Name(cluster=w689, "System Status.Labjack"=FALSE ("System Status.Gain Control")) -> (w692:T15)
        n261 = call "LJM_Close.vi"("error in"=w686, "Handle"=w687) -> ("error out"=w694:errorcluster)  [unwired: 9 in]
        n262 = call <vilib>:"Add State(s) to Queue__JKI_lib_State_Machine.vi"("State(s) in (\"\")"=w696) -> ("States Out"=w695:string)  [unwired: 14 in]
      }
      frame "LabJack: Interlock enable/disable" {
        w705 = i8 0  # int8
        # "[Covers: REQ8]"
        # "Interlock enable/disable\n(Usage: \"LabJack: Interlock enable/disable >> 1|0\")"
        n263 = Fract/Exp String To Number(string=w706, default (0 dbl)=w705) -> (number=w702:i8)  [unwired: 2 in, 1 out]
        n264 = Unbundle By Name(w704) -> ("LJ Pinout.Interlock"=w703:string)
        n265 = call "LabJack_FGV.vi"("Operation(Read)"=enum16{"Write", "Read"}."Read" ("Operation")) -> ("Read data"=w700:i32)  [unwired: 9 in, 1 out]
        n266 = call "LJM_eWriteName.vi"("Handle In"=w700, "Name"=w703, "Value"=w702, "error in"=w701) -> ("error out"=w698:errorcluster)  [unwired: 10 in, 1 out]
        n267 = call <vilib>:"Add State(s) to Queue__JKI_lib_State_Machine.vi"("State(s) in (\"\")"=w708) -> ("States Out"=w707:string)  [unwired: 14 in]
      }
      frame "LabJack: 355_PWM_Config" {
        w710 = 0.0 ("element")
        w730 = "DIO_EF_CLOCK1_ENABLE"
        # "Config PWM frequency"
        n268 = Unbundle By Name(w722) -> ("LJ Pinout.355 PWM"=w729:string)
        n269 = Unbundle By Name(w722) -> ("355 PWM setting.DIO_EF_CLOCK1_DIVISOR"=w721:i16, "355 PWM setting.DIO_EF_CLOCK1_ROLL_VALUE"=w720:i32, "355 PWM setting.DIO#_EF_INDEX"=w717:i16, "355 PWM setting.DIO#_EF_OPTIONS"=w716:i16, "355 PWM setting.DIO#_EF_CONFIG_A"=w715:i32)
        n270 = Concatenate Strings(w729, "_EF_ENABLE" ("string")) -> (w725:string)
        n271 = Concatenate Strings(w729, "_EF_INDEX") -> (w728:string)
        n272 = Concatenate Strings(w729, "_EF_OPTIONS") -> (w727:string)
        n273 = Concatenate Strings(w729, "_EF_CONFIG_A") -> (w726:string)
        n274 = call "LabJack_FGV.vi"("Operation(Read)"=enum16{"Write", "Read"}."Read" ("Operation")) -> ("Read data"=w723:i32)  [unwired: 9 in, 1 out]
        n275 = Build Array(w710, w710, w721, w720, 1.0 ("element"), 0.0 ("element"), w717, w716, w715) -> (w714:dbl[])
        n276 = Build Array("DIO_EF_CLOCK0_ENABLE", w730, "DIO_EF_CLOCK1_DIVISOR", "DIO_EF_CLOCK1_ROLL_VALUE", w730, w725, w728, w727, w726) -> (w724:string[])
        n277 = call "LJM_eWriteNames.vi"("Handle In"=w723, "aNames"=w724, "aValuesIn"=w714, "error in"=w712) -> ("error out"=w713:errorcluster)  [unwired: 9 in, 2 out]
        n278 = call <vilib>:"Add State(s) to Queue__JKI_lib_State_Machine.vi"("State(s) in (\"\")"=w739) -> ("States Out"=w738:string)  [unwired: 14 in]
      }
      frame "LabJack: 355_PWM_Start" {
        # "Template Separator\n(You can make a copy of, or modify, this frame)"
        n279 = Unbundle By Name(w747) -> ("LJ Pinout.355 PWM"=w746:string)
        n280 = call "LabJack_FGV.vi"("Operation(Read)"=enum16{"Write", "Read"}."Read" ("Operation"), "error in (no error)"=w741) -> ("error out"=w748:errorcluster, "Read data"=w749:i32)  [unwired: 8 in]
        n281 = Concatenate Strings(w746, "_EF_ENABLE" ("string")) -> (w744:string)
        n282 = call "LJM_eWriteName.vi"("Handle In"=w749, "Name"=w744, "Value"=1.0, "error in"=w748) -> ("error out"=w742:errorcluster)  [unwired: 10 in, 1 out]
        n283 = call <vilib>:"Add State(s) to Queue__JKI_lib_State_Machine.vi"("State(s) in (\"\")"=w752) -> ("States Out"=w751:string)  [unwired: 14 in]
      }
      frame "LabJack: 355_PWM_Stop" {
        # "Template Separator\n(You can make a copy of, or modify, this frame)"
        n284 = Unbundle By Name(w758) -> ("LJ Pinout.355 PWM"=w762:string)
        n285 = call "LabJack_FGV.vi"("Operation(Read)"=enum16{"Write", "Read"}."Read" ("Operation"), "error in (no error)"=w757) -> ("error out"=w763:errorcluster, "Read data"=w755:i32)  [unwired: 8 in]
        n286 = Concatenate Strings(w762, "_EF_ENABLE" ("string")) -> (w760:string)
        n287 = call "LJM_eWriteName.vi"("Handle In"=w755, "Name"=w760, "Value"=0.0, "error in"=w763) -> ("error out"=w754:errorcluster)  [unwired: 10 in, 1 out]
        n288 = local write "355nm Laser toggle"(FALSE ("355nm Laser toggle")) -> ()
        n289 = call <vilib>:"Add State(s) to Queue__JKI_lib_State_Machine.vi"("State(s) in (\"\")"=w766) -> ("States Out"=w765:string)  [unwired: 14 in]
      }
      frame "LabJack: AB_Start" {
        # "Aiming Beam Start\n(Based on aimging beam frequency, set LabJack pin)"
        n290 = Unbundle By Name(w776) -> ("AB Cluster.Freq"=w768:i32, "LJ Pinout.AimingBeam PWM"=w775:string)
        n291 = Greater Than 0?(x=w768) -> (x > 0?=w767:bool)
        n292 = case shown="False" w767 {
          tunnel: w775 -> [w782 w785]
          tunnel: [w782 w783] -> w774
          frame False {
            # "if 0 freq, set PWM pin"
          }
          frame True {
            # "if non zero freq, set PWM enable"
            n293 = Concatenate Strings(w785, "_EF_ENABLE" ("string")) -> (w783:string)
          }
        }
        n294 = call "LabJack_FGV.vi"("Operation(Read)"=enum16{"Write", "Read"}."Read" ("Operation"), "error in (no error)"=w771) -> ("error out"=w777:errorcluster, "Read data"=w778:i32)  [unwired: 8 in]
        n295 = call "LJM_eWriteName.vi"("Handle In"=w778, "Name"=w774, "Value"=1.0, "error in"=w777) -> ("error out"=w772:errorcluster)  [unwired: 10 in, 1 out]
        n296 = local write "Aiming beam toggle"(TRUE ("Aiming beam toggle")) -> ()
        n297 = call <vilib>:"Add State(s) to Queue__JKI_lib_State_Machine.vi"("State(s) in (\"\")"=w781) -> ("States Out"=w780:string)  [unwired: 14 in]
      }
      frame "LabJack: AB_Stop" {
        # "Aiming Beam Stop\n(Based on aiming beam frequency, set LabJack pin low)"
        n298 = Unbundle By Name(w793) -> ("AB Cluster.Freq"=w788:i32, "LJ Pinout.AimingBeam PWM"=w795:string)
        n299 = Greater Than 0?(x=w788) -> (x > 0?=w787:bool)
        n300 = case shown="False" w787 {
          tunnel: w795 -> [w801 w804]
          tunnel: [w801 w802] -> w786
          frame False {
          }
          frame True {
            n301 = Concatenate Strings(w804, "_EF_ENABLE" ("string")) -> (w802:string)
          }
        }
        n302 = call "LabJack_FGV.vi"("Operation(Read)"=enum16{"Write", "Read"}."Read" ("Operation"), "error in (no error)"=w791) -> ("error out"=w796:errorcluster, "Read data"=w797:i32)  [unwired: 8 in]
        n303 = call "LJM_eWriteName.vi"("Handle In"=w797, "Name"=w786, "Value"=0.0, "error in"=w796) -> ("error out"=w792:errorcluster)  [unwired: 10 in, 1 out]
        n304 = local write "Aiming beam toggle"(FALSE ("Aiming beam toggle")) -> ()
        n305 = call <vilib>:"Add State(s) to Queue__JKI_lib_State_Machine.vi"("State(s) in (\"\")"=w800) -> ("States Out"=w799:string)  [unwired: 14 in]
      }
      frame "LabJack: AB_PWM_Config" {
        w806 = 0.0 ("element")
        w826 = "DIO_EF_CLOCK2_ENABLE"
        # "Config PWM frequency"
        n306 = Unbundle By Name(w818) -> ("LJ Pinout.AimingBeam PWM"=w825:string)
        n307 = Unbundle By Name(w818) -> ("AB PWM setting.DIO_EF_CLOCK1_DIVISOR"=w817:i16, "AB PWM setting.DIO_EF_CLOCK1_ROLL_VALUE"=w816:i32, "AB PWM setting.DIO#_EF_INDEX"=w813:i16, "AB PWM setting.DIO#_EF_OPTIONS"=w812:i16, "AB PWM setting.DIO#_EF_CONFIG_A"=w811:i32)
        n308 = Concatenate Strings(w825, "_EF_ENABLE" ("string")) -> (w821:string)
        n309 = Concatenate Strings(w825, "_EF_INDEX") -> (w824:string)
        n310 = Concatenate Strings(w825, "_EF_OPTIONS") -> (w823:string)
        n311 = Concatenate Strings(w825, "_EF_CONFIG_A") -> (w822:string)
        n312 = call "LabJack_FGV.vi"("Operation(Read)"=enum16{"Write", "Read"}."Read" ("Operation")) -> ("Read data"=w819:i32)  [unwired: 9 in, 1 out]
        n313 = Build Array(w806, w806, w817, w816, 1.0 ("element"), 0.0 ("element"), w813, w812, w811) -> (w810:dbl[])
        n314 = Build Array("DIO_EF_CLOCK0_ENABLE", w826, "DIO_EF_CLOCK2_DIVISOR", "DIO_EF_CLOCK2_ROLL_VALUE", w826, w821, w824, w823, w822) -> (w820:string[])
        n315 = call "LJM_eWriteNames.vi"("Handle In"=w819, "aNames"=w820, "aValuesIn"=w810, "error in"=w808) -> ("error out"=w809:errorcluster)  [unwired: 9 in, 2 out]
        n316 = call <vilib>:"Add State(s) to Queue__JKI_lib_State_Machine.vi"("State(s) in (\"\")"=w835) -> ("States Out"=w834:string)  [unwired: 14 in]
      }
      frame "---------- LED ----------" {
        # "Template Separator\n(You can make a copy of, or modify, this frame)"
        n317 = call <vilib>:"Add State(s) to Queue__JKI_lib_State_Machine.vi"("State(s) in (\"\")"=w840) -> ("States Out"=w839:string)  [unwired: 14 in]
      }
      frame "LED: OpenVIRef" {
        # "Template Separator\n(You can make a copy of, or modify, this frame)"
        n318 = call <vilib>:"Application Directory.vi"() -> ("Application Directory"=w847:path)
        n319 = Build Path(base path=w847, name or relative path="SubVI") -> (appended path=w845:path)
        n320 = Build Path(base path=w845, name or relative path="LEDBreath.vi") -> (appended path=w843:path)
        n321 = Open VI Reference(vi path=w843, error in (no error)=w848) -> (vi reference=w849:refnum<vi>, error out=w842:errorcluster)  [unwired: 4 in]
        n322 = case shown="Error .." w842 {
          tunnel: [TRUE FALSE] -> w841
          frame No Error {
          }
          frame Error {
          }
        }
        n323 = Bundle By Name(cluster=w850, "LED vi reference"=w849, "LED vi ref open?"=w841) -> (w851:T15)
        n324 = call <vilib>:"Add State(s) to Queue__JKI_lib_State_Machine.vi"("State(s) in (\"\")"=w854) -> ("States Out"=w853:string)  [unwired: 14 in]
      }
      frame "LED: CloseVIRef" {
        # "Template Separator\n(You can make a copy of, or modify, this frame)"
        n325 = Unbundle By Name(w858) -> ("LED vi reference"=w859:refnum<vi>, "LED vi ref open?"=w857:bool)
        n326 = case shown="True" w857 {
          tunnel: w861 -> [w865 w868]
          tunnel: [w865 w867] -> w860
          tunnel: w859 -> [_ w866]
          frame False {
          }
          frame True {
            n327 = Close Reference(reference=w866, error in (no error)=w868) -> (error out=w867:errorcluster)
          }
        }
        n328 = call <vilib>:"Add State(s) to Queue__JKI_lib_State_Machine.vi"("State(s) in (\"\")"=w864) -> ("States Out"=w863:string)  [unwired: 14 in]
      }
      frame "LED: BreathGreen" {
        w869 = FALSE ("Wait Until Done")
        # "Breath system LED\n(LED: Breath >> True/False)"
        n329 = Unbundle By Name(w877) -> ("LED vi reference"=w876:refnum<vi>)
        n330 = invoke class="VI" method="Ctrl Val.Set"(reference=w876, error in=w874, "Control Name"="Color", "Value"=0) -> (reference out=w873:refnum<vi>, error out=w872:errorcluster)  [unwired: 1 in, 3 out]
        n331 = invoke on="Invoke Node" class="VI" method="Run VI"(reference=w873, error in=w872, "Wait until done"=w869, "Auto Dispose Ref"=w869) -> (error out=w875:errorcluster)  [unwired: 1 in, 4 out]
        n332 = call <vilib>:"Add State(s) to Queue__JKI_lib_State_Machine.vi"("State(s) in (\"\")"=w880) -> ("States Out"=w879:string)  [unwired: 14 in]
      }
      frame "LED: BreathOrange" {
        w881 = FALSE ("Wait Until Done")
        # "Breath system LED\n(LED: Breath >> True/False)"
        n333 = Unbundle By Name(w889) -> ("LED vi reference"=w888:refnum<vi>)
        n334 = invoke class="VI" method="Ctrl Val.Set"(reference=w888, error in=w886, "Control Name"="Color", "Value"=1) -> (reference out=w885:refnum<vi>, error out=w884:errorcluster)  [unwired: 1 in, 3 out]
        n335 = invoke on="Invoke Node" class="VI" method="Run VI"(reference=w885, error in=w884, "Wait until done"=w881, "Auto Dispose Ref"=w881) -> (error out=w887:errorcluster)  [unwired: 1 in, 4 out]
        n336 = call <vilib>:"Add State(s) to Queue__JKI_lib_State_Machine.vi"("State(s) in (\"\")"=w892) -> ("States Out"=w891:string)  [unwired: 14 in]
      }
      frame "LED: BreathOff" {
        # "System LED Breath Off\n(Breath off, check VI status to make sure it is off)"
        n337 = Unbundle By Name(w901) -> ("LED vi reference"=w900:refnum<vi>)
        n338 = invoke on="Invoke Node" class="VI" method="Ctrl Val.Set"(reference=w900, error in=w898, "Control Name"="Stop", "Value"=TRUE) -> (reference out=w893:refnum<vi>, error out=w894:errorcluster)  [unwired: 1 in, 3 out]
        n339 = case shown="No Error" w894 {
          selector: w894 -> [w906 _]
          tunnel: [w905 errorcluster {"status"=FALSE, "code"=0, "source"=""} ("error IO")] -> w899
          tunnel: ["" ("State(s) in Front (\"\")") "LED: BreathOff" ("State(s) in Front (\"\")")] -> w897
          tunnel: w893 -> [w907 _]
          frame No Error {
            # "No error, wait for VI to stop"
            n340 = while {
              tunnel: w907 -> [w915]
              shift-right: [w909] -> w905
              shift-left: w906 -> [w914]
              stop <- w911 stop-if-true
              # "continue check whether vi is running"
              n341 = property class="VI"(reference=w915, error in=w914) -> (error out=w909:errorcluster, "Exec.State"=w913:T12)  [unwired: 1 out]
              n342 = Wait (ms)(milliseconds to wait=u32 50) -> ()  [unwired: 1 out]
              n343 = Equal?(x=w913, y=T12."Idle") -> (x = y?=w911:bool)
            }
          }
          frame Error {
            # "try again when error"
          }
        }
        n344 = call <vilib>:"Add State(s) to Queue__JKI_lib_State_Machine.vi"("State(s) in Front (\"\")"=w897, "State(s) in (\"\")"=w904) -> ("States Out"=w903:string)  [unwired: 13 in]
      }
      frame "LED: Off" {
        # "set LED to red"
        # "Template Separator\n(You can make a copy of, or modify, this frame)"
        n345 = Unbundle By Name(w920) -> ("LJ Pinout.Red LED"=w919:string, "LJ Pinout.Green LED"=w918:string)
        n346 = call "LabJack_FGV.vi"("Operation(Read)"=enum16{"Write", "Read"}."Read" ("Operation"), "error in (no error)"=w921) -> ("error out"=w928:errorcluster, "Read data"=w927:i32)  [unwired: 8 in]
        n347 = call "LJM_eWriteName.vi"("Handle In"=w927, "Name"=w919, "Value"=0.0, "error in"=w928) -> ("Handle Out"=w925:i32, "error out"=w924:errorcluster)  [unwired: 10 in]
        n348 = call "LJM_eWriteName.vi"("Handle In"=w925, "Name"=w918, "Value"=0.0, "error in"=w924) -> ("error out"=w922:errorcluster)  [unwired: 10 in, 1 out]
        n349 = call <vilib>:"Add State(s) to Queue__JKI_lib_State_Machine.vi"("State(s) in (\"\")"=w932) -> ("States Out"=w931:string)  [unwired: 14 in]
      }
      frame "LED: Green" {
        # "set LED to green"
        # "Template Separator\n(You can make a copy of, or modify, this frame)"
        n350 = Unbundle By Name(w936) -> ("LJ Pinout.Red LED"=w934:string, "LJ Pinout.Green LED"=w935:string)
        n351 = call "LabJack_FGV.vi"("Operation(Read)"=enum16{"Write", "Read"}."Read" ("Operation"), "error in (no error)"=w938) -> ("error out"=w944:errorcluster, "Read data"=w943:i32)  [unwired: 8 in]
        n352 = call "LJM_eWriteName.vi"("Handle In"=w943, "Name"=w934, "Value"=0.0, "error in"=w944) -> ("Handle Out"=w941:i32, "error out"=w940:errorcluster)  [unwired: 10 in]
        n353 = call "LJM_eWriteName.vi"("Handle In"=w941, "Name"=w935, "Value"=9.0, "error in"=w940) -> ("error out"=w937:errorcluster)  [unwired: 10 in, 1 out]
        n354 = call <vilib>:"Add State(s) to Queue__JKI_lib_State_Machine.vi"("State(s) in (\"\")"=w947) -> ("States Out"=w946:string)  [unwired: 14 in]
      }
      frame "---------- Run ----------" {
        # "Template Separator\n(You can make a copy of, or modify, this frame)"
        n355 = call <vilib>:"Add State(s) to Queue__JKI_lib_State_Machine.vi"("State(s) in (\"\")"=w952) -> ("States Out"=w951:string)  [unwired: 14 in]
      }
      frame "Run: CaliIncrement" {
        # "Increment Calibration #\n(You can make a copy of, or modify, this frame)"
        n356 = Unbundle By Name(w954) -> ("IDs.Cali ID"=w956:i8)
        n357 = Increment(x=w956) -> (x+1=w953:i8)
        n358 = Bundle By Name(cluster=w954, "IDs.Cali ID"=w953) -> (w955:T15)
        n359 = call <vilib>:"Add State(s) to Queue__JKI_lib_State_Machine.vi"("State(s) in (\"\")"=w960) -> ("States Out"=w959:string)  [unwired: 14 in]
      }
      frame "Run: BGIncrement" {
        # "Increment BG #\n(You can make a copy of, or modify, this frame)"
        n360 = Unbundle By Name(w961) -> ("IDs.BG ID"=w964:i8)
        n361 = Increment(x=w964) -> (x+1=w963:i8)
        n362 = Bundle By Name(cluster=w961, "IDs.BG ID"=w963) -> (w962:T15)
        n363 = call <vilib>:"Add State(s) to Queue__JKI_lib_State_Machine.vi"("State(s) in (\"\")"=w968) -> ("States Out"=w967:string)  [unwired: 14 in]
      }
      frame "Run: Increment" {
        # "Increase Run# by 1"
        n364 = Unbundle By Name(w973) -> ("IDs.RunID"=w975:i8)
        n365 = Increment(x=w975) -> (x+1=w971:i8)
        n366 = Bundle By Name(cluster=w973, "IDs.RunID"=w971) -> (w974:T15)
        n367 = call "RunIDFGV.vi"("Error In"=w969, "RunID in"=w971) -> ("Error Out"=w970:errorcluster)  [unwired: 8 in, 1 out]
        n368 = call <vilib>:"Add State(s) to Queue__JKI_lib_State_Machine.vi"("State(s) in (\"\")"=w977) -> ("States Out"=w976:string)  [unwired: 14 in]
      }
      frame "Run: Decrement" {
        # "Increase Run# by 1"
        n369 = Unbundle By Name(w982) -> ("IDs.RunID"=w984:i8)
        n370 = Decrement(x=w984) -> (x-1=w980:i8)
        n371 = Bundle By Name(cluster=w982, "IDs.RunID"=w980) -> (w983:T15)
        n372 = call "RunIDFGV.vi"("Error In"=w978, "RunID in"=w980) -> ("Error Out"=w979:errorcluster)  [unwired: 8 in, 1 out]
        n373 = call <vilib>:"Add State(s) to Queue__JKI_lib_State_Machine.vi"("State(s) in (\"\")"=w986) -> ("States Out"=w985:string)  [unwired: 14 in]
      }
      frame "---------- SysConfig ----------" {
        # "Template Separator\n(You can make a copy of, or modify, this frame)"
        n374 = call <vilib>:"Add State(s) to Queue__JKI_lib_State_Machine.vi"("State(s) in (\"\")"=w991) -> ("States Out"=w990:string)  [unwired: 14 in]
      }
      frame "SysConfig: Load LJ Pinout" {
        # "Template Separator\n(You can make a copy of, or modify, this frame)"
        n375 = call <userlib>:"Current VIs Parent Directory__ogtk.vi"() -> ("Parent Directory (+ Relative)"=w1005:path)  [unwired: 5 in]
        n376 = Build Path(base path=w1005, name or relative path="SubVI\\LabJack\\LJ_pin_setting.config") -> (appended path=w1003:path)
        n377 = call "ReadLabjackConfig(SubVI).vi"("error in (no error)"=w1001, "appended path"=w1003) -> ("error out"=w1002:errorcluster, "Utility"=w999:T4)  [unwired: 8 in]
        n378 = Unbundle By Name(w999) -> ("Ch1 Bias"=w998:string, "Ch2 Bias"=w997:string, "Ch3 Bias"=w996:string, "Red LED"=w993:string, "Green LED"=w992:string)
        n379 = global write "GlobalVariables.vi" "LED Green pin"(w992) -> ()
        n380 = global write "GlobalVariables.vi" "LED Red pin"(w993) -> ()
        n381 = global write "GlobalVariables.vi" "Ch1 LJ pin"(w998) -> ()
        n382 = global write "GlobalVariables.vi" "Ch2 LJ pin"(w997) -> ()
        n383 = global write "GlobalVariables.vi" "Ch3 LJ pin"(w996) -> ()
        n384 = Bundle By Name(cluster=w994, "LJ Pinout"=w999) -> (w1000:T15)
        n385 = call <vilib>:"Add State(s) to Queue__JKI_lib_State_Machine.vi"("State(s) in (\"\")"=w1007) -> ("States Out"=w1006:string)  [unwired: 14 in]
      }
      frame "SysConfig: Load 355 PWM" {
        # "Template Separator\n(You can make a copy of, or modify, this frame)"
        n386 = call <userlib>:"Current VIs Parent Directory__ogtk.vi"() -> ("Parent Directory (+ Relative)"=w1025:path)  [unwired: 5 in]
        n387 = Build Path(base path=w1025, name or relative path="SubVI\\LabJack\\PWM_setting_355.config") -> (appended path=w1023:path)
        n388 = call "ReadPWMConfig(SubVI).vi"("error in (no error)"=w1020, "appended path"=w1023) -> ("error out"=w1021:errorcluster, "PWM Setting"=w1019:T24)  [unwired: 8 in]
        n389 = Unbundle By Name(w1019) -> ("DIO_EF_CLOCK1_DIVISOR"=w1016:i16, "DIO_EF_CLOCK1_ROLL_VALUE"=w1015:i32)
        n390 = Multiply(x=w1016, y=w1015) -> (x*y=w1017:i32)
        n391 = Bundle By Name(cluster=w1022, "355 PWM setting"=w1019) -> (w1009:T15)
        n392 = Divide(x=80000000.0, y=w1017) -> (x/y=w1014:dbl)
        "Laser Rep Rate" <- w1014
        n393 = Number To Decimal String(number=w1014) -> (decimal integer string=w1013:string)  [unwired: 1 in]
        n394 = Concatenate Strings("355nm " ("string"), w1013, "Hz" ("string")) -> (w1011:string)
        n395 = property on="355nm Laser toggle" class="Bool (strict)"("Caption.Text"=w1011) -> ()  [unwired: 2 in, 2 out]
        n396 = call <vilib>:"Add State(s) to Queue__JKI_lib_State_Machine.vi"("State(s) in (\"\")"=w1027) -> ("States Out"=w1026:string)  [unwired: 14 in]
      }
      frame "SysConfig: Load AB PWM" {
        # "Template Separator\n(You can make a copy of, or modify, this frame)"
        n397 = call <userlib>:"Current VIs Parent Directory__ogtk.vi"() -> ("Parent Directory (+ Relative)"=w1036:path)  [unwired: 5 in]
        n398 = Build Path(base path=w1036, name or relative path="SubVI\\LabJack\\PWM_setting_AB.config") -> (appended path=w1034:path)
        n399 = call "ReadPWMConfig(SubVI).vi"("error in (no error)"=w1031, "appended path"=w1034) -> ("error out"=w1032:errorcluster, "PWM Setting"=w1030:T24)  [unwired: 8 in]
        n400 = Bundle By Name(cluster=w1028, "AB PWM setting"=w1030) -> (w1033:T15)
        n401 = call <vilib>:"Add State(s) to Queue__JKI_lib_State_Machine.vi"("State(s) in (\"\")"=w1038) -> ("States Out"=w1037:string)  [unwired: 14 in]
      }
      frame "SysConfig: Load AB setting" {
        # "load aming beam setting\n(check frequency, if 0 do nothing, if not zero, config PWM)"
        n402 = call "readAimingBeamSetting.vi"("error in (no error)"=w1056) -> ("error out"=w1051:errorcluster, "Aiming Beam Setting"=w1043:T25)  [unwired: 9 in]
        n403 = Unbundle By Name(w1043) -> ("Default Current"=w1042:dbl)
        n404 = Unbundle By Name(w1043) -> ("Frequency(Hz)"=w1039:u32)
        n405 = Equal To 0?(x=w1039) -> (x = 0?=w1049:bool)
        n406 = Select(t="", s=w1049, f="SysConfig: Load AB PWM" ("State(s) in Front (\"\")")) -> (s? t:f=w1052:string)
        n407 = Number To Decimal String(number=w1039) -> (decimal integer string=w1048:string)  [unwired: 1 in]
        n408 = Number To Decimal String(number=w1042, width (-)=i16 2) -> (decimal integer string=w1041:string)
        n409 = Concatenate Strings("445nm " ("string"), w1048, "Hz " ("string"), w1041, "mA" ("string")) -> (w1047:string)
        n410 = property on="Aiming beam toggle" class="Bool (strict)"("Caption.Text"=w1047) -> ()  [unwired: 2 in, 2 out]
        n411 = case shown="False" w1049 {
          tunnel: w1051 -> [w1064 w1067]
          tunnel: [w1063 w1067] -> w1050
          tunnel: w1039 -> [w1062 _]
          frame False {
            n412 = call "LJ_calculate_PWM_parameters.vi"("Duty Cycle (%)"=u32 10, "Error In"=w1064, "Show Confirmation"=FALSE, "Laser Rep Rate (Hz)"=w1062, "Laser"=enum16{"355nm", "AimingBeam"}."AimingBeam") -> ("Error Out"=w1063:errorcluster)  [unwired: 5 in, 1 out]
          }
          frame True {
          }
        }
        n413 = Bundle By Name(cluster=w1057, "AB Cluster"=w1043) -> (w1058:T15)
        n414 = call <vilib>:"Add State(s) to Queue__JKI_lib_State_Machine.vi"("State(s) in Front (\"\")"=w1052, "State(s) in (\"\")"=w1060) -> ("States Out"=w1059:string)  [unwired: 13 in]
      }
      frame "SysConfig: LoadABVideoSetting" {
        # "Load AB video setting form ini file\n()"
        n415 = call "readVideoConfig.vi"("error in (no error)"=w1071) -> ("error out"=w1072:errorcluster, "Aiming Beam Config"=w1070:T14)  [unwired: 8 in, 1 out]
        n416 = Bundle By Name(cluster=w1068, "VideoConfig"=w1070) -> (w1069:T15)
        n417 = call <vilib>:"Add State(s) to Queue__JKI_lib_State_Machine.vi"("State(s) in (\"\")"=w1075) -> ("States Out"=w1074:string)  [unwired: 14 in]
      }
      frame "---------- SystemStatus ----------" {
        # "Template Separator\n(You can make a copy of, or modify, this frame)"
        n418 = call <vilib>:"Add State(s) to Queue__JKI_lib_State_Machine.vi"("State(s) in (\"\")"=w1080) -> ("States Out"=w1079:string)  [unwired: 14 in]
      }
      frame "SystemStatus: SlowSysStatusMacro" {
        # "store system check time"
        # "Template Separator\n(You can make a copy of, or modify, this frame)"
        n419 = Tick Count (ms)() -> (millisecond timer value=w1083:u32)
        n420 = Bundle By Name(cluster=w1081, "SlowTimer"=w1083) -> (w1082:T15)
        n421 = call <vilib>:"Add State(s) to Queue__JKI_lib_State_Machine.vi"("State(s) in Front (\"\")"="TCP: CheckConnection" ("State(s) in Front (\"\")"), "State(s) in (\"\")"=w1088) -> ("States Out"=w1087:string)  [unwired: 13 in]
      }
      frame "SystemStatus: FastSysStatusMacro" {
        # "store system check time"
        # "Template Separator\n(You can make a copy of, or modify, this frame)"
        n422 = Tick Count (ms)() -> (millisecond timer value=w1091:u32)
        n423 = Bundle By Name(cluster=w1089, "FastTimer"=w1091) -> (w1090:T15)
        n424 = call <vilib>:"Add State(s) to Queue__JKI_lib_State_Machine.vi"("State(s) in Front (\"\")"="355 Laser: CheckPWMStatus\nAimingBeam: GetPWMStatus\n/*355 Laser: CheckControllerStatus" ("State(s) in Front (\"\")"), "State(s) in (\"\")"=w1096) -> ("States Out"=w1095:string)  [unwired: 13 in]
      }
      frame "---------- UI ----------" {
        # "Do not put any code in this frame.\n(It is a separator no-op. You can make a copy of this frame to create a new UI frame)"
        n425 = call <vilib>:"Add State(s) to Queue__JKI_lib_State_Machine.vi"("State(s) in (\"\")"=w1101) -> ("States Out"=w1100:string)  [unwired: 14 in]
      }
      frame "UI: Initialize" {
        w1102 = T8."Disabled and Grayed Out" ("Disabled")
        # "Disable all button on startup"
        # "Initialize the User Interface, here.\n(this is called automatically, by the Macro: Init)"
        n426 = property on="StopButton" class="Bool (strict)"("DisabledEnum"=w1102) -> ()  [unwired: 2 in, 2 out]
        n427 = property on="Sys Reconfig" class="Bool"("DisabledEnum"=w1102) -> ()  [unwired: 2 in, 2 out]
        n428 = property on="StartButton" class="Bool (strict)"("DisabledEnum"=w1102) -> ()  [unwired: 2 in, 2 out]
        n429 = property on="355nm Laser toggle" class="Bool (strict)"("DisabledEnum"=w1102) -> ()  [unwired: 2 in, 2 out]
        n430 = property on="Aiming beam toggle" class="Bool (strict)"("DisabledEnum"=w1102) -> ()  [unwired: 2 in, 2 out]
        n431 = property on="Video Source" class="RadioBtnsControl (strict)"("DisabledEnum"=w1102) -> ()  [unwired: 2 in, 2 out]
        n432 = call <vilib>:"Add State(s) to Queue__JKI_lib_State_Machine.vi"("State(s) in (\"\")"=w1107) -> ("States Out"=w1106:string)  [unwired: 14 in]
      }
      frame "UI: showDisclaimer" {
        # "Show disclamer window.\n(It is a separator no-op. You can make a copy of this frame to create a new UI frame)"
        n433 = call <vilib>:"Application Directory.vi"() -> ("Application Directory"=w1120:path)
        n434 = disable-structure "Diagram Disable Structure" shown="Disabled" {
          frame Disabled {
            n435 = flat-sequence {
              frame #0 {
                n436 = call "disclaimer.vi"() -> ()  [unwired: 12 in]
              }
              frame #1 {
                n437 = Wait (ms)(milliseconds to wait=u32 250) -> ()  [unwired: 1 out]
              }
              frame #2 {
                n438 = call "SoftwareNote.vi"() -> ()  [unwired: 12 in]
              }
            }
          }
          frame Enabled {
          }
        }
        n439 = Build Path(base path=w1120, name or relative path="Disclamer.png") -> (appended path=w1118:path)
        n440 = property on="Disclamer" class="Pict"() -> ("Draw Area Size"=w1116:T26)  [unwired: 2 in, 2 out]
        n441 = call <vilib>:"Read PNG File.vi"("path to PNG file"=w1118) -> ("image data"=w1115:T27)  [unwired: 8 in, 2 out]
        n442 = Unbundle By Name(w1115) -> ("Rectangle.right"=w1113:i16, "Rectangle.bottom"=w1111:i16)
        n443 = Unbundle By Name(w1116) -> ("Width"=w1114:u32, "Height"=w1112:u32)
        n444 = call <vilib>:"Draw Flattened Pixmap.vi"("image data"=w1115) -> ("new picture"=→"Disclamer":picture)  [unwired: 8 in]
        n445 = Divide(x=w1114, y=w1113) -> (x/y=w1110:dbl)
        n446 = Divide(x=w1112, y=w1111) -> (x/y=w1109:dbl)
        n447 = Max & Min(x=w1110, y=w1109) -> (min(x,y)=w1108:dbl)  [unwired: 1 out]
        n448 = property on="Disclamer" class="Pict"("ZoomFactor"=w1108) -> ()  [unwired: 2 in, 2 out]
        n449 = call <vilib>:"Add State(s) to Queue__JKI_lib_State_Machine.vi"("State(s) in (\"\")"=w1125) -> ("States Out"=w1124:string)  [unwired: 14 in]
      }
      frame "UI: DuringAquisition" {
        w1129 = T8."Disabled and Grayed Out" ("Disabled")
        # "Do not put any code in this frame.\n(It is a separator no-op. You can make a copy of this frame to create a new UI frame)"
        n450 = Unbundle By Name(w1128) -> ("bothVidSourceAvail"=w1127:bool)
        n451 = case shown="True" w1127 {
          tunnel: w1129 -> [_ w1135]
          frame False {
          }
          frame True {
            n452 = property on="Video Source" class="RadioBtnsControl (strict)"("DisabledEnum"=w1135) -> ()  [unwired: 2 in, 2 out]
          }
        }
        n453 = property on="StartButton" class="Bool (strict)"("DisabledEnum"=w1129) -> ()  [unwired: 2 in, 2 out]
        n454 = property on="Sys Reconfig" class="Bool"("DisabledEnum"=w1129) -> ()  [unwired: 2 in, 2 out]
        n455 = property on="355nm Laser toggle" class="Bool (strict)"("DisabledEnum"=w1129) -> ()  [unwired: 2 in, 2 out]
        n456 = property on="Aiming beam toggle" class="Bool (strict)"("DisabledEnum"=w1129) -> ()  [unwired: 2 in, 2 out]
        n457 = property on="Quit" class="Bool"("DisabledEnum"=w1129) -> ()  [unwired: 2 in, 2 out]
        n458 = property on="Video Display" class="Bool (strict)"("DisabledEnum"=w1129) -> ()  [unwired: 2 in, 2 out]
        n459 = property on="StopButton" class="Bool (strict)"("DisabledEnum"=T8."Enabled" ("Disabled")) -> ()  [unwired: 2 in, 2 out]
        n460 = call <vilib>:"Add State(s) to Queue__JKI_lib_State_Machine.vi"("State(s) in (\"\")"=w1134) -> ("States Out"=w1133:string)  [unwired: 14 in]
      }
      frame "UI: duringIRFAlign" {
        w1136 = T8."Disabled and Grayed Out" ("Disabled")
        # "Set UI to during iRF alignment\n(It is a separator no-op. You can make a copy of this frame to create a new UI frame)"
        n461 = property on="StartButton" class="Bool (strict)"("DisabledEnum"=w1136) -> ()  [unwired: 2 in, 2 out]
        n462 = property on="Sys Reconfig" class="Bool"("DisabledEnum"=w1136) -> ()  [unwired: 2 in, 2 out]
        n463 = property on="355nm Laser toggle" class="Bool (strict)"("DisabledEnum"=w1136) -> ()  [unwired: 2 in, 2 out]
        n464 = property on="Aiming beam toggle" class="Bool (strict)"("DisabledEnum"=w1136) -> ()  [unwired: 2 in, 2 out]
        n465 = property on="StopButton" class="Bool (strict)"("DisabledEnum"=w1136) -> ()  [unwired: 2 in, 2 out]
        n466 = call <vilib>:"Add State(s) to Queue__JKI_lib_State_Machine.vi"("State(s) in (\"\")"=w1141) -> ("States Out"=w1140:string)  [unwired: 14 in]
      }
      frame "UI: duringBGAcquire" {
        w1142 = T8."Disabled and Grayed Out" ("Disabled")
        # "Do not put any code in this frame.\n(It is a separator no-op. You can make a copy of this frame to create a new UI frame)"
        n467 = property on="StartButton" class="Bool (strict)"("DisabledEnum"=w1142) -> ()  [unwired: 2 in, 2 out]
        n468 = property on="StopButton" class="Bool (strict)"("DisabledEnum"=w1142) -> ()  [unwired: 2 in, 2 out]
        n469 = property on="Sys Reconfig" class="Bool"("DisabledEnum"=w1142) -> ()  [unwired: 2 in, 2 out]
        n470 = property on="355nm Laser toggle" class="Bool (strict)"("DisabledEnum"=w1142) -> ()  [unwired: 2 in, 2 out]
        n471 = property on="Aiming beam toggle" class="Bool (strict)"("DisabledEnum"=w1142) -> ()  [unwired: 2 in, 2 out]
        n472 = call <vilib>:"Add State(s) to Queue__JKI_lib_State_Machine.vi"("State(s) in (\"\")"=w1147) -> ("States Out"=w1146:string)  [unwired: 14 in]
      }
      frame "UI: ReadyForAquisition" {
        w1151 = T8."Enabled" ("Disabled")
        # "Do not put any code in this frame.\n(It is a separator no-op. You can make a copy of this frame to create a new UI frame)"
        n473 = Unbundle By Name(w1150) -> ("System Status.TCP/IP"=w1149:bool, "bothVidSourceAvail"=w1148:bool)
        n474 = property on="StartButton" class="Bool (strict)"("DisabledEnum"=w1151) -> ()  [unwired: 2 in, 2 out]
        n475 = property on="Sys Reconfig" class="Bool"("DisabledEnum"=w1151) -> ()  [unwired: 2 in, 2 out]
        n476 = property on="355nm Laser toggle" class="Bool (strict)"("DisabledEnum"=w1151) -> ()  [unwired: 2 in, 2 out]
        n477 = property on="Aiming beam toggle" class="Bool (strict)"("DisabledEnum"=w1151) -> ()  [unwired: 2 in, 2 out]
        n478 = property on="Quit" class="Bool"("DisabledEnum"=w1151) -> ()  [unwired: 2 in, 2 out]
        n479 = case shown="True" w1148 {
          tunnel: w1151 -> [_ w1157]
          frame False {
          }
          frame True {
            n480 = property on="Video Source" class="RadioBtnsControl (strict)"("DisabledEnum"=w1157) -> ()  [unwired: 2 in, 2 out]
          }
        }
        n481 = case shown="True" w1149 {
          tunnel: w1151 -> [_ w1158]
          frame False {
          }
          frame True {
            n482 = property on="Video Display" class="Bool (strict)"("DisabledEnum"=w1158) -> ()  [unwired: 2 in, 2 out]
          }
        }
        n483 = property on="StopButton" class="Bool (strict)"("DisabledEnum"=T8."Disabled and Grayed Out" ("Disabled")) -> ()  [unwired: 2 in, 2 out]
        n484 = call <vilib>:"Add State(s) to Queue__JKI_lib_State_Machine.vi"("State(s) in (\"\")"=w1156) -> ("States Out"=w1155:string)  [unwired: 14 in]
      }
      frame "UI: Update" {
        # "Do not put any code in this frame.\n(It is a separator no-op. You can make a copy of this frame to create a new UI frame)"
        n485 = Unbundle By Name(w1169) -> ("System Status"=→"System Hardware Connection Status":T2, "IDs.RunID"=→"Run #":i8, "CaseID"=→"Case #":string, "FLImDAQ"=→"FLImDAQ":T20, "SysRunning?"=→"Aquisition Status:":bool, "LJ Pinout"=→"LJ Pinout":T4, "IDs.BG ID"=→"BG #":i8, "IDs.Cali ID"=→"Calibration #":i8, "video source"=→"Visualization PC video source":T1)
        n486 = call <vilib>:"Add State(s) to Queue__JKI_lib_State_Machine.vi"("State(s) in (\"\")"=w1172) -> ("States Out"=w1171:string)  [unwired: 14 in]
      }
      frame "UI: updateVideoToggle" {
        # "Set video toggle based on visualization PC video source.\n(take )"
        n487 = call <vilib>:"Add State(s) to Queue__JKI_lib_State_Machine.vi"("State(s) in (\"\")"=w1177) -> ("States Out"=w1176:string)  [unwired: 14 in]
      }
      frame "UI: Cursor Set" {
        # "Argument"
        # "Set and Unset Cursor Busy.\n(Usage: \"UI: Cursor Set >> Busy|Idle\")"
        n488 = case shown="\"Idle\", Default" w1179 {
          tunnel: w1181 -> [w1186 w1188]
          tunnel: [w1185 w1187] -> w1180
          frame "Idle", Default {
            n489 = call <vilib>:"Unset Busy.vi"("error in (no error)"=w1186) -> ("error out"=w1185:errorcluster)  [unwired: 10 in]
          }
          frame "Busy" {
            n490 = call <vilib>:"Set Busy.vi"("error in (no error)"=w1188) -> ("error out"=w1187:errorcluster)  [unwired: 9 in, 1 out]
          }
        }
        n491 = call <vilib>:"Add State(s) to Queue__JKI_lib_State_Machine.vi"("State(s) in (\"\")"=w1184) -> ("States Out"=w1183:string)  [unwired: 14 in]
      }
      frame "UI: Front Panel State" {
        # "Argument"
        # "Set Front Panel Open or Closed\n(Usage: \"UI: Front Panel State >> Open|Close\")"
        n492 = Unbundle By Name(w1192) -> ("Core.Current VI Reference"=w1191:refnum<vi>)
        n493 = case shown="\"Open\", \"Standard\", Default" w1190 {
          tunnel: w1194 -> [w1202 w1217 w1228 w1241 w1254]
          tunnel: [w1204 w1218 w1230 w1243 w1256] -> w1193
          tunnel: w1191 -> [w1203 w1215 w1229 w1242 w1255]
          frame "Open", "Standard", Default {
            w1197 = T10."Standard" ("State")
            n494 = property on="Property Node" class="VI"(reference=w1203, error in=w1202) -> (reference out=w1200:refnum<vi>, error out=w1201:errorcluster, "FP.State"=w1199:T10)
            n495 = Not Equal?(x=w1199, y=w1197) -> (x != y?=w1198:bool)
            n496 = case shown="True" w1198 {
              tunnel: [w1208 w1210] -> w1204
              tunnel: w1201 -> [w1207 w1210]
              tunnel: w1200 -> [w1206 _]
              tunnel: w1197 -> [w1205 _]
              frame True {
                n497 = invoke on="Invoke Node" class="VI" method="FP.Open"(reference=w1206, error in=w1207, "Activate"=TRUE, "State"=w1205) -> (error out=w1208:errorcluster)  [unwired: 1 in, 4 out]
              }
              frame False {
              }
            }
          }
          frame "Close", "Closed" {
            n498 = property on="Property Node" class="VI"(reference=w1215, error in=w1217) -> (reference out=w1214:refnum<vi>, error out=w1216:errorcluster, "FP.State"=w1212:T10)
            n499 = Not Equal?(x=w1212, y=T10."Closed" ("Front Panel Window:State")) -> (x != y?=w1211:bool)
            n500 = case shown="True" w1211 {
              tunnel: [w1219 w1222] -> w1218
              tunnel: w1216 -> [w1219 w1221]
              tunnel: w1214 -> [_ w1220]
              frame False {
              }
              frame True {
                n501 = invoke on="Invoke Node" class="VI" method="FP.Close"(reference=w1220, error in=w1221) -> (error out=w1222:errorcluster)  [unwired: 1 in, 2 out]
              }
            }
          }
          frame "Hidden", "Hide" {
            w1223 = T10."Hidden" ("State")
            n502 = property on="Property Node" class="VI"(reference=w1229, error in=w1228) -> (reference out=w1226:refnum<vi>, error out=w1227:errorcluster, "FP.State"=w1225:T10)
            n503 = Not Equal?(x=w1225, y=w1223) -> (x != y?=w1224:bool)
            n504 = case shown="True" w1224 {
              tunnel: [w1234 w1235] -> w1230
              tunnel: w1227 -> [w1233 w1235]
              tunnel: w1226 -> [w1232 _]
              tunnel: w1223 -> [w1231 _]
              frame True {
                n505 = invoke on="Invoke Node" class="VI" method="FP.Open"(reference=w1232, error in=w1233, "State"=w1231) -> (error out=w1234:errorcluster)  [unwired: 2 in, 4 out]
              }
              frame False {
              }
            }
          }
          frame "Minimize", "Minimized" {
            w1236 = T10."Minimized" ("State")
            n506 = property on="Property Node" class="VI"(reference=w1242, error in=w1241) -> (reference out=w1239:refnum<vi>, error out=w1240:errorcluster, "FP.State"=w1238:T10)
            n507 = Not Equal?(x=w1238, y=w1236) -> (x != y?=w1237:bool)
            n508 = case shown="True" w1237 {
              tunnel: [w1247 w1248] -> w1243
              tunnel: w1240 -> [w1246 w1248]
              tunnel: w1239 -> [w1245 _]
              tunnel: w1236 -> [w1244 _]
              frame True {
                n509 = invoke on="Invoke Node" class="VI" method="FP.Open"(reference=w1245, error in=w1246, "State"=w1244) -> (error out=w1247:errorcluster)  [unwired: 2 in, 4 out]
              }
              frame False {
              }
            }
          }
          frame "Maximize", "Maximized" {
            w1249 = T10."Maximized" ("State")
            n510 = property on="Property Node" class="VI"(reference=w1255, error in=w1254) -> (reference out=w1252:refnum<vi>, error out=w1253:errorcluster, "FP.State"=w1251:T10)
            n511 = Not Equal?(x=w1251, y=w1249) -> (x != y?=w1250:bool)
            n512 = case shown="True" w1250 {
              tunnel: [w1260 w1261] -> w1256
              tunnel: w1253 -> [w1259 w1261]
              tunnel: w1252 -> [w1258 _]
              tunnel: w1249 -> [w1257 _]
              frame True {
                n513 = invoke on="Invoke Node" class="VI" method="FP.Open"(reference=w1258, error in=w1259, "State"=w1257) -> (error out=w1260:errorcluster)  [unwired: 2 in, 4 out]
              }
              frame False {
              }
            }
          }
        }
        n514 = call <vilib>:"Add State(s) to Queue__JKI_lib_State_Machine.vi"("State(s) in (\"\")"=w1196) -> ("States Out"=w1195:string)  [unwired: 14 in]
      }
      frame "---------- AimingBeam ----------" {
        # "Template Separator\n(You can make a copy of, or modify, this frame)"
        n515 = call <vilib>:"Add State(s) to Queue__JKI_lib_State_Machine.vi"("State(s) in (\"\")"=w1266) -> ("States Out"=w1265:string)  [unwired: 14 in]
      }
      frame "AimingBeam: Initialize" {
        # "set aiming beam button color"
        # "Open COM port for Aiming Beam\n(Require USB connection)"
        n516 = Unbundle By Name(w1268) -> ("AB Cluster.Aiming Beam COM Port"=w1276:refnum<visa-resource-name>)
        n517 = call-poly "VISA Configure Serial Port"("VISA resource name"=w1276, "Enable Termination\nChar (T)"=TRUE ("Enable Termination\nChar (T)"), "baud rate (9600)"=u32 9600, "error in (no error)"=w1273) -> ("error out"=w1272:errorcluster)  [unwired: 10 in, 1 out]
        n518 = Unbundle By Name(w1272) -> ("status"=w1271:bool)
        n519 = Not(x=w1271) -> (.not. x?=w1270:bool)
        n520 = Bundle By Name(cluster=w1268, "System Status.Aiming Beam"=w1270) -> (w1269:T15)
        n521 = call <vilib>:"Add State(s) to Queue__JKI_lib_State_Machine.vi"("State(s) in (\"\")"=w1278) -> ("States Out"=w1277:string)  [unwired: 14 in]
      }
      frame "AimingBeam: Close" {
        # "Close Aiming Beam COM port\n(Require USB connection to Aiming Beam Laser)"
        n522 = Unbundle By Name(w1281) -> ("AB Cluster.Aiming Beam COM Port"=w1285:refnum<visa-resource-name>)
        n523 = VISA Close(VISA resource name=w1285, error in (no error)=w1283) -> (error out=w1284:errorcluster)
        n524 = Bundle By Name(cluster=w1281, "System Status.Aiming Beam"=FALSE) -> (w1282:T15)
        n525 = call <vilib>:"Add State(s) to Queue__JKI_lib_State_Machine.vi"("State(s) in (\"\")"=w1287) -> ("States Out"=w1286:string)  [unwired: 14 in]
      }
      frame "AimingBeam: Set Current" {
        # "Set Aiming Beam Current\n(You can make a copy of, or modify, this frame)"
        n526 = Unbundle By Name(w1302) -> ("AB Cluster.Aiming Beam COM Port"=w1295:refnum<visa-resource-name>, "AB Cluster.Max Current"=w1291:dbl, "AB Cluster.Default Current"=w1293:dbl, "AB Cluster.Min Current"=w1292:dbl)
        n527 = In Range and Coerce(upper limit=w1291, x=w1293, lower limit=w1292) -> (coerced(x)=w1288:dbl)  [unwired: 1 out]
        n528 = Number To Fractional String(number=w1288, precision (6)=i16 2) -> (F-format string=w1296:string)  [unwired: 2 in]
        n529 = Concatenate Strings("slc:", w1296, "\r" ("Carriage Return Constant"), "\n" ("Line Feed Constant")) -> (w1299:string)
        n530 = VISA Write(VISA resource name=w1295, write buffer=w1299, error in (no error)=w1290) -> (error out=w1294:errorcluster)  [unwired: 2 out]
        n531 = call <vilib>:"Add State(s) to Queue__JKI_lib_State_Machine.vi"("State(s) in (\"\")"=w1304) -> ("States Out"=w1303:string)  [unwired: 14 in]
      }
      frame "AimingBeam: Set Status" {
        # "Enable Aiming Beam\n(Usage: \"AimingBeam: Set >> Enable|Disable\")"
        n532 = Unbundle By Name(w1311) -> ("AB Cluster.Aiming Beam COM Port"=w1308:refnum<visa-resource-name>)
        n533 = case shown="\"Enable\"" w1310 {
          tunnel: [w1314 w1318] -> w1309
          frame "Disable", Default {
            n534 = Concatenate Strings("cof", "\r" ("Carriage Return Constant"), "\n" ("Line Feed Constant")) -> (w1314:string)
          }
          frame "Enable" {
            n535 = Concatenate Strings("con", "\r" ("Carriage Return Constant"), "\n" ("Line Feed Constant")) -> (w1318:string)
          }
        }
        n536 = VISA Write(VISA resource name=w1308, write buffer=w1309, error in (no error)=w1306) -> (error out=w1307:errorcluster)  [unwired: 2 out]
        n537 = call <vilib>:"Add State(s) to Queue__JKI_lib_State_Machine.vi"("State(s) in (\"\")"=w1313) -> ("States Out"=w1312:string)  [unwired: 14 in]
      }
      frame "AimingBeam: GetPWMStatus" {
        # "Get aiming beam PWM status\n()"
        n538 = Unbundle By Name(w1326) -> ("AB Cluster.Freq"=w1325:i32, "LJ Pinout.AimingBeam PWM"=w1332:string)
        n539 = Equal To 0?(x=w1325) -> (x = 0?=w1324:bool)
        n540 = call "LabJack_FGV.vi"("Operation(Read)"=enum16{"Write", "Read"}."Read" ("Operation"), "error in (no error)"=w1328) -> ("error out"=w1330:errorcluster, "Read data"=w1331:i32)  [unwired: 8 in]
        n541 = case shown="True" w1324 {
          tunnel: w1332 -> [w1345 _]
          tunnel: [w1343 "DIO_STATE"] -> w1329
          frame False {
            n542 = Concatenate Strings(w1345, "_EF_ENABLE" ("string")) -> (w1343:string)
          }
          frame True {
          }
        }
        n543 = call "LJM_eReadName.vi"("Handle In"=w1331, "Name"=w1329, "error in"=w1330) -> ("Value"=w1323:dbl, "error out"=w1327:errorcluster)  [unwired: 10 in, 1 out]
        n544 = case shown="True" w1324 {
          tunnel: w1323 -> [w1338 w1342]
          tunnel: [w1337 w1339] -> w1322
          frame False {
            n545 = Greater Than 0?(x=w1338) -> (x > 0?=w1337:bool)
          }
          frame True {
            n546 = Number To Boolean Array(number=w1342) -> (Boolean array=w1341:bool[])
            n547 = Index Array(array=w1341, index=3) -> (element=w1339:bool)
          }
        }
        n548 = case shown="False" w1322 {
          frame False {
            # "PWM is off\nset color to dark green"
            n549 = local write "Aiming beam toggle"(FALSE ("Aimging beam")) -> ()
          }
          frame True {
            # "PWM is on\nset color to light green"
            n550 = local write "Aiming beam toggle"(TRUE ("Aimging beam")) -> ()
          }
        }
        n551 = call <vilib>:"Add State(s) to Queue__JKI_lib_State_Machine.vi"("State(s) in (\"\")"=w1336) -> ("States Out"=w1335:string)  [unwired: 14 in]
      }
      frame "---------- 355 Laser ----------" {
        # "Template Separator\n(You can make a copy of, or modify, this frame)"
        n552 = call <vilib>:"Add State(s) to Queue__JKI_lib_State_Machine.vi"("State(s) in (\"\")"=w1353) -> ("States Out"=w1352:string)  [unwired: 14 in]
      }
      frame "355 Laser: Check Dewelling" {
        # "if time laser start time is less than 7.5s before, wait 250ms then check again."
        # "Template Separator\n(You can make a copy of, or modify, this frame)"
        n553 = Unbundle By Name(w1361) -> ("Laser start tic"=w1358:u32)
        n554 = Tick Count (ms)() -> (millisecond timer value=w1359:u32)
        n555 = Subtract(x=w1359, y=w1358) -> (x-y=w1357:u32)
        n556 = Greater?(x=w1357, y=u32 5000) -> (0:w1355:bool)
        n557 = case shown="False" w1355 {
          tunnel: ["355 Laser: Check Dewelling" ""] -> w1354
          frame False {
            n558 = Wait (ms)(milliseconds to wait=u32 250) -> ()  [unwired: 1 out]
          }
          frame True {
          }
        }
        n559 = call <vilib>:"Add State(s) to Queue__JKI_lib_State_Machine.vi"("State(s) in Front (\"\")"=w1354, "State(s) in (\"\")"=w1364) -> ("States Out"=w1363:string)  [unwired: 13 in]
      }
      frame "355 Laser: Laser enable" {
        # "Laser enable/disable\n(Usage: \"LabJack: Laser enable/disable >> 1|0\")"
        n560 = Unbundle By Name(w1371) -> ("LJ Pinout.Laser Start/Stop"=w1375:string, "System Status.355 Laser"=w1369:bool)
        n561 = case shown="False" w1369 {
          tunnel: w1368 -> [w1390 w1391]
          tunnel: w1375 -> [w1384 _]
          tunnel: [w1379 w1391] -> w1373
          tunnel: [w1378 u32 0 ("millisecond timer value")] -> w1370
          frame False {
            n562 = call "LabJack_FGV.vi"("Operation(Read)"=enum16{"Write", "Read"}."Read" ("Operation")) -> ("Read data"=w1386:i32)  [unwired: 9 in, 1 out]
            n563 = call "LJM_eWriteName.vi"("Handle In"=w1386, "Name"=w1384, "Value"=1.0, "error in"=w1390) -> ("Handle Out"=w1385:i32, "error out"=w1383:errorcluster)  [unwired: 10 in]
            n564 = call <userlib>:"Wait (ms)__ogtk.vi"("error in (no error)"=w1383, "milliseconds to wait"=u32 250) -> ("error out"=w1382:errorcluster)  [unwired: 8 in, 1 out]
            n565 = call "LJM_eWriteName.vi"("Handle In"=w1385, "Name"=w1384, "Value"=0.0, "error in"=w1382) -> ("error out"=w1380:errorcluster)  [unwired: 10 in, 1 out]
            n566 = call <userlib>:"Tick Count (ms)__ogtk.vi"("error in (no error)"=w1380) -> ("error out"=w1379:errorcluster, "millisecond timer value"=w1378:u32)  [unwired: 9 in]
          }
          frame True {
          }
        }
        n567 = Bundle By Name(cluster=w1371, "Laser start tic"=w1370) -> (w1372:T15)
        n568 = call <vilib>:"Add State(s) to Queue__JKI_lib_State_Machine.vi"("State(s) in (\"\")"=w1377) -> ("States Out"=w1376:string)  [unwired: 14 in]
      }
      frame "355 Laser: Laser disable" {
        # "Laser enable/disable\n(Usage: \"LabJack: Laser enable/disable >> 1|0\")"
        n569 = Unbundle By Name(w1395) -> ("LJ Pinout.Laser Start/Stop"=w1399:string, "System Status.355 Laser"=w1393:bool)
        n570 = case shown="True" w1393 {
          tunnel: w1400 -> [w1403 w1417]
          tunnel: w1399 -> [_ w1411]
          tunnel: [w1403 w1406] -> w1397
          tunnel: [u32 0 ("millisecond timer value") w1405] -> w1394
          frame False {
          }
          frame True {
            n571 = call "LabJack_FGV.vi"("Operation(Read)"=enum16{"Write", "Read"}."Read" ("Operation")) -> ("Read data"=w1413:i32)  [unwired: 9 in, 1 out]
            n572 = call "LJM_eWriteName.vi"("Handle In"=w1413, "Name"=w1411, "Value"=1.0, "error in"=w1417) -> ("Handle Out"=w1412:i32, "error out"=w1410:errorcluster)  [unwired: 10 in]
            n573 = call <userlib>:"Wait (ms)__ogtk.vi"("error in (no error)"=w1410, "milliseconds to wait"=u32 250) -> ("error out"=w1409:errorcluster)  [unwired: 8 in, 1 out]
            n574 = call "LJM_eWriteName.vi"("Handle In"=w1412, "Name"=w1411, "Value"=0.0, "error in"=w1409) -> ("error out"=w1407:errorcluster)  [unwired: 10 in, 1 out]
            n575 = call <userlib>:"Tick Count (ms)__ogtk.vi"("error in (no error)"=w1407) -> ("error out"=w1406:errorcluster, "millisecond timer value"=w1405:u32)  [unwired: 9 in]
          }
        }
        n576 = Bundle By Name(cluster=w1395, "Laser start tic"=w1394) -> (w1396:T15)
        n577 = call <vilib>:"Add State(s) to Queue__JKI_lib_State_Machine.vi"("State(s) in (\"\")"=w1402) -> ("States Out"=w1401:string)  [unwired: 14 in]
      }
      frame "355 Laser: Dewelling" {
        # "Wait some time (ms)\n(355 Laser: Dewelling >> #)"
        n578 = Fract/Exp String To Number(string=w1421, default (0 dbl)=0) -> (number=w1419:i32)  [unwired: 2 in, 1 out]
        n579 = Wait (ms)(milliseconds to wait=w1419) -> ()  [unwired: 1 out]
        n580 = call <vilib>:"Add State(s) to Queue__JKI_lib_State_Machine.vi"("State(s) in (\"\")"=w1425) -> ("States Out"=w1424:string)  [unwired: 14 in]
      }
      frame "355 Laser: Close" {
        # "Template Separator\n(You can make a copy of, or modify, this frame)"
        n581 = call <vilib>:"Add State(s) to Queue__JKI_lib_State_Machine.vi"("State(s) in Front (\"\")"="355 Laser: CheckControllerStatus\n355 Laser: Laser disable\n355 Laser: Dewelling >>1000", "State(s) in (\"\")"=w1431) -> ("States Out"=w1430:string)  [unwired: 13 in]
      }
      frame "355 Laser: CheckControllerStatus" {
        # "if average < 2, laser no power\nif average 2 < average < 9.3, laser on\nif 9.3<average<10, interlock open, blink indicator\nif average > 10, laser off\n[Covers: REQ30]"
        # "take 10 measuremt and look at average"
        # "Check 355 laser controller status\nBy probing Emisison Lamp negative terminal voltage"
        n582 = Unbundle By Name(w1440) -> ("LJ Pinout.Laser Ready"=w1443:string)
        n583 = call "LabJack_FGV.vi"("Operation(Read)"=enum16{"Write", "Read"}."Read" ("Operation")) -> ("Read data"=w1444:i32)  [unwired: 9 in, 1 out]
        n584 = for {
          N: 20 -> [_]
          tunnel: w1444 -> [w1455]
          tunnel: w1443 -> [w1454]
          shift-right: [w1453] -> w1436
          shift-left: w1442 -> [w1452]
          tunnel: [w1450] -> w1435 mode=indexing
          n585 = call "LJM_eReadName.vi"("Handle In"=w1455, "Name"=w1454, "error in"=w1452) -> ("Value"=w1450:dbl, "error out"=w1453:errorcluster)  [unwired: 10 in, 1 out]
          n586 = Wait (ms)(milliseconds to wait=u32 25) -> ()  [unwired: 1 out]
        }
        n587 = call "checkLaserStatus.vi"("error in (no error)"=w1436, "Laser LED voltage"=w1435) -> ("error out"=w1437:errorcluster, "Interlock open?"=w1432:bool, "Laser on?"=w1434:bool, "Mean voltage"=→"laser EM lamp V":dbl)  [unwired: 6 in]
        n588 = Bundle By Name(cluster=w1440, "System Status.355 Laser"=w1434) -> (w1441:T15)
        n589 = case shown="True" w1432 {
          frame False {
            n590 = property on="355 Laser" class="Bool (strict)"("Blinking"=FALSE) -> ()  [unwired: 2 in, 2 out]
          }
          frame True {
            n591 = property on="355 Laser" class="Bool (strict)"("Blinking"=TRUE) -> ()  [unwired: 2 in, 2 out]
          }
        }
        n592 = call <vilib>:"Add State(s) to Queue__JKI_lib_State_Machine.vi"("State(s) in (\"\")"=w1447) -> ("States Out"=w1446:string)  [unwired: 14 in]
      }
      frame "355 Laser: CheckPWMStatus" {
        # "Check 355 laser PWM status\n(Read LJ DIO#EF_ENABLE register to determine PWM status)"
        n593 = Unbundle By Name(w1465) -> ("LJ Pinout.355 PWM"=w1464:string)
        n594 = call "LabJack_FGV.vi"("Operation(Read)"=enum16{"Write", "Read"}."Read" ("Operation"), "error in (no error)"=w1458) -> ("error out"=w1461:errorcluster, "Read data"=w1462:i32)  [unwired: 8 in]
        n595 = Concatenate Strings(w1464, "_EF_ENABLE" ("string")) -> (w1460:string)
        n596 = call "LJM_eReadName.vi"("Handle In"=w1462, "Name"=w1460, "error in"=w1461) -> ("Value"=w1457:dbl, "error out"=w1459:errorcluster)  [unwired: 10 in, 1 out]
        n597 = Greater Than 0?(x=w1457) -> (x > 0?=w1456:bool)
        n598 = case shown="False" w1456 {
          frame False {
            # "PWM is off\nset color to gray"
            n599 = local write "355nm Laser toggle"(FALSE ("355nm Laser")) -> ()
          }
          frame True {
            # "PWM is on\nset color to light green"
            n600 = local write "355nm Laser toggle"(TRUE ("355nm Laser")) -> ()
          }
        }
        n601 = call <vilib>:"Add State(s) to Queue__JKI_lib_State_Machine.vi"("State(s) in (\"\")"=w1469) -> ("States Out"=w1468:string)  [unwired: 14 in]
      }
      frame "355 Laser: Start" {
        # "Template Separator\n(You can make a copy of, or modify, this frame)"
        n602 = call <vilib>:"Add State(s) to Queue__JKI_lib_State_Machine.vi"("State(s) in Front (\"\")"="LabJack: 355_PWM_Start", "State(s) in (\"\")"=w1477) -> ("States Out"=w1476:string)  [unwired: 13 in]
      }
      frame "355 Laser: Stop" {
        # "Template Separator\n(You can make a copy of, or modify, this frame)"
        n603 = call <vilib>:"Add State(s) to Queue__JKI_lib_State_Machine.vi"("State(s) in Front (\"\")"="LabJack: 355_PWM_Stop", "State(s) in (\"\")"=w1483) -> ("States Out"=w1482:string)  [unwired: 13 in]
      }
      frame "---------- Utility ----------" {
        # "Template Separator\n(You can make a copy of, or modify, this frame)"
        n604 = call <vilib>:"Add State(s) to Queue__JKI_lib_State_Machine.vi"("State(s) in (\"\")"=w1488) -> ("States Out"=w1487:string)  [unwired: 14 in]
      }
      frame "Utility: AquiTimerReset" {
        # "Set Aquisition Timer\n(You can make a copy of, or modify, this frame)"
        n605 = Tick Count (ms)() -> (millisecond timer value=w1491:u32)
        n606 = Bundle By Name(cluster=w1489, "Aquisition Timer"=w1491) -> (w1490:T15)
        n607 = call <vilib>:"Add State(s) to Queue__JKI_lib_State_Machine.vi"("State(s) in (\"\")"=w1495) -> ("States Out"=w1494:string)  [unwired: 14 in]
      }
      frame "Utility: AquiTimerCheck" {
        # "5min to ms"
        # "Set Aquisition Timer\n([Covers: REQ35])"
        n608 = Unbundle By Name(w1503) -> ("Aquisition Timer"=w1501:u32)
        n609 = Tick Count (ms)() -> (millisecond timer value=w1502:u32)
        n610 = Subtract(x=w1502, y=w1501) -> (x-y=w1500:u32)
        n611 = Multiply(x=1000, y=300) -> (x*y=w1497:i32)
        n612 = Greater Or Equal?(x=w1500, y=w1497) -> (x >= y?=w1496:bool)
        n613 = case shown="True" w1496 {
          frame False {
            # "do nothing"
          }
          frame True {
            # "if timed out, stop aquisition"
            n614 = property on="StopButton" class="Bool (strict)"("Val(Sgnl)"=TRUE ("Value (Signaling)")) -> ()  [unwired: 2 in, 2 out]
          }
        }
        n615 = call <vilib>:"Add State(s) to Queue__JKI_lib_State_Machine.vi"("State(s) in (\"\")"=w1507) -> ("States Out"=w1506:string)  [unwired: 14 in]
      }
      frame "Utility: StartBeep" {
        # "Beep\n([Covers: REQ18])"
        n616 = call <vilib>:"Beep.vi"("use system alert? (T)"=FALSE, "duration (msec)"=u32 1000, "frequency (Hz)"=u32 2000) -> ()  [unwired: 9 in]
        n617 = call <vilib>:"Add State(s) to Queue__JKI_lib_State_Machine.vi"("State(s) in (\"\")"=w1516) -> ("States Out"=w1515:string)  [unwired: 14 in]
      }
      frame "Utility: EndBeep" {
        # "Beep\n([Covers: REQ18])"
        n618 = flat-sequence {
          frame #0 {
            n619 = call <vilib>:"Beep.vi"("use system alert? (T)"=FALSE, "duration (msec)"=u32 500, "frequency (Hz)"=u32 2000) -> ()  [unwired: 9 in]
          }
          frame #1 {
            n620 = call <vilib>:"Beep.vi"("use system alert? (T)"=FALSE, "duration (msec)"=u32 500, "frequency (Hz)"=u32 2000) -> ()  [unwired: 9 in]
          }
        }
        n621 = call <vilib>:"Add State(s) to Queue__JKI_lib_State_Machine.vi"("State(s) in (\"\")"=w1521) -> ("States Out"=w1520:string)  [unwired: 14 in]
      }
      frame "Utility: Dewelling" {
        # "Main loop dewell\n(Dewelling >> #)"
        n622 = Fract/Exp String To Number(string=w1531, default (0 dbl)=0) -> (number=w1529:i32)  [unwired: 2 in, 1 out]
        n623 = Wait (ms)(milliseconds to wait=w1529) -> ()  [unwired: 1 out]
        n624 = call <vilib>:"Add State(s) to Queue__JKI_lib_State_Machine.vi"("State(s) in (\"\")"=w1535) -> ("States Out"=w1534:string)  [unwired: 14 in]
      }
      frame "---------- SysLog ----------" {
        # "Template Separator\n(You can make a copy of, or modify, this frame)"
        n625 = call <vilib>:"Add State(s) to Queue__JKI_lib_State_Machine.vi"("State(s) in (\"\")"=w1540) -> ("States Out"=w1539:string)  [unwired: 14 in]
      }
      frame "SysLog: OpenLogFile" {
        # "Template Separator\n(You can make a copy of, or modify, this frame)"
        n626 = call <vilib>:"Add State(s) to Queue__JKI_lib_State_Machine.vi"("State(s) in (\"\")"=w1545) -> ("States Out"=w1544:string)  [unwired: 14 in]
      }
      frame "---------- TCP ----------" {
        # "Template Separator\n(You can make a copy of, or modify, this frame)"
        n627 = call <vilib>:"Add State(s) to Queue__JKI_lib_State_Machine.vi"("State(s) in (\"\")"=w1550) -> ("States Out"=w1549:string)  [unwired: 14 in]
      }
      frame "TCP: InitializeNew" {
        # "if unsuccessful and count <10, increament count \nand try again"
        # "Initialize TCP connection to aimging beam computer\n(You can make a copy of, or modify, this frame)"
        n628 = TCP Create Listener(10:u16 2100 ("port"), 11:"RTLT" ("service name")) -> (0:w1556:errorcluster, 3:w1557:refnum<k5>)  [unwired: 3 in, 1 out]
        n629 = call <userlib>:"Tick Count (ms)__ogtk.vi"("error in (no error)"=w1556) -> ("millisecond timer value"=w1554:u32)  [unwired: 9 in, 1 out]
        n630 = while {
          tunnel: w1557 -> [w1583]
          tunnel: w1556 -> [w1582]
          tunnel: [w1573] -> w1562
          tunnel: [w1570] -> w1551
          i -> [w1579]
          stop <- w1570 stop-if-true
          n631 = TCP Wait On Listener(8:w1582, 9:100 ("timeout ms (wait forever: -1)"), 11:w1583) -> (0:w1580:errorcluster, 4:w1577:refnum<k5>)  [unwired: 1 in, 3 out]
          n632 = Less Or Equal?(x=50, y=w1579) -> (x <= y?=w1576:bool)
          n633 = case shown="No Error" w1580 {
            selector: w1580 -> [w1593 w1603]
            tunnel: w1577 -> [w1594 _]
            tunnel: [errorcluster {"status"=TRUE, "code"=0, "source"=""} ("No error") w1604] -> w1572
            tunnel: [w1585 FALSE ("TCP connected?")] -> w1573
            frame No Error {
              # "connection is ready, read data"
              n634 = TCP Read(connection ID=w1594, bytes to read=512, error in (no error)=w1593, 7:T13."CRLF" ("mode (standard)"), 9:5000 ("timeout ms (25000)")) -> (connection ID out=w1587:refnum<k5>, data out=w1589:string, error out=w1586:errorcluster)
              n635 = Concatenate Strings("alive" ("string"), "\r\n" ("End of Line Constant")) -> (w1590:string)
              n636 = Equal?(x=w1590, y=w1589) -> (x = y?=w1588:bool)
              n637 = case shown="False" w1588 {
                tunnel: w1587 -> [_ w1599]
                tunnel: w1586 -> [_ _]
                tunnel: [FALSE ("TCP connected?") TRUE ("TCP connected?")] -> w1585
                frame False {
                }
                frame True {
                  n638 = call "TcpIDFGV.vi"("action"=enum16{"write", "read"}."write", "connection ID in"=w1599) -> ()  [unwired: 8 in, 2 out]
                }
              }
            }
            frame Error {
              # "connection not ready, keep waiting"
              n639 = Unbundle By Name(w1603) -> ("code"=w1605:i32)
              n640 = case shown="56" w1605 {
                tunnel: w1603 -> [w1606 _]
                tunnel: [w1606 w1607] -> w1604
                frame Default {
                }
                frame 56 {
                  w1607 = errorcluster {"status"=FALSE, "code"=0, "source"=""}  # No error
                }
              }
            }
          }
          n641 = Select(t=errorcluster {"status"=TRUE, "code"=5001, "source"=""} ("error in (no error)"), s=w1576, f=errorcluster {"status"=FALSE, "code"=0, "source"=""} ("error in (no error)")) -> (s? t:f=w1571:errorcluster)
          n642 = Merge Errors(w1572, w1571) -> (w1570:errorcluster)
        }
        n643 = call <userlib>:"Tick Count (ms)__ogtk.vi"("error in (no error)"=w1551) -> ("error out"=w1552:errorcluster, "millisecond timer value"=w1555:u32)  [unwired: 9 in]
        n644 = Unbundle By Name(w1552) -> ("code"=w1561:i32)
        n645 = Bundle By Name(cluster=w1563, "System Status.TCP/IP"=w1562, "listener ID"=w1557) -> (w1567:T15)
        n646 = global write "GlobalVariables.vi" "TCP connected?"(w1562) -> ()
        n647 = Equal To 0?(x=w1561) -> (x = 0?=w1560:bool)
        n648 = Subtract(x=w1555, y=w1554) -> (x-y=→"TCP wait time(ms)":u32)
        n649 = Select(t=errorcluster {"status"=FALSE, "code"=0, "source"=""} ("error in (no error)"), s=w1560, f=w1552) -> (s? t:f=w1558:errorcluster)
        n650 = call <vilib>:"Add State(s) to Queue__JKI_lib_State_Machine.vi"("State(s) in (\"\")"=w1569) -> ("States Out"=w1568:string)  [unwired: 14 in]
      }
      frame "TCP: checkSource" {
        # "Check visualization PC video source\n(send !video_source message, listen for response, then parse it to binary mask)"
        n651 = Unbundle By Name(w1614) -> ("System Status.TCP/IP"=w1617:bool)
        n652 = case shown="True" w1617 {
          tunnel: w1616 -> [w1622 w1645]
          tunnel: [w1622 w1629] -> w1615
          tunnel: [w1621 w1634] -> w1612
          tunnel: [w1621 w1632] -> w1611
          tunnel: [w1621 w1633] -> w1610
          tunnel: [w1621 w1631] -> w1609
          tunnel: [w1621 w1623] -> w1608
          frame False {
            w1621 = FALSE
          }
          frame True {
            n653 = call "TcpIDFGV.vi"("Error In"=w1645, "action"=enum16{"write", "read"}."read") -> ("Error Out"=w1642:errorcluster, "connection ID out"=w1644:refnum<k5>)  [unwired: 8 in]
            n654 = call "TCP_WriteRead.vi"("error in (no error)"=w1642, "data in"="!video_source", "connectin ID in"=w1644) -> ("error out"=w1639:errorcluster, "data out"=w1641:string)  [unwired: 4 in, 1 out]
            n655 = Scan From String(format string="!video_source:%d", input string=w1641, error in=w1639) -> (error out=w1630:errorcluster, output 1=w1628:i32)  [unwired: 2 in, 2 out]
            n656 = case shown="5..7, 9..11, 13..15" w1628 {
              tunnel: w1630 -> [_ _ _ _]
              tunnel: [errorcluster {"status"=TRUE, "code"=5007, "source"="Visualization PC"} ("error out") errorcluster {"status"=FALSE, "code"=0, "source"=""} ("error out") errorcluster {"status"=FALSE, "code"=0, "source"=""} ("error out") errorcluster {"status"=FALSE, "code"=0, "source"=""} ("error out")] -> w1629
              tunnel: [FALSE FALSE FALSE TRUE] -> w1623
              frame 0, Default {
                # "No video source available or default"
                n657 = property on="Video Source" class="RadioBtnsControl (strict)"("DisabledEnum"=T8."Disabled and Grayed Out" ("Disabled")) -> ()  [unwired: 2 in, 2 out]
              }
              frame 1..3 {
                # "one or both camera available"
                n658 = local write "Video Source"(enum32{"Camera", "FrameGrabber"}."Camera" ("Video Source")) -> ()
                n659 = property on="Video Source" class="RadioBtnsControl (strict)"("DisabledEnum"=T8."Disabled and Grayed Out" ("Disabled")) -> ()  [unwired: 2 in, 2 out]
              }
              frame 4, 8, 12 {
                # "one or both frame grabber available"
                n660 = local write "Video Source"(enum32{"Camera", "FrameGrabber"}."FrameGrabber" ("Video Source")) -> ()
                n661 = property on="Video Source" class="RadioBtnsControl (strict)"("DisabledEnum"=T8."Disabled and Grayed Out" ("Disabled")) -> ()  [unwired: 2 in, 2 out]
              }
              frame 5..7, 9..11, 13..15 {
                n662 = property on="Video Source" class="RadioBtnsControl (strict)"("DisabledEnum"=T8."Enabled" ("Disabled")) -> ()  [unwired: 2 in, 2 out]
              }
            }
            n663 = Integer to Fixed-Point Cast(fixed-point type=fxp<+,4,4> 0.0, integer=w1628) -> (fixed-point=w1627:fxp<+,4,4>)
            n664 = Number To Boolean Array(number=w1627) -> (Boolean array=w1625:bool[])
            n665 = Reverse 1D Array(array=w1625) -> (reversed array=w1624:bool[])
            n666 = Index Array(array=w1624, index=0) -> (element=w1634:bool)
            n667 = Index Array(array=w1624, index=1) -> (element=w1632:bool)
            n668 = Index Array(array=w1624, index=2) -> (element=w1633:bool)
            n669 = Index Array(array=w1624, index=3) -> (element=w1631:bool)
          }
        }
        n670 = Bundle By Name(cluster=w1614, "video source.Main Frame Grabber"=w1612, "video source.Side Frame Grabber"=w1611, "video source.Main Camera"=w1610, "video source.Side Camera"=w1609, "bothVidSourceAvail"=w1608) -> (w1613:T15)
        n671 = call <vilib>:"Add State(s) to Queue__JKI_lib_State_Machine.vi"("State(s) in (\"\")"=w1620) -> ("States Out"=w1619:string)  [unwired: 14 in]
      }
      frame "TCP: SyncTime" {
        # "Template Separator\n(You can make a copy of, or modify, this frame)"
        n672 = Unbundle By Name(w1662) -> ("System Status.TCP/IP"=w1661:bool)
        n673 = case shown="True" w1661 {
          tunnel: w1663 -> [_ w1671]
          frame False {
          }
          frame True {
            n674 = call "TcpIDFGV.vi"("Error In"=w1671, "action"=enum16{"write", "read"}."read") -> ("Error Out"=w1670:errorcluster, "connection ID out"=w1667:refnum<k5>)  [unwired: 8 in]
            n675 = call <userlib>:"Tick Count (ms)__ogtk.vi"("error in (no error)"=w1670) -> ("error out"=w1669:errorcluster, "millisecond timer value"=w1668:u32)  [unwired: 9 in]
            n676 = while {
              tunnel: w1669 -> [w1691]
              tunnel: w1667 -> [w1690]
              tunnel: w1668 -> [w1679]
              stop <- w1674 stop-if-true
              n677 = Concatenate Strings("latencycheck" ("string"), "\r\n" ("End of Line Constant")) -> (w1686:string)
              n678 = TCP Read(connection ID=w1690, bytes to read=512, error in (no error)=w1691, 7:T13."CRLF" ("mode (standard)"), 9:2000 ("timeout ms (25000)")) -> (connection ID out=w1683:refnum<k5>, data out=w1681:string, error out=w1673:errorcluster)
              n679 = Tick Count (ms)() -> (millisecond timer value=w1680:u32)
              n680 = Subtract(x=w1680, y=w1679) -> (x-y=w1678:u32)
              n681 = Equal?(x=w1681, y=w1686) -> (x = y?=w1682:bool)
              n682 = case shown="True" w1682 {
                tunnel: w1683 -> [_ w1704]
                tunnel: w1681 -> [w1696 _]
                tunnel: [w1692 FALSE] -> w1676
                tunnel: w1673 -> [_ w1698]
                frame False {
                  n683 = Concatenate Strings("synctimer" ("string"), "\r\n" ("End of Line Constant")) -> (w1693:string)
                  n684 = Equal?(x=w1696, y=w1693) -> (x = y?=w1692:bool)
                  "Sync Success?" <- w1692
                }
                frame True {
                  n685 = Concatenate Strings("latencycheck:" ("string"), "\r\n" ("End of Line Constant")) -> (w1703:string)
                  n686 = TCP Write(connection ID=w1704, data in=w1703, error in (no error)=w1698, 9:1000 ("timeout ms (25000)")) -> (error out=w1697:errorcluster)  [unwired: 2 out]
                  n687 = call <vilib>:"Clear Errors.vi"("error in (no error)"=w1697) -> ()  [unwired: 5 in, 2 out]
                }
              }
              n688 = Greater?(x=w1678, y=u32 10000 ("x-y")) -> (0:w1675:bool)
              n689 = Or(x=w1676, y=w1675) -> (x .or. y?=w1674:bool)
            }
          }
        }
        n690 = call <vilib>:"Add State(s) to Queue__JKI_lib_State_Machine.vi"("State(s) in (\"\")"=w1666) -> ("States Out"=w1665:string)  [unwired: 14 in]
      }
      frame "TCP: SendSettingMacro" {
        # "Template Separator\n(You can make a copy of, or modify, this frame)"
        n691 = Unbundle By Name(w1708) -> ("System Status.TCP/IP"=w1707:bool)
        n692 = case shown="True" w1707 {
          tunnel: ["" ("Empty String Constant") "TCP: sendSubjectID\nTCP: sendScaleBarSetting\nTCP: sendScaleMaxMin\nTCP: sendDeconChannel\nTCP: sendANSI\nTCP: sendRadius\nTCP: send3Dsetting\nTCP: sendFirefly\nTCP: sendPentero"] -> w1706
          frame False {
          }
          frame True {
          }
        }
        n693 = call <vilib>:"Add State(s) to Queue__JKI_lib_State_Machine.vi"("State(s) in Front (\"\")"=w1706, "State(s) in (\"\")"=w1711) -> ("States Out"=w1710:string)  [unwired: 13 in]
      }
      frame "TCP: sendRunNum" {
        # "Send run number to AB PC\n(You can make a copy of, or modify, this frame)"
        n694 = Unbundle By Name(w1718) -> ("System Status.TCP/IP"=w1715:bool, "IDs.RunID"=w1719:i8)
        n695 = Increment(x=w1719) -> (x+1=w1714:i8)
        n696 = case shown="True" w1715 {
          tunnel: w1714 -> [_ w1733]
          tunnel: [w1723 w1725] -> w1717
          tunnel: w1716 -> [w1723 w1724]
          frame False {
          }
          frame True {
            n697 = Number To Decimal String(number=w1733, width (-)=i16 3) -> (decimal integer string=w1728:string)
            n698 = call "TcpIDFGV.vi"("Error In"=w1724, "action"=enum16{"write", "read"}."read") -> ("Error Out"=w1726:errorcluster, "connection ID out"=w1730:refnum<k5>)  [unwired: 8 in]
            n699 = Concatenate Strings("!run:", w1728) -> (w1727:string)
            n700 = call "TCP_WriteRead.vi"("error in (no error)"=w1726, "data in"=w1727, "connectin ID in"=w1730) -> ("error out"=w1725:errorcluster)  [unwired: 4 in, 2 out]
          }
        }
        n701 = call <vilib>:"Add State(s) to Queue__JKI_lib_State_Machine.vi"("State(s) in (\"\")"=w1722) -> ("States Out"=w1721:string)  [unwired: 14 in]
      }
      frame "TCP: sendVideoSource" {
        # "Send video source \n(You can make a copy of, or modify, this frame)"
        n702 = Unbundle By Name(w1735) -> ("System Status.TCP/IP"=w1734:bool)
        n703 = case shown="True" w1734 {
          tunnel: [w1741 w1743] -> w1737
          tunnel: w1736 -> [w1741 w1742]
          frame False {
          }
          frame True {
            n704 = case shown="\"Camera\", Default" "Video Source" {
              tunnel: [0 1] -> w1748
              frame "Camera", Default {
              }
              frame "FrameGrabber" {
              }
            }
            n705 = call "TcpIDFGV.vi"("Error In"=w1742, "action"=enum16{"write", "read"}."read") -> ("Error Out"=w1744:errorcluster, "connection ID out"=w1750:refnum<k5>)  [unwired: 8 in]
            n706 = Number To Decimal String(number=w1748) -> (decimal integer string=w1746:string)  [unwired: 1 in]
            n707 = Concatenate Strings("!invivo:" ("data in"), w1746) -> (w1745:string)
            n708 = call "TCP_WriteRead.vi"("error in (no error)"=w1744, "data in"=w1745, "connectin ID in"=w1750) -> ("error out"=w1743:errorcluster)  [unwired: 4 in, 2 out]
          }
        }
        n709 = call <vilib>:"Add State(s) to Queue__JKI_lib_State_Machine.vi"("State(s) in (\"\")"=w1740) -> ("States Out"=w1739:string)  [unwired: 14 in]
      }
      frame "TCP: startRun" {
        # "Template Separator\n(You can make a copy of, or modify, this frame)"
        n710 = Unbundle By Name(w1755) -> ("System Status.TCP/IP"=w1754:bool)
        n711 = case shown="True" w1754 {
          tunnel: [w1761 w1763] -> w1757
          tunnel: w1756 -> [w1761 w1762]
          frame False {
          }
          frame True {
            n712 = call "TcpIDFGV.vi"("Error In"=w1762, "action"=enum16{"write", "read"}."read") -> ("Error Out"=w1764:errorcluster, "connection ID out"=w1765:refnum<k5>)  [unwired: 8 in]
            n713 = call "TCP_WriteRead.vi"("error in (no error)"=w1764, "data in"="!acquire:1", "connectin ID in"=w1765) -> ("error out"=w1763:errorcluster)  [unwired: 4 in, 2 out]
          }
        }
        n714 = call <vilib>:"Add State(s) to Queue__JKI_lib_State_Machine.vi"("State(s) in (\"\")"=w1760) -> ("States Out"=w1759:string)  [unwired: 14 in]
      }
      frame "TCP: stopRun" {
        # "Send stop run to AB PC\n(You can make a copy of, or modify, this frame)"
        n715 = Unbundle By Name(w1769) -> ("System Status.TCP/IP"=w1768:bool)
        n716 = case shown="True" w1768 {
          tunnel: [w1775 w1777] -> w1771
          tunnel: w1770 -> [w1775 w1776]
          frame False {
            # "if not connected, do nothing"
          }
          frame True {
            # "If TCP connected, send stop run"
            n717 = call "TcpIDFGV.vi"("Error In"=w1776, "action"=enum16{"write", "read"}."read") -> ("Error Out"=w1778:errorcluster, "connection ID out"=w1780:refnum<k5>)  [unwired: 8 in]
            n718 = call "TCP_WriteRead.vi"("error in (no error)"=w1778, "data in"="!acquire:0", "connectin ID in"=w1780) -> ("error out"=w1777:errorcluster)  [unwired: 4 in, 2 out]
          }
        }
        n719 = call <vilib>:"Add State(s) to Queue__JKI_lib_State_Machine.vi"("State(s) in (\"\")"=w1774) -> ("States Out"=w1773:string)  [unwired: 14 in]
      }
      frame "TCP: CheckConnection" {
        # "Check TCP/IP connection statuse\n(If connection is lost, throw error)"
        n720 = Unbundle By Name(w1783) -> ("System Status.TCP/IP"=w1782:bool)
        n721 = case shown="True" w1782 {
          frame False {
          }
          frame True {
            # "If TCP/IP is true check, otherwise skip"
          }
        }
        n722 = call <vilib>:"Add State(s) to Queue__JKI_lib_State_Machine.vi"("State(s) in (\"\")"=w1787) -> ("States Out"=w1786:string)  [unwired: 14 in]
      }
      frame "TCP: sendSubjectID" {
        # "Send subject ID"
        n723 = Unbundle By Name(w1789) -> ("System Status.TCP/IP"=w1788:bool, "CaseID"=w1792:string)
        n724 = case shown="True" w1788 {
          tunnel: w1792 -> [_ w1803]
          tunnel: [w1796 w1798] -> w1791
          tunnel: w1790 -> [w1796 w1797]
          frame False {
          }
          frame True {
            n725 = call "TcpIDFGV.vi"("Error In"=w1797, "action"=enum16{"write", "read"}."read") -> ("Error Out"=w1799:errorcluster, "connection ID out"=w1801:refnum<k5>)  [unwired: 8 in]
            n726 = Concatenate Strings("!subject:", w1803) -> (w1800:string)
            n727 = call "TCP_WriteRead.vi"("error in (no error)"=w1799, "data in"=w1800, "connectin ID in"=w1801) -> ("error out"=w1798:errorcluster)  [unwired: 4 in, 2 out]
          }
        }
        n728 = call <vilib>:"Add State(s) to Queue__JKI_lib_State_Machine.vi"("State(s) in (\"\")"=w1795) -> ("States Out"=w1794:string)  [unwired: 14 in]
      }
      frame "TCP: sendScaleBarSetting" {
        # "Template Separator\n(You can make a copy of, or modify, this frame)"
        n729 = Unbundle By Name(w1807) -> ("System Status.TCP/IP"=w1805:bool, "VideoConfig.Scale Bar"=w1806:bool)
        n730 = case shown="True" w1805 {
          tunnel: [w1813 w1822] -> w1809
          tunnel: w1808 -> [w1813 w1821]
          tunnel: w1806 -> [_ w1820]
          frame False {
          }
          frame True {
            n731 = Boolean To (0,1)(Boolean=w1820) -> (0, 1=w1819:i16)
            n732 = call "TcpIDFGV.vi"("Error In"=w1821, "action"=enum16{"write", "read"}."read") -> ("Error Out"=w1823:errorcluster, "connection ID out"=w1824:refnum<k5>)  [unwired: 8 in]
            n733 = Number To Fractional String(number=w1819, width (-)=i16 1, precision (6)=i16 0) -> (F-format string=w1817:string)  [unwired: 1 in]
            n734 = Concatenate Strings("!autocolor:" ("data in"), w1817) -> (w1815:string)
            n735 = call "TCP_WriteRead.vi"("error in (no error)"=w1823, "data in"=w1815, "connectin ID in"=w1824) -> ("error out"=w1822:errorcluster)  [unwired: 4 in, 2 out]
          }
        }
        n736 = call <vilib>:"Add State(s) to Queue__JKI_lib_State_Machine.vi"("State(s) in (\"\")"=w1812) -> ("States Out"=w1811:string)  [unwired: 14 in]
      }
      frame "TCP: sendScaleMaxMin" {
        # "Send scale bar max and min to AB PC\n(You can make a copy of, or modify, this frame)"
        n737 = Unbundle By Name(w1829) -> ("System Status.TCP/IP"=w1826:bool, "VideoConfig.Scale Low"=w1828:dbl, "VideoConfig.Scale High"=w1827:dbl)
        n738 = case shown="True" w1826 {
          tunnel: [w1835 w1848] -> w1831
          tunnel: w1830 -> [w1835 w1847]
          tunnel: w1828 -> [_ w1846]
          tunnel: w1827 -> [_ w1837]
          frame False {
          }
          frame True {
            n739 = call "TcpIDFGV.vi"("Error In"=w1847, "action"=enum16{"write", "read"}."read") -> ("Error Out"=w1849:errorcluster, "connection ID out"=w1850:refnum<k5>)  [unwired: 8 in]
            n740 = Number To Fractional String(number=w1846, width (-)=i16 4, precision (6)=i16 2) -> (F-format string=w1842:string)  [unwired: 1 in]
            n741 = Number To Fractional String(number=w1837, width (-)=i16 4, precision (6)=i16 2) -> (F-format string=w1838:string)  [unwired: 1 in]
            n742 = Concatenate Strings("!color:" ("string"), w1842, ";" ("string"), w1838) -> (w1836:string)
            n743 = call "TCP_WriteRead.vi"("error in (no error)"=w1849, "data in"=w1836, "connectin ID in"=w1850) -> ("error out"=w1848:errorcluster)  [unwired: 4 in, 2 out]
          }
        }
        n744 = call <vilib>:"Add State(s) to Queue__JKI_lib_State_Machine.vi"("State(s) in (\"\")"=w1834) -> ("States Out"=w1833:string)  [unwired: 14 in]
      }
      frame "TCP: sendDeconChannel" {
        # "Send Decon channel\n(You can make a copy of, or modify, this frame)"
        n745 = Unbundle By Name(w1853) -> ("System Status.TCP/IP"=w1852:bool)
        n746 = case shown="True" w1852 {
          tunnel: [w1859 w1864] -> w1855
          tunnel: w1854 -> [w1859 w1863]
          frame False {
          }
          frame True {
            n747 = local read "DeconChannel"() -> (w1862:i8)
            n748 = Increment(x=w1862) -> (x+1=w1861:i8)
            n749 = Number To Decimal String(number=w1861) -> (decimal integer string=w1860:string)  [unwired: 1 in]
            n750 = call "TcpIDFGV.vi"("Error In"=w1863, "action"=enum16{"write", "read"}."read") -> ("Error Out"=w1865:errorcluster, "connection ID out"=w1868:refnum<k5>)  [unwired: 8 in]
            n751 = Concatenate Strings("!channel:", w1860) -> (w1866:string)
            n752 = call "TCP_WriteRead.vi"("error in (no error)"=w1865, "data in"=w1866, "connectin ID in"=w1868) -> ("error out"=w1864:errorcluster)  [unwired: 4 in, 2 out]
          }
        }
        n753 = call <vilib>:"Add State(s) to Queue__JKI_lib_State_Machine.vi"("State(s) in (\"\")"=w1858) -> ("States Out"=w1857:string)  [unwired: 14 in]
      }
      frame "TCP: sendANSI" {
        # "Template Separator\n(You can make a copy of, or modify, this frame)"
        n754 = Unbundle By Name(w1872) -> ("System Status.TCP/IP"=w1870:bool, "VideoConfig.ANSI"=w1871:dbl)
        n755 = case shown="True" w1870 {
          tunnel: [w1878 w1884] -> w1874
          tunnel: w1873 -> [w1878 w1883]
          tunnel: w1871 -> [_ w1882]
          frame False {
          }
          frame True {
            n756 = Number To Fractional String(number=w1882) -> (F-format string=w1880:string)  [unwired: 3 in]
            n757 = call "TcpIDFGV.vi"("Error In"=w1883, "action"=enum16{"write", "read"}."read") -> ("Error Out"=w1885:errorcluster, "connection ID out"=w1886:refnum<k5>)  [unwired: 8 in]
            n758 = Concatenate Strings("!ansi:" ("data in"), w1880) -> (w1879:string)
            n759 = call "TCP_WriteRead.vi"("error in (no error)"=w1885, "data in"=w1879, "connectin ID in"=w1886) -> ("error out"=w1884:errorcluster)  [unwired: 4 in, 2 out]
          }
        }
        n760 = call <vilib>:"Add State(s) to Queue__JKI_lib_State_Machine.vi"("State(s) in (\"\")"=w1877) -> ("States Out"=w1876:string)  [unwired: 14 in]
      }
      frame "TCP: sendRadius" {
        # "Send drawing radius to AB PC\n(You can make a copy of, or modify, this frame)"
        n761 = Unbundle By Name(w1890) -> ("System Status.TCP/IP"=w1888:bool, "VideoConfig.Radius"=w1889:dbl)
        n762 = case shown="True" w1888 {
          tunnel: [w1896 w1902] -> w1892
          tunnel: w1891 -> [w1896 w1901]
          tunnel: w1889 -> [_ w1900]
          frame False {
          }
          frame True {
            n763 = Number To Fractional String(number=w1900) -> (F-format string=w1899:string)  [unwired: 3 in]
            n764 = Concatenate Strings("!radius:" ("data in"), w1899) -> (w1897:string)
            n765 = call "TcpIDFGV.vi"("Error In"=w1901, "action"=enum16{"write", "read"}."read") -> ("Error Out"=w1903:errorcluster, "connection ID out"=w1904:refnum<k5>)  [unwired: 8 in]
            n766 = call "TCP_WriteRead.vi"("error in (no error)"=w1903, "data in"=w1897, "connectin ID in"=w1904) -> ("error out"=w1902:errorcluster)  [unwired: 4 in, 2 out]
          }
        }
        n767 = call <vilib>:"Add State(s) to Queue__JKI_lib_State_Machine.vi"("State(s) in (\"\")"=w1895) -> ("States Out"=w1894:string)  [unwired: 14 in]
      }
      frame "TCP: send3Dsetting" {
        # "Send 3D setting to AB computer\n(You can make a copy of, or modify, this frame)"
        n768 = Unbundle By Name(w1908) -> ("System Status.TCP/IP"=w1906:bool, "VideoConfig.3D?"=w1907:bool)
        n769 = case shown="True" w1906 {
          tunnel: [w1914 w1921] -> w1910
          tunnel: w1909 -> [w1914 w1920]
          tunnel: w1907 -> [_ w1919]
          frame False {
          }
          frame True {
            n770 = Boolean To (0,1)(Boolean=w1919) -> (0, 1=w1918:i16)
            n771 = Number To Fractional String(number=w1918) -> (F-format string=w1917:string)  [unwired: 3 in]
            n772 = call "TcpIDFGV.vi"("Error In"=w1920, "action"=enum16{"write", "read"}."read") -> ("Error Out"=w1922:errorcluster, "connection ID out"=w1923:refnum<k5>)  [unwired: 8 in]
            n773 = Concatenate Strings("!3dset:" ("data in"), w1917) -> (w1915:string)
            n774 = call "TCP_WriteRead.vi"("error in (no error)"=w1922, "data in"=w1915, "connectin ID in"=w1923) -> ("error out"=w1921:errorcluster)  [unwired: 4 in, 2 out]
          }
        }
        n775 = call <vilib>:"Add State(s) to Queue__JKI_lib_State_Machine.vi"("State(s) in (\"\")"=w1913) -> ("States Out"=w1912:string)  [unwired: 14 in]
      }
      frame "TCP: sendFirefly" {
        # "Template Separator\n(You can make a copy of, or modify, this frame)"
        n776 = Unbundle By Name(w1926) -> ("System Status.TCP/IP"=w1925:bool)
        n777 = case shown="False" w1925 {
          tunnel: [w1932 w1934] -> w1928
          tunnel: w1927 -> [w1932 w1933]
          frame False {
          }
          frame True {
            n778 = call "TcpIDFGV.vi"("Error In"=w1933, "action"=enum16{"write", "read"}."read") -> ("Error Out"=w1935:errorcluster, "connection ID out"=w1937:refnum<k5>)  [unwired: 8 in]
            n779 = call "TCP_WriteRead.vi"("error in (no error)"=w1935, "data in"="!firefly:0", "connectin ID in"=w1937) -> ("error out"=w1934:errorcluster)  [unwired: 4 in, 2 out]
          }
        }
        n780 = call <vilib>:"Add State(s) to Queue__JKI_lib_State_Machine.vi"("State(s) in (\"\")"=w1931) -> ("States Out"=w1930:string)  [unwired: 14 in]
      }
      frame "TCP: sendPentero" {
        # "Send Pentero setting to AB computer\n(You can make a copy of, or modify, this frame)"
        n781 = Unbundle By Name(w1940) -> ("System Status.TCP/IP"=w1939:bool)
        n782 = case shown="True" w1939 {
          tunnel: [w1946 w1948] -> w1942
          tunnel: w1941 -> [w1946 w1947]
          frame False {
          }
          frame True {
            n783 = call "TcpIDFGV.vi"("Error In"=w1947, "action"=enum16{"write", "read"}."read") -> ("Error Out"=w1949:errorcluster, "connection ID out"=w1951:refnum<k5>)  [unwired: 8 in]
            n784 = call "TCP_WriteRead.vi"("error in (no error)"=w1949, "data in"="!pentero:0", "connectin ID in"=w1951) -> ("error out"=w1948:errorcluster)  [unwired: 4 in, 2 out]
          }
        }
        n785 = call <vilib>:"Add State(s) to Queue__JKI_lib_State_Machine.vi"("State(s) in (\"\")"=w1945) -> ("States Out"=w1944:string)  [unwired: 14 in]
      }
      frame "TCP: sendChannel" {
        # "Send DeCon Channel to AB computer\n()"
        n786 = Unbundle By Name(w1954) -> ("System Status.TCP/IP"=w1953:bool)
        n787 = case shown="True" w1953 {
          tunnel: [w1960 w1964] -> w1956
          tunnel: w1955 -> [w1960 w1963]
          frame False {
          }
          frame True {
            n788 = local read "DeconChannel"() -> (w1962:i8)
            n789 = case shown="1" w1962 {
              tunnel: ["" ("data in") "!channel:1" ("data in") "!channel:2" ("data in") "!channel:3" ("data in")] -> w1961
              frame 0, Default {
              }
              frame 1 {
              }
              frame 2 {
              }
              frame 3 {
              }
            }
            n790 = call "TcpIDFGV.vi"("Error In"=w1963, "action"=enum16{"write", "read"}."read") -> ("Error Out"=w1965:errorcluster, "connection ID out"=w1966:refnum<k5>)  [unwired: 8 in]
            n791 = call "TCP_WriteRead.vi"("error in (no error)"=w1965, "data in"=w1961, "connectin ID in"=w1966) -> ("error out"=w1964:errorcluster)  [unwired: 4 in, 2 out]
          }
        }
        n792 = call <vilib>:"Add State(s) to Queue__JKI_lib_State_Machine.vi"("State(s) in (\"\")"=w1959) -> ("States Out"=w1958:string)  [unwired: 14 in]
      }
      frame "TCP: startCam" {
        # "Send Pentero setting to AB computer\n(You can make a copy of, or modify, this frame)"
        n793 = Unbundle By Name(w1973) -> ("System Status.TCP/IP"=w1972:bool)
        n794 = case shown="True" w1972 {
          tunnel: [w1979 w1981] -> w1975
          tunnel: w1974 -> [w1979 w1980]
          frame False {
          }
          frame True {
            n795 = call "TcpIDFGV.vi"("Error In"=w1980, "action"=enum16{"write", "read"}."read") -> ("Error Out"=w1982:errorcluster, "connection ID out"=w1984:refnum<k5>)  [unwired: 8 in]
            n796 = call "TCP_WriteRead.vi"("error in (no error)"=w1982, "data in"="!focus:1", "connectin ID in"=w1984) -> ("error out"=w1981:errorcluster)  [unwired: 4 in, 2 out]
          }
        }
        n797 = call <vilib>:"Add State(s) to Queue__JKI_lib_State_Machine.vi"("State(s) in (\"\")"=w1978) -> ("States Out"=w1977:string)  [unwired: 14 in]
      }
      frame "TCP: stopCam" {
        # "Send Pentero setting to AB computer\n(You can make a copy of, or modify, this frame)"
        n798 = Unbundle By Name(w1987) -> ("System Status.TCP/IP"=w1986:bool)
        n799 = case shown="True" w1986 {
          tunnel: [w1993 w1995] -> w1989
          tunnel: w1988 -> [w1993 w1994]
          frame False {
          }
          frame True {
            n800 = call "TcpIDFGV.vi"("Error In"=w1994, "action"=enum16{"write", "read"}."read") -> ("Error Out"=w1996:errorcluster, "connection ID out"=w1998:refnum<k5>)  [unwired: 8 in]
            n801 = call "TCP_WriteRead.vi"("error in (no error)"=w1996, "data in"="!focus:0", "connectin ID in"=w1998) -> ("error out"=w1995:errorcluster)  [unwired: 4 in, 2 out]
          }
        }
        n802 = call <vilib>:"Add State(s) to Queue__JKI_lib_State_Machine.vi"("State(s) in (\"\")"=w1992) -> ("States Out"=w1991:string)  [unwired: 14 in]
      }
      frame "TCP: StartLTLoop" {
        # "reset error"
        # "Start lifetime communication loop\n(You can make a copy of, or modify, this frame)"
        n803 = local write "error (stop LT loop)"(w2000) -> ()
        n804 = Generate User Event(user event=w2003, event data cluster=TRUE ("event data"), error in=w2000) -> (error out=w2001:errorcluster)  [unwired: 1 in, 1 out]
        n805 = call <vilib>:"Add State(s) to Queue__JKI_lib_State_Machine.vi"("State(s) in (\"\")"=w2007) -> ("States Out"=w2006:string)  [unwired: 14 in]
      }
      frame "TCP: StopLTLoop" {
        # "Stop LT communication loop with error\n(You can make a copy of, or modify, this frame)"
        n806 = local write "error (stop LT loop)"(errorcluster {"status"=TRUE, "code"=0, "source"="Stop LT loop"} ("error (stop LT loop)")) -> ()
        n807 = call <vilib>:"Add State(s) to Queue__JKI_lib_State_Machine.vi"("State(s) in (\"\")"=w2013) -> ("States Out"=w2012:string)  [unwired: 14 in]
      }
      frame "TCP: Close" {
        # "Close TCP connection\n()"
        n808 = Unbundle By Name(w2016) -> ("System Status.TCP/IP"=w2014:bool)
        n809 = case shown="True" w2014 {
          tunnel: [w2022 w2024] -> w2017
          tunnel: w2015 -> [w2022 w2023]
          frame False {
          }
          frame True {
            n810 = call "TcpIDFGV.vi"("Error In"=w2023, "action"=enum16{"write", "read"}."read") -> ("Error Out"=w2026:errorcluster, "connection ID out"=w2027:refnum<k5>)  [unwired: 8 in]
            n811 = TCP Close Connection(connection ID=w2027, error in (no error)=w2026) -> (error out=w2024:errorcluster)  [unwired: 1 in, 1 out]
          }
        }
        n812 = case shown="Error .." w2017 {
          tunnel: [w2030 w2031] -> w2018
          tunnel: w2016 -> [w2029 w2031]
          frame No Error {
            w2028 = FALSE ("System Status.TCP/IP")
            n813 = Bundle By Name(cluster=w2029, "System Status.TCP/IP"=w2028) -> (w2030:T15)
            n814 = global write "GlobalVariables.vi" "TCP connected?"(w2028) -> ()
          }
          frame Error {
          }
        }
        n815 = call <vilib>:"Add State(s) to Queue__JKI_lib_State_Machine.vi"("State(s) in (\"\")"=w2021) -> ("States Out"=w2020:string)  [unwired: 14 in]
      }
      frame "---------- Temp ----------" {
        # "Template Separator\n(You can make a copy of, or modify, this frame)"
        n816 = call <vilib>:"Add State(s) to Queue__JKI_lib_State_Machine.vi"("State(s) in (\"\")"=w2036) -> ("States Out"=w2035:string)  [unwired: 14 in]
      }
    }
    n817 = Not(x=w49) -> (.not. x?=w48:bool)
    n818 = local write "ML?"(w48) -> ()
    "ML?" <- TRUE ("main loop running?")
  }
  n819 = while {
    tunnel: w7 -> [w2039]
    tunnel: w1 -> [w2037]
    stop <- w2038 stop-if-true
    n820 = event shown="[1] <StartCommLoop>: User Event" {
      selector: w2039 -> [_ _]
      dyn-events: _ -> [_ _]
      timeout: 30 -> [_ _]
      tunnel: [w2041 _] -> w2038
      tunnel: w2037 -> [w2044 _]
      event Timeout {
        n821 = event-data() -> ()  [unwired: 1 in, 3 out]
        n822 = Get Notifier Status(notifier=w2044) -> (current notification=w2043:bool, error out=w2042:errorcluster)  [unwired: 1 in, 3 out]
        n823 = Or(x=w2043, y=w2042) -> (x .or. y?=w2041:bool)
      }
      event User Event {
        n824 = event-data() -> ()  [unwired: 1 in, 5 out]
        n825 = while {
          shift-right: [w2069] -> _
          shift-left: u32 0 -> [w2070]
          i -> [w2068]
          stop <- w2062 stop-if-true
          # "Send data to AB computer here"
          # "if TCP ip is not open, loop will run once and stop. To re-establish connection and start this loop. Reboot softwrae."
          # "Data communication loop"
          n826 = Tick Count (ms)() -> (millisecond timer value=w2069:u32)
          n827 = Wait (ms)(milliseconds to wait=u32 50) -> ()  [unwired: 1 out]
          n828 = Random Number (0-1)() -> (number: 0 to 1=w2067:dbl)
          n829 = Subtract(x=w2069, y=w2070) -> (x-y=→"Communication loop(ms)":u32)
          n830 = Multiply(x=w2067, y=5.0) -> (x*y=w2065:dbl)
          n831 = Add(x=1.0, y=w2065) -> (x+y=w2060:dbl)
          "Dummy LT Waveform" <- w2060
          n832 = Number To Decimal String(number=w2068) -> (decimal integer string=w2057:string)  [unwired: 1 in]
          n833 = call "TcpIDFGV.vi"("action"=enum16{"write", "read"}."read") -> ("Error Out"=w2047:errorcluster, "connection ID out"=w2055:refnum<k5>)  [unwired: 9 in]
          n834 = Number To Fractional String(number=w2060, precision (6)=i16 2) -> (F-format string=w2049:string)  [unwired: 2 in]
          n835 = Concatenate Strings("!idx:", w2057) -> (w2058:string)
          n836 = Concatenate Strings("!lifetime:", w2049) -> (w2054:string)
          n837 = call "TCP_WriteRead.vi"("error in (no error)"=w2047, "data in"=w2058, "connectin ID in"=w2055) -> ("error out"=w2046:errorcluster, "connectin ID out"=w2056:refnum<k5>)  [unwired: 4 in, 1 out]
          n838 = call "TCP_WriteRead.vi"("error in (no error)"=w2046, "data in"=w2054, "connectin ID in"=w2056) -> ("error out"=w2063:errorcluster, "data out"=→"data out(communcation loop)":string)  [unwired: 4 in, 1 out]
          n839 = Or(x="error (stop LT loop)", y=w2063) -> (x .or. y?=w2062:bool)
        }
      }
    }
  }
  n840 = disable-structure "Diagram Disable Structure" shown="Disabled" {
    frame Disabled {
      w2072 = T28 {"Horizontal"=500, "Vertical"=100}  # Top Left Corner
      n841 = Control Help Window(0:w2072, 1:TRUE ("Show")) -> ()
      n842 = call <vilib>:"TDMS - File Viewer.vi"() -> ()  [unwired: 6 in, 2 out]
    }
    frame Enabled {
    }
  }
  n843 = Unregister For Events(event registration refnum=w35, error in=w13) -> (error out=w3:errorcluster)
  n844 = Release Notifier(notifier=w1, error in (no error)=w3) -> (error out=w2:errorcluster)  [unwired: 1 in, 2 out]
  n845 = Close File(refnum=w23, error in=w2) -> ()  [unwired: 2 out]
